vi "TF+NLH_2Dsweep.vi"() -> ()   [LabVIEW 2022 SP3]
uses:
  <vilib>/Analysis/baseanly.llb/Mean (DBL).vi
  <vilib>/Utility/file.llb/Write Delimited Spreadsheet (DBL).vi
  <vilib>/Analysis/NI_AALBase.lvlib
panel:
  out "Ri_2 phase":cluster{dbl[], dbl[]}(graph)={array[447 elements], [67.2863266033115, 68.42643229574017, 69.17560413533383, 69.48941864427059, 69.72823571868426, 69.93246230369206, 70.1751884099646, 70.29710903847356, 70.39938133386191, 70.53057955170597, 70.54955973974907, 70.65483370602274, 70.71576830766907, 70.74836693865872, 70.76726186359649, 70.82230290925978, 70.874667517587, 70.89353111410381, 70.91524850533594, 70.93619825305268, 70.95863943875658, 71.00402301767619, 71.02562315691524, 71.04364751898778, 71.09155969320202, 71.10466632875095, 71.10472623689654, 71.11327539933023, 71.12212675635854, 71.13448640937536, 71.13707018459343, 71.156029588503, 71.18142789627288, 71.18100597943726, 71.20627888034906, 71.2369698804632, 71.21647578693465, 71.22359731855786, 71.23619623503137, 71.23447865756799, 71.25487976993254, 71.25641101829986, 71.23187433810936, 71.26795744521557, 71.26926560819051, 71.2771926948209, 71.27014833338151, 71.29771757397829, 71.30132174890119, 71.3027753509576, 71.31013562290448, 71.3102375767113, 71.31479459935522, 71.31377012836376, 71.31067966990994, 71.32732871141567, 71.31983842896408, 71.32251344696019, 71.32521523529707, 71.32875354873806, 71.35240329133966, 71.32964637397781, 71.32891425163895, 71.33475814547418, 71.34060930371533, 71.34054473598107, 71.31731968477858, 71.34187116380903, 71.33824813020512, 71.3390204549954, 71.3291558641549, 71.33242973297482, 71.32654001657814, 71.3272617859802, 71.3232175453115, 71.32751642872424, 71.3248015822765, 71.31798187946346, 71.3225081113599, 71.29809468363369, 71.30757005126013, 71.31570116799156, 71.30739843616387, 71.29146920648236, 71.31124170405452, 71.29596584243514, 71.28527922227121, 71.28458810569983, 71.27687551520447, 71.28116342030664, 71.27141850884814, 71.25665249517958, 71.26071027298815, 71.24933212594051, 71.25573024107487, 71.23687214113531, 71.24357647122437, 71.22797873896852, 71.24152814258585, 71.24474907085207, 71.22697381112455, 71.19497244467797, 71.17889791182691, 71.18099382170517, 71.15694947879511, 71.17059403346802, 71.12873981748677, 71.1107641143075, 71.14403706999485, 71.09262969949951, 71.06730520589295, 71.0630662116972, 71.02272879938403, 71.01998987723536, 70.99742600032722, 70.95532207530876, 70.92773951911037, 70.91163496840906, 70.8723642026468, 70.8417266112045, 70.8181277661851, 70.78078830297738, 70.71770772291823, 70.64708869592285, 70.61065891810469, 70.54665253154197, 70.46814601200624, 70.3283370315843, 70.29477028786333, 70.12133548068076, 70.06168917206354, 69.71047188058449, 69.32322258598009, 69.00245607837441, 68.38129382500267, 63.32943082108405, 63.32943082108405]}
  out "Ri_1 phase":cluster{dbl[], dbl[]}(graph)={array[447 elements], [98.64824057353222, 99.17128830231329, 99.1951342832612, 99.00789207290453, 86.10182821595602, -22.857403054638922, 96.84732468296504, 95.16561698897686, 94.41179895625767, 93.19312788552409, 92.23293801802438, 91.48213679635391, 90.86975385450903, 90.08904401111859, 89.56708637967665, 89.05816339184628, 88.51699643736988, 88.00847910591001, 87.55358527129964, 86.9386521072525, 86.32661049392021, 85.97224810625127, 85.4201820241664, 84.76613324411304, 83.98328622688851, 82.62160554286582, 81.65949317710628, 81.06783279665753, 79.92401079184569, 79.42237386116088, 77.70119428653867, 76.70556650622181, 75.87256065512653, 74.17517588749186, 72.53499012614749, 70.99216973171393, 69.3270225882778, 67.65430069310983, 66.10158964613719, 64.57827117039957, 63.36900691986517, 61.856694114558294, 60.5780266856337, 58.9553710362398, 57.66899646954723, 56.46028015883566, 55.18644618742208, 53.89478474582762, 52.86893225941858, 51.90576740532828, 50.815840539479666, 49.83854583648395, 48.98783726797048, 48.20481920257575, 47.14323960132569, 46.56300379926881, 45.8424597787853, 45.104085421320164, 43.98778066206287, 43.55050208439842, 42.823698017347695, 42.208475197083224, 41.75023833211596, 41.006095441554294, 40.42414009253254, 39.92347465699966, 39.3026509483175, 38.70256301313423, 38.39814062530039, 39.08975991819877, 39.69244374540481, 40.39664196446022, 41.06014705097745, 41.5943514568138, 42.34629494787673, 42.80698579826661, 43.43303183920828, 44.19103885752135, 44.94458808485702, 45.81347646789879, 46.337237587140464, 47.157534614289126, 48.026176291338786, 48.910058096664116, 49.821788971793694, 50.620099538298255, 51.49220008891227, 52.576410576076526, 53.43639146612666, 54.795931099898326, 56.02887262919462, 57.22985495493462, 58.39636346943762, 60.06322069434742, 61.59991363454748, 63.227834999494156, 64.75529515969637, 66.40199391928505, 67.89160304574969, 69.41810595275406, 70.61294407010547, 72.26206019073916, 73.96623167454496, 74.87689970747078, 76.00422375609539, 77.31419973762613, 78.31609814928468, 79.07290556369516, 80.20713955144493, 81.345873616141, 82.42155295485148, 83.26995575330962, 84.0578825397184, 84.63979623611135, 85.34509922962876, 85.96512304224451, 86.47660709059683, 87.13813748614467, 87.65181081992219, 88.1985540120427, 88.44105847774664, 89.09342262415899, 89.37635655278324, 90.01954857540177, 90.8783427304726, 91.68597231772134, 92.80218889070814, 93.69238065841928, 95.01075372611008, 95.72905598293364, 71.98501757492694, 98.59740760348397, 98.99419919655249, 99.42747762755556, 99.12811502864284, 104.73224340549825, 118.33929590572768, 118.33929590572768]}
  out "Ri_2":cluster{dbl[], dbl[]}(graph)={array[447 elements], [15988.416286217624, 16728.6647819144, 17222.42749373977, 17463.498507260032, 17721.138199063775, 17863.57717963653, 17945.60163377109, 18070.197068356076, 18166.566932119193, 18199.668814845758, 18277.191037185512, 18350.597939893203, 18361.15003068617, 18538.192909865553, 18450.974040946323, 18496.93935775767, 18509.824502922875, 18528.92733421688, 18537.86973653712, 18247.33592210623, 18948.769873693338, 18615.781885697997, 18640.684401341037, 18645.991010057183, 18662.51527969985, 18677.117982566386, 18686.291050878437, 18723.39732314651, 18716.394342243046, 18745.923698774528, 18742.943040640737, 18753.840717426145, 18775.146084839842, 18775.625740218755, 18793.50624032839, 18791.928638182748, 18789.77689065863, 18803.77679848704, 18818.522370940067, 18811.440317156736, 18828.816055004674, 18833.01121266815, 18836.536471830892, 18842.43162267871, 18845.759082692643, 18855.340959944944, 18860.621985832437, 18874.850438323345, 18867.832627662334, 18873.199676166147, 18874.553160643718, 18877.146479793708, 18879.575606860988, 18890.63600339655, 18899.581042113925, 18907.506617494073, 18916.48206061786, 18918.81920186236, 18914.158596064004, 18938.10837688086, 18914.372066344815, 18923.82303003343, 18929.691680309785, 18941.758817006208, 18940.591605136684, 18976.56467259452, 18972.98156024733, 18965.48790428681, 19192.184240301955, 19190.22161257914, 19184.32494170946, 19192.81728878463, 19180.92951693814, 19179.037679145236, 19182.86767673744, 19178.918568569236, 19201.412480776875, 19341.87490145231, 19045.70581863397, 19204.205684223503, 19196.311769694086, 19199.806156914856, 19198.870165396227, 19206.399452576, 19204.64888696486, 19206.22900198729, 19211.355500785234, 19200.977734814664, 19217.406066104344, 19207.61978640744, 19204.203265191234, 19196.626056963243, 19213.181809880232, 19222.584678372026, 19214.73805057691, 19211.056701580124, 19227.966064572895, 19215.157961719193, 19228.694420225944, 19223.67013231585, 19234.181235717897, 19224.874809867804, 19179.32553225776, 19255.49825519169, 19244.876218524, 19264.41086650312, 19250.059516370784, 19265.408404384434, 19272.545589135265, 19280.416444140265, 19266.700590910965, 19241.253047333794, 19347.160839478965, 19374.179636748766, 19317.46815326459, 19397.194589803166, 19411.40251989236, 19457.002513082487, 19912.691099016047, 19043.806257533153, 19494.748229323617, 19516.780218679087, 19447.240330432873, 19579.68129130049, 19615.446193127405, 19659.245364140435, 19735.448787978745, 19815.406553193978, 19861.803283628833, 20009.699793679596, 20240.011056436713, 20342.30679666903, 20588.65312850611, 21006.842319071144, 21525.00085326132, 20433.789359112274, 20433.789359112274]}
  out "Ri_1":cluster{dbl[], dbl[]}(graph)={array[447 elements], [22045576.2714605, 27293475.908086587, 30763955.208301757, 33265764.692809474, 43359821.082717545, 3155950.3758325954, 33975645.41594882, 32879454.66260026, 31716318.00728969, 31039472.693512905, 29809111.33585218, 28574312.45520694, 27543957.107786126, 26496347.036176518, 25559561.38549122, 24548364.813615683, 23365812.88687177, 22124529.65451581, 21230854.097893827, 20210267.51082642, 19580261.477197297, 18912705.180425838, 18406731.282342993, 17712068.29371939, 17027409.310427506, 16451774.118448615, 15829444.291943796, 15233977.48645753, 14766262.770308785, 14332279.386885434, 13748323.747465877, 13302293.487016145, 12875564.13292509, 12323361.341903234, 11777348.54953025, 11284216.582856042, 10759787.6896821, 10352358.648472596, 9964767.14158643, 9552161.023707548, 9163674.14096663, 8774378.96453125, 8376817.067701741, 8100140.907855841, 7766189.394005965, 7453943.332151328, 7145119.814823653, 6822330.020409241, 6532919.550885053, 6345124.678109345, 6023202.797745062, 5790106.182555463, 5600133.754870802, 5372266.874572496, 5136954.451639774, 4961445.221169122, 4757697.428252076, 4596225.497057631, 4386501.247851164, 4248260.447246732, 4089296.5911337156, 3966429.9201004268, 3832855.939994699, 3717164.6148954397, 3590778.0316126416, 3454130.471709945, 3341234.1590903536, 3265289.764642522, 3297870.0581998965, 3413163.572910136, 3544001.8891905816, 3689443.812705478, 3799303.206259065, 3926721.983737788, 4086964.4365348606, 4206268.0769452825, 4324796.6500504315, 4532717.444204017, 4705136.3930503065, 4875754.054723214, 5071253.457257944, 5303339.599973234, 5481789.417311492, 5728974.215024379, 5943041.275664855, 6174939.548842898, 6419505.835430101, 6696129.679688083, 6980660.096420176, 7328131.387300405, 7608587.58451165, 7931731.115199456, 8263562.874033847, 8695880.524476495, 9124333.086620266, 9537334.492855161, 10001273.51709675, 10434185.413471175, 10904732.657212943, 11384488.704988042, 11790752.952395312, 12375155.659543715, 12874611.660482263, 13299920.063137745, 13680109.511602128, 14152552.783915121, 14646406.058544977, 15242436.55088634, 15838963.722419221, 16488066.171778262, 17189155.40604383, 17874112.959747944, 18505753.66220926, 19199799.29112946, 20082043.340339284, 20849920.713500258, 21637861.109894592, 22530184.096754618, 23696883.713339817, 24704796.36239602, 25871820.156915992, 26994576.58276976, 28599022.488043997, 29553699.907902468, 30925102.81800534, 32120594.843124736, 33923375.76541176, 35108063.55119341, 36833143.39217386, 37366688.458940916, 23545040.53535154, 41067758.729426846, 40939623.20198413, 39560091.29458222, 36752071.88798856, 14862918.294371193, 394331.9556378005, 394331.9556378005]}
  out "Device 2 phase":dbl=67.2863266033115 format="%.3p"
  out "Device 1 phase":dbl=98.64824057353222 format="%.3p"
  out "Ri_2(Ohm)":dbl=15988.416286217624
  out "Ri_1(Ohm)":dbl=22045576.2714605
  out "Device2 Current(mA)":dbl=8.369793490118766e-06
  out "Device1 Current(mA)":dbl=1.295038149901161e-06
  in  "R2(Kohm)":dbl=2.0 format="%#_13g"
  in  "R1(Kohm)":dbl=2.0 format="%#_13g"
  in  "R2 Sensitivity":u16(ring)=26 items=["1 nV/fA", "2 nV/fA", "5 nV/fA", "10 nV/fA", "20 nV/fA", "50 nV/fA", "100 nV/fA", "200 nV/fA", "500 nV/fA", "1 uV/pA", "2 uV/pA", "5 uV/pA", "10 uV/pA", "20 uV/pA", "50 uV/pA", "100 uV/pA", "200 uV/pA", "500 uV/pA", "1 mV/nA", "2 mV/nA", "5 mV/nA", "10 mV/nA", "20 mV/nA", "50 mV/nA", "100 mV/nA", "200 mV/nA", "500 mV/nA", "1 V/uA"]
  in  "R2 Current T Constant":u8(ring)=9 items=["10 us", "30 us", "100 us", "300 us", "1 ms", "3 ms", "10 ms", "30 ms", "100 ms", "300 ms", "1 s", "3 s", "10 s", "30 s", "100 s", "300 s", "1 ks", "3 ks"]
  in  "R1 Current T Constant":u8(ring)=9 items=["10 us", "30 us", "100 us", "300 us", "1 ms", "3 ms", "10 ms", "30 ms", "100 ms", "300 ms", "1 s", "3 s", "10 s", "30 s", "100 s", "300 s", "1 ks", "3 ks"]
  in  "R1 Current sensitivity":u16(ring)=26 items=["1 nV/fA", "2 nV/fA", "5 nV/fA", "10 nV/fA", "20 nV/fA", "50 nV/fA", "100 nV/fA", "200 nV/fA", "500 nV/fA", "1 uV/pA", "2 uV/pA", "5 uV/pA", "10 uV/pA", "20 uV/pA", "50 uV/pA", "100 uV/pA", "200 uV/pA", "500 uV/pA", "1 mV/nA", "2 mV/nA", "5 mV/nA", "10 mV/nA", "20 mV/nA", "50 mV/nA", "100 mV/nA", "200 mV/nA", "500 mV/nA", "1 V/uA"]
  in  "LOCKIN3 address":refnum<visa-resource-name>="COM5"
  in  "Current measurement?":bool=TRUE
  in  "Parameter 1B 1":u16(ring)=2 items=["X", "Y", "R", "Theta", "Frequency", "Noise", "Xh1", "Yh1", "Rh1", "Theta h1", "Xh2", "Yh2", "Rh2", "Theta h2"]
  in  "Phase 1B 1":u16(ring)=3 items=["X", "Y", "R", "Theta", "Frequency", "Noise", "Xh1", "Yh1", "Rh1", "Theta h1", "Xh2", "Yh2", "Rh2", "Theta h2"]
  out "Vab_1(1w)/mV":dbl=69.89491300035615
  out "phase Vab_1":dbl=90.88973926590094
  out "Vab_1/mV":cluster{dbl[], dbl[]}(graph)={array[447 elements], [69.89491300035615, 96.76091439179595, 121.60820325078673, 144.86984014112141, 167.73987501255314, 189.85333845062206, 212.76412267080005, 234.14803223340567, 254.28955060290502, 272.7317853345533, 289.83246203860267, 305.5450081707562, 320.16279403993354, 334.0773405165712, 347.02580142204937, 359.09399104540176, 372.23679318705814, 381.71894566566425, 396.5690488528649, 406.940835102248, 415.4777292621394, 424.8569017583363, 432.7538730200402, 440.00812513863, 448.52637063152594, 456.85237908909124, 464.137670276543, 472.2262412823993, 479.92842889273936, 487.6190417996467, 496.3166214468891, 503.07011002512405, 508.8219837590173, 517.1519063185144, 525.7953306380335, 539.3627686357203, 541.3617410482888, 548.5971674541836, 556.374844313196, 563.6069775945068, 571.8031649261083, 580.495799665217, 586.3877145229121, 593.8940166229253, 600.721090651385, 607.6895159228869, 614.1735521509668, 621.3512268861805, 628.0638510684262, 636.9440825992266, 642.589550225185, 649.9335791143177, 656.2448134788818, 663.9368277053549, 670.7937070923226, 678.5695123765853, 686.3987854950642, 694.5732517890214, 699.7779564487922, 705.685059941211, 713.0262385771273, 720.1108156834745, 729.569007775922, 735.0544079957034, 740.576008333156, 748.092243959333, 756.9633362654706, 760.2650973137223, 770.0898646046744, 763.2754854059085, 758.3002322895187, 746.9705677890544, 742.0331175764676, 735.46121484323, 727.7172172859215, 720.7173158772874, 712.99169073752, 707.050271699919, 699.916135108249, 694.4541828796475, 687.007963984917, 680.182322092647, 671.6050750240062, 665.5686279746279, 659.08553222554, 653.6017948895201, 646.4809963945931, 639.403394643278, 630.3579752688884, 623.5181112871613, 616.8554923220863, 610.6099012812795, 603.2215573569297, 595.4709115032604, 585.447913504759, 577.6229779091719, 570.5976464085383, 563.4007691158172, 555.4873986901947, 548.6413839458369, 540.585411112968, 532.6016369667757, 526.2399667657975, 518.0081516009911, 511.03829248244693, 502.0670977041706, 494.5727702095127, 488.0329979874539, 478.84273975168026, 471.69952058379425, 464.6428266619654, 455.7501857674969, 447.6210647470701, 440.1493478794361, 431.08806792417124, 421.6336738249846, 411.80987033576866, 403.49332406392034, 393.617268025408, 383.21282480148824, 372.20708655208506, 360.5170780717179, 348.99573641712726, 336.0751062717885, 322.3016839152484, 307.1083537103844, 290.94530748218335, 273.55902036869213, 254.4926943267793, 234.28942783781397, 212.9781220107684, 187.86427671847667, 165.2636595766354, 142.77665596194007, 119.793615425549, 95.38271597000687, 0.09538271597000687]}
  out "phase Vab_1":cluster{dbl[], dbl[]}(graph)={array[447 elements], [90.88973926590094, 90.52797326935718, 90.24221168935227, 90.05619331418181, 89.82402670735155, 89.43475667628768, 88.97990454089964, 88.44396332463643, 87.96488659679174, 87.42119770073006, 86.92388263342272, 86.48364998536113, 85.99122029778825, 85.57113746974912, 85.1737392935055, 84.84429176826526, 84.61648244558981, 84.39863700541643, 84.39047173551977, 84.31040018808953, 84.28616173042795, 84.27963444410904, 84.29052508971986, 84.35337905461374, 84.48798685578761, 84.6334468365483, 84.84938888426412, 85.05553183037861, 85.2218152401819, 85.40541095682514, 85.66046178789543, 85.90545188370128, 86.13216922565734, 86.38265558116399, 86.65406276846046, 86.91253207804952, 87.18486426305384, 87.42816773898326, 87.63158481854084, 87.86233637683861, 88.13407094246728, 88.27976493605578, 88.57655203525272, 88.82933322275144, 89.06438112269504, 89.29707773628597, 89.50407685721082, 89.74107738483386, 89.89143188530203, 90.06691792993078, 90.3103543154843, 90.46367936659934, 90.6387057493134, 90.82986512108896, 91.01674618887878, 91.09084887196157, 91.27133334734977, 91.40474871037804, 91.52644294089797, 91.67243711695147, 91.77582850460796, 91.93779407688712, 91.96007834595751, 92.15572215870259, 92.29971314770144, 92.3387174294799, 92.42238251137285, 92.62272966378458, 92.59121603701458, 92.52667962397057, 92.37812039104159, 92.41197917214927, 92.25218709944694, 92.13367167192551, 92.04888515402025, 91.9110871959863, 91.79252598732182, 91.60650423258802, 91.59890708517739, 91.40387946715751, 91.21488009806522, 91.11358490554794, 90.99524149204582, 90.79975373157988, 90.62251592150207, 90.45192948011531, 90.27266294152018, 90.08071301381186, 89.92199803936612, 89.66090401141147, 89.48436778178451, 89.24229483637853, 88.99995082200304, 88.80450846419185, 88.63063132266655, 88.3773911659327, 88.11024296250065, 87.90048336420998, 87.63874656677974, 87.40922433762555, 87.15146501518254, 86.86078212535051, 86.6538901112055, 86.41540121139467, 86.20189760315316, 85.9426657982776, 85.690292850898, 85.43151419868113, 85.2197061571944, 85.01429203463259, 84.84078565202971, 84.65834064339072, 84.50978131286871, 84.38968861773391, 84.27730864450257, 84.19167192359482, 84.15599911428015, 84.24936497822945, 84.29514042933667, 84.4229792596429, 84.61642660479922, 84.87595078760202, 85.23931108593368, 85.62649020269703, 86.06934732659286, 86.55060906452294, 87.03428962580335, 87.51819781702497, 88.06917931477217, 88.5245583671414, 88.98978203472014, 89.44122721966406, 89.75358671473366, 90.00839348446064, 90.21871142933574, 90.46727689558784, 90.46727689558784]}
  out "Vab_2(1w)/mV":dbl=0.05504782589540923
  in  "Parameter 2B 1":u16(ring)=2 items=["X", "Y", "R", "Theta", "Frequency", "Noise", "Xh1", "Yh1", "Rh1", "Theta h1", "Xh2", "Yh2", "Rh2", "Theta h2"]
  in  "Phase 2B 1":u16(ring)=3 items=["X", "Y", "R", "Theta", "Frequency", "Noise", "Xh1", "Yh1", "Rh1", "Theta h1", "Xh2", "Yh2", "Rh2", "Theta h2"]
  out "Vab_2/mV":cluster{dbl[], dbl[]}(graph)={array[447 elements], [0.05504782589540923, 0.08174963900387706, 0.1086491390142213, 0.1350953352313944, 0.16199632000588896, 0.18871077141583378, 0.21540521495658613, 0.24212435453052203, 0.26890247886877494, 0.29552482456320167, 0.32258570821668, 0.3494042559717882, 0.37594130906440903, 0.40415399166191385, 0.4297877956839886, 0.4565469885788846, 0.4834868719058818, 0.5099801395541058, 0.5365898114212174, 0.5650196727768638, 0.6153224681040677, 0.6167753495606371, 0.6433511284852396, 0.6698553439971563, 0.6963334815374641, 0.72306249630336, 0.7498661407570503, 0.777540387307819, 0.8039872881129053, 0.8306848892073286, 0.8565751828914451, 0.8836807612900971, 0.9105318047943302, 0.936516650845644, 0.9636848031511576, 0.9900174496688153, 1.0155067100535131, 1.0429079201232776, 1.069429262326823, 1.0956882570263036, 1.1222110190156476, 1.148795646772743, 1.1753327010150363, 1.2019263533143982, 1.228381719823452, 1.2545475198538012, 1.2812633241442646, 1.3070782706694737, 1.333608439591284, 1.3600906687552823, 1.3862774538793732, 1.412061455838872, 1.4389670903805294, 1.4651948591598645, 1.4908718427837173, 1.518015543331282, 1.545769299778577, 1.572154931730819, 1.5985003001796778, 1.6233111449201556, 1.6484992142095583, 1.6747983901681438, 1.7020924335968, 1.7287579367019952, 1.7559499387410313, 1.782575600183194, 1.8090046681914527, 1.8359466301397063, 1.8586719383176984, 1.8319060664677964, 1.8059980427635538, 1.7796862395299262, 1.7514192762034468, 1.7244809548743052, 1.6983410974939976, 1.6718938419879956, 1.6462121209020237, 1.6195000852062709, 1.5674352448786275, 1.5688527907635799, 1.5421352110091182, 1.5166894409291403, 1.4901521893311171, 1.463685618446582, 1.4371269782596554, 1.4108838829627208, 1.3845821412725943, 1.3582753758079424, 1.3321639978967672, 1.3046348516956425, 1.2784296961198498, 1.251377246196452, 1.2257446823466882, 1.199624176714759, 1.1726915378017204, 1.1462270638572194, 1.11975842382519, 1.0933051178522766, 1.0670212956767868, 1.0400481080390023, 1.0136730950163222, 0.9865872713125264, 0.9595089165754551, 0.9333819228541328, 0.9067272830452382, 0.8800918508692932, 0.8531109540697044, 0.8272638966110974, 0.8002139272602338, 0.77334067720438, 0.7464596577055119, 0.720085145608187, 0.6941845834379488, 0.6705341882933702, 0.6438603276504212, 0.617016475397683, 0.5899056969248984, 0.5631586418589446, 0.535158502041674, 0.4850978602391158, 0.48255405943119034, 0.4553320577540521, 0.42723377189680495, 0.4011445572614489, 0.3744925824568009, 0.3473094083332051, 0.32092465247254065, 0.2938313088100053, 0.2671169874808368, 0.2403177493052949, 0.21367423121897425, 0.18666841954924793, 0.1596474534235999, 0.13259816185629864, 0.10564756137259422, 0.10564756137259422]}
  out "phase Vab_2":dbl=89.98636954382417
  out "phase Vab_2":cluster{dbl[], dbl[]}(graph)={array[447 elements], [89.98636954382417, 90.03967319419863, 90.0401476465123, 89.99776761885384, 90.0222418709453, 90.01526903166591, 90.02869426514728, 90.01475132450953, 90.02160015273246, 90.03106270083825, 90.03582546833678, 90.03257710652228, 90.02612755809257, 90.02777418011617, 90.02881201881874, 90.02603115955061, 90.03387858321058, 90.02423111026776, 90.0298329743401, 90.0199101721892, 90.02008626238324, 90.01905833125883, 90.0226624250662, 90.01524219410577, 90.01064477190369, 90.01314320313155, 90.00964441150451, 90.007480576353, 90.00751384955382, 90.00568040647654, 90.00225023080912, 90.00179313839485, 89.9943445053494, 89.99638341896197, 89.99107879178376, 89.99070351224353, 89.98795446635322, 89.98662682800266, 89.98255898571668, 89.97950944534594, 89.97885050000609, 89.98001159100461, 89.97638179460355, 89.97397388097008, 89.97386998434929, 89.97190686780083, 89.96964943942537, 89.96652965395793, 89.96664790872887, 89.9651967818322, 89.96328286683708, 89.96390175771866, 89.9603252973263, 89.95814083102191, 89.95867001681638, 89.95859246077052, 89.9599408176306, 89.9554627877762, 89.9563396626164, 89.9542344080695, 89.9537832379153, 89.95103282620559, 89.95050590087968, 89.95106030902204, 89.95264289581421, 89.95158819964809, 89.95041962543326, 89.94974338020069, 89.94997443777854, 89.95170075918911, 89.95247909300647, 89.95180399748936, 89.94841578255253, 89.9503050525758, 89.95385182971656, 89.95377247032924, 89.95406599067066, 89.96047202514728, 89.95820512566924, 89.95880560309685, 89.95764180403465, 89.96186623373474, 89.96308076069838, 89.96241158857234, 89.96358286171663, 89.96555096814687, 89.96414990686654, 89.96805952212296, 89.96805956444439, 89.96842578734393, 89.97234710687766, 89.97321477774166, 89.97532264688338, 89.97725566537538, 89.98119721498324, 89.97774793328412, 89.98176413337141, 89.9856479020747, 89.98484345999856, 89.98795891683308, 89.98813178811233, 89.98795432168693, 89.98952215489766, 89.99420384702498, 89.99647060182336, 89.99526917518443, 89.99933379690103, 90.00609885406311, 90.00482328009898, 90.00861804999309, 90.01263720244857, 90.01011885735718, 90.01426821869731, 90.01434477063428, 90.02407380002145, 90.01888273544807, 90.02104556140974, 90.02226692616459, 90.0184250982925, 90.02624472279317, 90.03191794705317, 90.02551643212949, 90.02854738363274, 90.02816141702668, 90.02924202432983, 90.0225129073069, 90.03393763571692, 90.02461542837548, 90.02201842331168, 90.02883400042535, 90.0149527060912, 90.03276532522105, 90.03417556063343, 90.00596720794834, 89.99433316143694, 89.99433316143694]}
  out "Phase2A-F":cluster{dbl[], dbl[]}(graph)={[0.1], [0.0]}
  out "R2A-F":cluster{dbl[], dbl[]}(graph)={[0.1], [0.0]}
  out "Phase2B-F":cluster{dbl[], dbl[]}(graph)
  out "R2B-F":cluster{dbl[], dbl[]}(graph)={[0.1], [0.0]}
  out "phase 2B 2":dbl
  in  "Phase 2B 2":u16(ring)=9 items=["X", "Y", "R", "Theta", "Frequency", "Noise", "Xh1", "Yh1", "Rh1", "Theta h1", "Xh2", "Yh2", "Rh2", "Theta h2"]
  out "phase 2A 2":dbl
  in  "Phase 2A  2":u16(ring)=3 items=["X", "Y", "R", "Theta", "Frequency", "Noise", "Xh1", "Yh1", "Rh1", "Theta h1", "Xh2", "Yh2", "Rh2", "Theta h2"]
  out "para2A Measurement 2":dbl
  in  "F Clear Plot 2A":bool
  in  "Parameter 2A 2":u16(ring)=2 items=["X", "Y", "R", "Theta", "Frequency", "Noise", "Xh1", "Yh1", "Rh1", "Theta h1", "Xh2", "Yh2", "Rh2", "Theta h2"]
  out "para2B Measurement 2":dbl
  in  "F Clear Plot 2B":bool
  in  "Parameter 2B 2":u16(ring)=8 items=["X", "Y", "R", "Theta", "Frequency", "Noise", "Xh1", "Yh1", "Rh1", "Theta h1", "Xh2", "Yh2", "Rh2", "Theta h2"]
  out "Phase1A-F":cluster{dbl[], dbl[]}(graph)
  out "R1A-F":cluster{dbl[], dbl[]}(graph)
  out "Phase1B-F":cluster{dbl[], dbl[]}(graph)
  out "R1B-F":cluster{dbl[], dbl[]}(graph)
  out "phase 1B 2":dbl
  in  "Phase 1B 2":u16(ring)=9 items=["X", "Y", "R", "Theta", "Frequency", "Noise", "Xh1", "Yh1", "Rh1", "Theta h1", "Xh2", "Yh2", "Rh2", "Theta h2"]
  out "phase 1A 2":dbl
  in  "Phase 1A 2":u16(ring)=3 items=["X", "Y", "R", "Theta", "Frequency", "Noise", "Xh1", "Yh1", "Rh1", "Theta h1", "Xh2", "Yh2", "Rh2", "Theta h2"]
  out "para1A Measurement (mV) 2":dbl=1.49013e-07
  in  "F Clear Plot 1A":bool
  in  "Parameter 1A 2":u16(ring)=2 items=["X", "Y", "R", "Theta", "Frequency", "Noise", "Xh1", "Yh1", "Rh1", "Theta h1", "Xh2", "Yh2", "Rh2", "Theta h2"]
  out "para1B Measurement (uV) 2":dbl=1.49013e-07
  in  "F Clear Plot 1B":bool
  in  "Parameter 1B 2":u16(ring)=8 items=["X", "Y", "R", "Theta", "Frequency", "Noise", "Xh1", "Yh1", "Rh1", "Theta h1", "Xh2", "Yh2", "Rh2", "Theta h2"]
  in  "path2 (folder + filename)":string="H:\\My Drive\\Lab\\Opticool\\Measurement\\NLH\\T dependence\\TaI27_A1016_B1516_test"
  out "phase Vaa_1":cluster{dbl[], dbl[]}(graph)={array[447 elements], [-90.0, -90.0, -90.0, -90.0, -90.0, -90.0, -90.0, -90.0, -90.0, -90.0, -90.0, -90.0, -90.0, -90.0, -90.0, -90.0, -90.0, -90.0, -90.0, -90.0, -90.0, -90.0, -90.0, -90.0, -90.0, -90.0, -90.0, -90.0, -90.0, -90.0, -90.0, -90.0, -90.0, -90.0, -90.0, -90.0, -90.0, -90.0, -90.0, -90.0, -90.0, -90.0, -90.0, -90.0, -90.0, -90.0, -90.0, -90.0, -90.0, -90.0, -90.0, -90.0, -90.0, -90.0, -90.0, -90.0, -90.0, -90.0, -90.0, -90.0, -90.0, -90.0, -90.0, -90.0, -90.0, -90.0, -90.0, -90.0, -90.0, -90.0, -90.0, -90.0, -90.0, -90.0, -90.0, -90.0, -90.0, -90.0, -90.0, -90.0, -90.0, -90.0, -90.0, -90.0, -90.0, -90.0, -90.0, -90.0, -90.0, -90.0, -90.0, -90.0, -90.0, -90.0, -90.0, -90.0, -90.0, -90.0, -90.0, -90.0, -90.0, -90.0, -90.0, -90.0, -90.0, -90.0, -90.0, -90.0, -90.0, -90.0, -90.0, -90.0, -90.0, -90.0, -90.0, -90.0, -90.0, -90.0, -90.0, -90.0, -90.0, -90.0, -90.0, -90.0, -90.0, -90.0, -90.0, -90.0, -90.0, -90.0, -90.0, -90.0, -90.0, -90.0, -90.0, -90.0, -90.0, -90.0]}
  out "Vaa_1/mV":cluster{dbl[], dbl[]}(graph)={array[447 elements], [28.54986230809714, 47.90602322555852, 69.13880402618318, 91.74088027854695, 116.09423060900622, 126.29292594886878, 152.34333138764072, 170.38941026837637, 188.72717003139223, 207.09670879518862, 223.27714792302223, 239.09530915982268, 253.96866223624244, 268.10055850834317, 284.1930208945555, 296.9400604656871, 306.8418650583954, 314.71077986113585, 324.8096514364511, 334.45516719840055, 345.2751932124764, 355.7157880621078, 366.8537803090993, 375.6147659337272, 382.6007505803814, 393.47724926935217, 400.49050064772996, 407.5485504924969, 413.6432604376539, 420.8265461237909, 426.6173764310682, 433.635430137789, 442.5451386667651, 446.83506923110616, 449.41691810343707, 455.1160806660415, 459.5157780704797, 464.5304454573484, 471.2973043505908, 475.2198625165156, 479.07227226723137, 482.9178917074458, 486.22088193879244, 495.09103303765596, 499.324083426905, 504.20168302074853, 509.45597042076264, 512.0104443681062, 513.8593456505303, 521.857561920325, 521.7846572347574, 524.8188626940346, 530.7443300930335, 532.2284129403052, 536.4970249271563, 538.859316009316, 541.4792257221472, 546.466260110555, 551.0869260849482, 552.4833138837979, 555.8760860627742, 557.6075820251485, 559.767692284389, 565.4670612075352, 567.1402355116674, 568.4045720496342, 571.3865971710253, 578.6325276470443, 576.7201061295497, 571.1883361841326, 570.4182884439209, 569.461761245208, 565.2512639499868, 562.3052339123483, 560.6884611622394, 558.9193285846687, 553.1436266827282, 551.5932911338228, 548.635799671936, 542.1674835477035, 541.0172163291315, 539.914220429268, 533.6419081222197, 531.0176781462837, 525.3084038907192, 522.7943427328461, 518.5380642635973, 515.8961486976631, 514.2733852885369, 509.72759631064423, 503.9501781756484, 499.2678347371449, 496.40962237161796, 491.80635505697677, 490.4617117070987, 485.1742271220353, 482.0446129719921, 475.9996837404127, 472.6782621100959, 468.2971762724189, 462.1864679849175, 458.47754471745617, 450.5194671600685, 445.05833394151387, 437.3036576834162, 429.75676530040477, 422.2152681826013, 416.86776209046945, 410.4010237044718, 403.16700771496164, 396.8216458438753, 388.49299645581715, 380.56332239470265, 372.3807562243823, 361.6392938119466, 355.2142501054603, 344.4659622791879, 333.32240957381543, 323.4493356975189, 312.13865046326316, 300.50315760800555, 286.86993382755776, 275.8465837513604, 258.6568970790021, 241.15871978639944, 227.792037293373, 211.3465846844987, 195.5210307298651, 179.12175652769412, 160.0385725885352, 150.4506723637251, 123.84923542089372, 103.1763424845562, 80.07139246418663, 57.276443385142485, 36.166077095315934, 17.42622501409195, 17.42622501409195]}
  out "Phase1B-T":cluster{dbl[], dbl[]}(graph)={array[447 elements], [-0.0428368767358694, 0.019425738673648576, 0.06601336294885965, 0.12751390529792714, 0.21891328703140842, 0.2139600423089886, 0.3202891373518463, 0.5653445808746654, 0.8962538707982652, 1.2571346321505499, 1.606301670176481, 1.9056143928649256, 1.991351868000408, 1.988260247302692, 1.755701270770857, 1.4150419758773847, 0.9666181709825361, 0.4781661851611167, 0.07786977428258289, -0.31921775054521556, -0.5319269967389744, -0.917697368480033, -1.416396561722631, -1.6500153972582816, -1.9572642672945826, -2.2544114467295797, -2.162541178826363, -2.378638843933177, -2.7944233559771234, -2.9522321795232656, -3.073536918287995, -3.1242675115899687, -3.0838196681594883, -3.5508253393225524, -3.8243520103554154, -3.9039948394823236, -3.705890346352678, -4.021095031312841, -4.142208186339788, -4.557849167991822, -4.69334843822529, -4.98064985720908, -5.141308179691781, -5.597455016446071, -5.6045044083128195, -5.890565984116882, -6.487479059224005, -6.648445444092485, -6.7025474266406535, -6.807549291485394, -6.890715596724121, -6.670677922609039, -7.1779161834435525, -7.397104646423365, -7.725977915533429, -9.028821811181647, -9.625827157282213, -10.551010326623167, -10.140345055790643, -9.719127290466453, -9.455249331621122, -9.002043477711032, -8.812633517143642, -8.001995584354216, -6.796618229609791, -6.506804750288498, -5.384613593618006, -4.999091183121753, -4.671119395457472, -4.995028651891374, -5.163198702989056, -5.2275892583156764, -5.553112626699551, -5.742012236238783, -6.002884347788617, -6.34951264021017, -6.501343380041442, -6.996016601650247, -6.885713785862563, -6.808189214852123, -6.891739474989711, -6.414914544932198, -6.6107298401261305, -6.666545643649042, -6.669317377611124, -6.803630786969256, -6.687625686618477, -6.229020650697875, -6.5754921415814, -6.434215291472372, -6.178441867090024, -6.148668612211155, -5.855063552961937, -5.641145351326709, -5.407002479193986, -5.175085704554695, -4.984151429330852, -4.740938590426882, -4.393567047411585, -4.125555149902717, -3.9232596961522432, -3.58122053632991, -3.55297978358587, -3.012480741093095, -2.961273786915813, -2.17265758603968, -2.0218915507952593, -1.872085515945707, -1.6814909435522, -1.5599782037249579, -1.4112374104641112, -1.2382170209936327, -1.0671702138186363, -0.740217543128334, -0.6352820647843831, -0.36943879373102734, -0.16661703603105704, -0.02775688194834209, 0.12209464743594815, 0.27578697463604673, 0.44353680360386927, 0.5855139758919539, 0.6691109238405835, 0.7293740437580607, 0.7454861201352151, 0.7097541743895233, 0.6348587589201704, 0.5050228954104379, 0.3837962630215416, 0.23928951289350775, 0.4048700099789791, 0.2969667660401464, 0.2419093507799051, 0.15724973554986582, 0.07803063399563674, 0.03971435353920284, 0.03971435353920284]}
  out "R1B-T":cluster{dbl[], dbl[]}(graph)={array[447 elements], [156653.03630696764, 148669.35859716916, 140750.0698084012, 132895.51710122655, 125358.74665741803, 117251.34041918642, 110126.05537967787, 104032.3796825124, 98694.84438965151, 93627.06160482153, 88874.08330738443, 84651.96247295255, 80655.62889130137, 77353.36648383504, 74364.1231804382, 71537.43674065488, 69358.97439512891, 67633.51892577752, 66810.86995199334, 66456.55828298542, 66096.12665938094, 65862.08981586057, 65831.94755910935, 65938.78834732961, 66064.27762077464, 65323.83051235899, 64939.17778834897, 64592.35089393325, 64320.54559203627, 63927.50238148678, 63685.4736398772, 62952.941632842456, 61863.71621556276, 60968.37722476152, 60230.47573671074, 60493.40833415097, 60188.09201001243, 59886.193502477945, 59665.2220993736, 59463.7849048051, 59499.745510583736, 59594.69145722589, 59646.58712569106, 59775.211553687855, 59922.61732820779, 60037.32436687335, 59796.209859831164, 59396.04823648047, 59077.798079345455, 59005.77481987122, 58899.62037777882, 58549.59949712524, 57296.55847069468, 55185.31877347994, 52434.76696388336, 49244.170987330435, 45614.190254019355, 42447.2433009042, 40166.66109099554, 39992.14976412257, 40580.392421616554, 41558.88836278036, 43693.48991513804, 46625.649281395774, 49688.994850098374, 53044.280697961374, 55723.281474167954, 57636.31181556067, 57615.52406975564, 57520.638046988526, 57448.45745580508, 57767.61595961488, 57652.01666564756, 57527.643047949015, 57548.26764858691, 58046.55680219043, 58688.139202819584, 59519.35386512262, 60156.35189802062, 60345.93454513358, 60854.62397351101, 61566.06525510755, 62715.45636752421, 63851.76867791205, 64485.88190095292, 64583.8900715666, 64614.7318290972, 64616.22804455587, 65019.35744354623, 65159.95720882481, 65238.57114716061, 65026.68356980856, 64746.407251066936, 64664.484449826756, 64999.380726995165, 65462.789162605935, 65755.6101803984, 66133.51813389454, 66634.81383937939, 67166.7870458519, 68036.55322059919, 69027.86485769883, 70048.14565665925, 71368.20869162361, 72949.53106005031, 74835.45795357773, 76722.40627798814, 79199.53379772593, 82330.04244523244, 85827.64570941599, 89933.38874289654, 94673.33307932099, 100195.65823507162, 106491.45500187187, 113728.49713083068, 121616.58437941017, 130081.97029892445, 138723.70753480514, 148021.39689669872, 157968.65499305708, 167699.95173412305, 177664.07084666408, 184374.81286493735, 189183.163541887, 191512.30730552098, 191188.05610214468, 187927.49166520472, 180376.339012124, 168716.50294927045, 154922.70062195673, 138205.33167340915, 121320.09824131276, 104575.51507388374, 88622.86788988147, 75489.54929101207, 68245.72466796775, 68245.72466796775]}
  out "phase 1B":dbl=-0.0428368767358694
  in  "Phase 1B":u16(ring)=9 items=["X", "Y", "R", "Theta", "Frequency", "Noise", "Xh1", "Yh1", "Rh1", "Theta h1", "Xh2", "Yh2", "Rh2", "Theta h2"]
  out "phase Vaa_1":dbl=-90.0
  in  "Phase 1A":u16(ring)=3 items=["X", "Y", "R", "Theta", "Frequency", "Noise", "Xh1", "Yh1", "Rh1", "Theta h1", "Xh2", "Yh2", "Rh2", "Theta h2"]
  out "Vaa_1(1w)/mV":dbl=28.54986230809714
  in  "T Clear Plot 1A":bool
  in  "Parameter 1A":u16(ring)=2 items=["X", "Y", "R", "Theta", "Frequency", "Noise", "Xh1", "Yh1", "Rh1", "Theta h1", "Xh2", "Yh2", "Rh2", "Theta h2"]
  out "para1B Measurement":dbl=156653.03630696764
  in  "T Clear Plot 1B":bool
  in  "Parameter 1B":u16(ring)=8 items=["X", "Y", "R", "Theta", "Frequency", "Noise", "Xh1", "Yh1", "Rh1", "Theta h1", "Xh2", "Yh2", "Rh2", "Theta h2"]
  out "phase Vaa_2":cluster{dbl[], dbl[]}(graph)={array[447 elements], [90.0, 90.0, 90.0, 90.0, 90.0, 90.0, 90.0, 90.0, 90.0, 90.0, 90.0, 90.0, 90.0, 90.0, 90.0, 90.0, 90.0, 90.0, 90.0, 90.0, 90.0, 90.0, 90.0, 90.0, 90.0, 90.0, 90.0, 90.0, 90.0, 90.0, 90.0, 90.0, 90.0, 90.0, 90.0, 90.0, 90.0, 90.0, 90.0, 90.0, 90.0, 90.0, 90.0, 90.0, 90.0, 90.0, 90.0, 90.0, 90.0, 90.0, 90.0, 90.0, 90.0, 90.0, 90.0, 90.0, 90.0, 90.0, 90.0, 90.0, 90.0, 90.0, 90.0, 90.0, 90.0, 90.0, 90.0, 90.0, 90.0, 90.0, 90.0, 90.0, 90.0, 90.0, 90.0, 90.0, 90.0, 90.0, 90.0, 90.0, 90.0, 90.0, 90.0, 90.0, 90.0, 90.0, 90.0, 90.0, 90.0, 90.0, 90.0, 90.0, 90.0, 90.0, 90.0, 90.0, 90.0, 90.0, 90.0, 90.0, 90.0, 90.0, 90.0, 90.0, 90.0, 90.0, 90.0, 90.0, 90.0, 90.0, 90.0, 90.0, 90.0, 90.0, 90.0, 90.0, 90.0, 90.0, 90.0, 90.0, 90.0, 90.0, 90.0, 90.0, 90.0, 90.0, 90.0, 90.0, 90.0, 90.0, 90.0, 90.0, 90.0, 90.0, 90.0, 90.0]}
  out "Vaa_2/mV":cluster{dbl[], dbl[]}(graph)={array[447 elements], [0.13381974254969312, 0.18742714557336168, 0.24193630688555348, 0.2935892785474931, 0.3479241671469837, 0.40180896386790493, 0.45368862257203035, 0.5082025450648269, 0.5617588973183396, 0.6130105235675594, 0.6681572310006635, 0.7227895287602891, 0.7736466036357633, 0.8335500758536397, 0.8815480547811793, 0.9357109191098203, 0.9875782277032862, 1.040868809441492, 1.095090897331736, 1.1747106159712257, 1.226856272234, 1.2540223708132843, 1.308791730226083, 1.3601778715290997, 1.4144756362080564, 1.4669111879869992, 1.5198122641709386, 1.5763564964287788, 1.627258918430943, 1.6829610709942446, 1.7347039042428267, 1.787131627051539, 1.842990828060025, 1.8948913764748603, 1.9499228164526228, 2.0017844440101387, 2.0532826238944915, 2.109197084129517, 2.1629586294805323, 2.2144151171419972, 2.2692987490718153, 2.322005989452896, 2.3740937894622642, 2.4282075783401544, 2.48027388623933, 2.5346829265701496, 2.5886897937084234, 2.643246419254771, 2.693911762161861, 2.748627308177585, 2.801110037277913, 2.8529923664874692, 2.9056809189103614, 2.9607146118620182, 3.015233207723972, 3.068486923290655, 3.1234203943636327, 3.1755679448464025, 3.2287947853467114, 3.284263127783291, 3.333983892472329, 3.3877660463472044, 3.4425367018738493, 3.4976986613730205, 3.5487949460745205, 3.609858553422258, 3.6611429843509202, 3.710602935938376, 3.707057741181432, 3.652440365901994, 3.598528318933693, 3.547133036416897, 3.491914000109365, 3.436654890996338, 3.38373777826206, 3.3289956981589874, 3.279244940684171, 3.1929766105427855, 3.144399429486219, 3.1199998023843234, 3.064956277223548, 3.011777093344942, 2.958733588137276, 2.9073826220408523, 2.8529486049233252, 2.799604745203765, 2.7462382732359663, 2.6907286153414556, 2.6399129053163444, 2.5839375773906603, 2.529941329570786, 2.475965439824034, 2.4253889243156443, 2.37271574046373, 2.317295557052546, 2.2642061200665595, 2.2125103836347613, 2.1562554502299545, 2.1051508641724936, 2.050677472623137, 1.9979216366039663, 1.942572819238161, 1.8854172013620933, 1.8394191546832923, 1.7839892210108856, 1.7305228805087955, 1.6757577630299372, 1.6246239862471612, 1.5719471607187463, 1.517782524650135, 1.46244227108224, 1.4077807390939265, 1.3609587826472371, 1.307813032382216, 1.2515421511312934, 1.2020571451792048, 1.1476637017173545, 1.095545763835169, 1.0179772081249736, 0.9631381585880434, 0.9334695619404194, 0.8794155178512697, 0.8227043347953057, 0.7727602458939524, 0.7184672676003201, 0.6655627507727929, 0.6135075057219885, 0.5601076930051849, 0.5050556179993441, 0.4543692162049564, 0.40185237548020547, 0.34633302986717796, 0.2909740598878531, 0.23867838334778513, 0.18388695194469842, 0.18388695194469842]}
  out "Phase2B-T":cluster{dbl[], dbl[]}(graph)={array[447 elements], [-0.03469454178376795, -0.00736809463286604, -0.022964586979785772, -0.029719841307236955, -0.012534923664164779, -0.024046608840346307, -0.022023733182412193, -0.03259843425226211, 0.009789315130899187, -0.019231697327260287, -0.00197076413704439, -0.0009456659113533516, 0.021598458359082032, -0.00413298679003386, 0.011347317585862665, -0.005489815159564186, -0.0014322184820076947, 0.008701249063545564, -0.0007863262108556386, 0.040937815111443836, 0.014917465084632426, 0.016230414199592022, 0.015825143776374527, -0.004238768141281416, -0.01051382589652682, 0.009920733281610564, 0.010710247783674309, 0.023230377031032846, 0.017171097526619862, 0.011395695367618117, 0.029813815765387212, 0.012898568093394203, 0.032448247847814984, 0.03562701536157138, 0.009907229898713375, 0.04977618254559889, 0.061536323763389945, 0.055873059364917675, 0.02380492475396696, 0.03625374373044442, 0.03430519448445, 0.06277510794547422, 0.07897375762787914, 0.08752807527088088, 0.08402221704419507, 0.08973991309346498, 0.0868690267598029, 0.13339273780823613, 0.09958950773923789, 0.1319588742982189, 0.11200284605761765, 0.15173873916779504, 0.16735786090412777, 0.15229026460267883, 0.22884208641750078, 0.23233864824972522, 0.23085021357532587, 0.33335493111798997, 0.326747996257691, 0.35480709937030613, 0.4086867273386582, 0.48624541016539424, 0.3986964971024789, 0.4539889628130613, 0.4112947951309035, 0.36204948261250963, 0.37742637398489504, 0.42856724709625676, 0.4055333230141495, 0.3897500925288805, 0.3912548203211305, 0.3629025185492264, 0.32524440217378214, 0.3266906651948484, 0.30773861022717164, 0.25136721891928404, 0.24350155530653952, 0.2074197884324378, 0.20756072404172934, 0.20676220168454867, 0.19175260402444544, 0.1844711791087847, 0.13579375665250842, 0.15673231630620288, 0.11178794068160332, 0.14232205084844235, 0.11318497393618447, 0.1178655751936033, 0.09750899228105897, 0.09598622265035975, 0.07968677068785954, 0.062103901546804154, 0.06468685358155588, 0.07130268220684274, 0.07367927757035928, 0.044940632348484826, 0.04322308683449492, 0.05928277999632499, 0.024978464527785058, 0.03750346734159589, 0.030685547811318513, 0.018566627851074075, 0.03964375522641834, 0.004305476282311017, 0.010646690472283877, 0.008912045909642622, 0.017865981871776022, -0.0008468168685072223, 0.003932436303019588, 0.0009799036396718466, 0.03471865296441348, 0.017131373755713237, 0.005703705814645815, 0.007878891259521884, 0.032421741276479184, 0.010287942075355511, 0.02494364696719114, -0.007668201026975579, 0.02259238992163588, 0.0024294858061123647, -0.020071333366863748, 0.00913976669873675, 0.017212947020931714, -0.0033978822633656614, 0.012212676978409043, -0.01377040034799221, -0.030083462210506257, 0.004873300030023296, -0.023080036016378157, -0.007736338791769626, 0.022416006023880913, -0.05293149222077768, 0.005589169575936739, -0.09292022719030579, -0.04906017162668733, -0.04906017162668733]}
  out "R2B-T":cluster{dbl[], dbl[]}(graph)={array[447 elements], [224.31020276269777, 224.60377548201282, 225.22347176742275, 225.91773997839977, 226.45945173437548, 227.12567189517975, 227.51642229012563, 227.96829859640474, 228.47996003541195, 228.76107190040221, 226.4189254096958, 223.91764724512285, 223.23117521643087, 222.48718467724544, 221.9456332503363, 221.41367062456445, 220.8761919530412, 220.23973368373112, 219.4068524676711, 219.86104138665482, 222.92290328956537, 222.76495129689187, 222.58427828222167, 222.25680481414642, 222.0208623609733, 221.5968860635552, 221.39100387860464, 221.49563198982224, 221.40393206190254, 221.31485763476508, 221.19976412255608, 221.0888567681919, 221.06677662002747, 221.01456689210949, 221.0527851800606, 221.09549196529608, 220.9264169471766, 220.8304991827642, 220.82785689146283, 220.84043268399137, 220.72177686322723, 220.6345111468347, 220.55644747173685, 220.5402590623827, 220.48225606035743, 220.32087161306325, 220.11846055196474, 219.8640256189347, 219.64924927945688, 219.7536045590544, 219.8422693562694, 218.4031930662498, 214.5319582267555, 207.61882892034237, 197.49457221720758, 184.630714158023, 170.54591260604502, 158.4030182669329, 153.8075165339134, 154.47527859435257, 156.71929368175213, 162.25156612173976, 170.9538890288341, 182.18693584845872, 195.05212018672682, 206.2188748866844, 217.76901545437033, 225.6820571765245, 222.9976895844238, 220.0647761355623, 219.48677619173765, 218.79669141503646, 218.52796635690916, 218.45569181296025, 218.46156278856736, 218.549579972007, 218.34084474404497, 219.35602755748306, 223.06977804707998, 223.11503384681896, 222.9852365584214, 222.65965517515065, 222.31342433505662, 222.06471234403773, 221.9410105223669, 221.74277958375646, 221.66022405497193, 221.84712962001694, 221.88575662893146, 222.23993109513987, 222.4955356478094, 223.03038336409185, 223.27144521099504, 223.42837371143932, 223.85804156605815, 224.10381398938705, 224.07165969923227, 223.97780787672374, 223.82008476386866, 223.73628283256286, 223.63708505535965, 223.76627606393504, 223.9889370427336, 224.3673614055348, 225.11185280168365, 225.97940490668242, 226.8642371378034, 227.60879420193237, 228.4471285359262, 226.7211995262438, 225.23371021811445, 225.4061576476849, 225.3413731847518, 224.94638444033504, 224.5758371075391, 223.95789162594562, 223.4997408059089, 222.8913673823479, 223.37483154916856, 226.7894253640083, 226.85336503567444, 226.2459228281341, 224.2264539057997, 220.38012630707524, 215.23644906884803, 206.68869367458956, 196.44840238295063, 183.03686374884867, 167.1169259695031, 149.507102179271, 130.1937485434156, 110.57110560406726, 91.03958567818853, 72.82366360836305, 58.408183652265265, 58.408183652265265]}
  out "phase 2B":dbl=-0.03469454178376795
  in  "Phase 2B":u16(ring)=9 items=["X", "Y", "R", "Theta", "Frequency", "Noise", "Xh1", "Yh1", "Rh1", "Theta h1", "Xh2", "Yh2", "Rh2", "Theta h2"]
  out "phase Vaa_2":dbl=90.0
  in  "Phase 2A":u16(ring)=3 items=["X", "Y", "R", "Theta", "Frequency", "Noise", "Xh1", "Yh1", "Rh1", "Theta h1", "Xh2", "Yh2", "Rh2", "Theta h2"]
  out "Vaa_2(1w)/mV":dbl=0.13381974254969312
  in  "T Clear Plot 2A":bool
  in  "Parameter 2A":u16(ring)=2 items=["X", "Y", "R", "Theta", "Frequency", "Noise", "Xh1", "Yh1", "Rh1", "Theta h1", "Xh2", "Yh2", "Rh2", "Theta h2"]
  out "para2B Measurement":dbl=224.31020276269777
  in  "T Clear Plot 2B":bool
  in  "Parameter 2B":u16(ring)=8 items=["X", "Y", "R", "Theta", "Frequency", "Noise", "Xh1", "Yh1", "Rh1", "Theta h1", "Xh2", "Yh2", "Rh2", "Theta h2"]
  in  "Save data or not":bool=TRUE
  in  "path1 (folder + filename)":string="H:\\My Drive\\Lab\\Opticool\\Measurement\\NLH\\T dependence\\TaI29_A1112_B116_test"
  in  "V Loop#":i32=1
  in  "Two Devices ?":bool=TRUE
  in  "LOCKIN2 address":refnum<visa-resource-name>="COM4"
  in  "2B frequency 2":dbl=26.7 format="%#_13g"
  in  "2B Input Connection (0: Single-Ended)":u16(ring)=1 items=["Single-Ended Voltage", "Differential Voltage", "1 MOhm Current Gain", "100 MOhm Current Gain"]
  in  "2B harmonic 1":u8=2
  in  "2B harmonic 2":u8=3
  in  "2B reference Manual Phase":dbl
  in  "auto phase 2B":bool=TRUE
  in  "2B Sample time (s)":dbl=0.001 min=0.001 max=100.0 step=0.001
  in  "2B Sensitivity":u16(ring)=27 items=["1 nV/fA", "2 nV/fA", "5 nV/fA", "10 nV/fA", "20 nV/fA", "50 nV/fA", "100 nV/fA", "200 nV/fA", "500 nV/fA", "1 uV/pA", "2 uV/pA", "5 uV/pA", "10 uV/pA", "20 uV/pA", "50 uV/pA", "100 uV/pA", "200 uV/pA", "500 uV/pA", "1 mV/nA", "2 mV/nA", "5 mV/nA", "10 mV/nA", "20 mV/nA", "50 mV/nA", "100 mV/nA", "200 mV/nA", "500 mV/nA", "1 V/uA"]
  in  "Enable Sync Filter 2B (open when f<200Hz)":bool
  in  "2B Time Constant":u8(ring)=9 items=["10 us", "30 us", "100 us", "300 us", "1 ms", "3 ms", "10 ms", "30 ms", "100 ms", "300 ms", "1 s", "3 s", "10 s", "30 s", "100 s", "300 s", "1 ks", "3 ks"]
  in  "2B Reference Source":u8(ring)=3 items=["External", "Internal", "Internal Sweep", "Channel-A"]
  in  "2B Low Pass Filter Slope":u8(ring)=2 items=["6 dB/oct", "12 dB/oct", "18 db/oct", "24 dB/oct"]
  in  "2A frequency":dbl=36.7 format="%#_13g"
  in  "2A Input Connection (0: Single-Ended)":u16(ring)=1 items=["Single-Ended Voltage", "Differential Voltage", "1 MOhm Current Gain", "100 MOhm Current Gain"]
  in  "2A harmonic 1":u8=2
  in  "2A harmonic 2":u8=3
  in  "2A reference Manual Phase":dbl
  in  "auto phase 2A":bool=TRUE
  in  "2A Reference Source":u8(ring)=1 items=["External", "Internal", "Internal Sweep"]
  in  "2A Sample time (s)":dbl=0.001 min=0.001 max=100.0 step=0.001
  in  "2A Time Constant":u8(ring)=9 items=["10 us", "30 us", "100 us", "300 us", "1 ms", "3 ms", "10 ms", "30 ms", "100 ms", "300 ms", "1 s", "3 s", "10 s", "30 s", "100 s", "300 s", "1 ks", "3 ks"]
  in  "Enable Sync Filter 2A (open when f<200Hz)":bool
  in  "2A Sensitivity":u16(ring)=27 items=["1 nV/fA", "2 nV/fA", "5 nV/fA", "10 nV/fA", "20 nV/fA", "50 nV/fA", "100 nV/fA", "200 nV/fA", "500 nV/fA", "1 uV/pA", "2 uV/pA", "5 uV/pA", "10 uV/pA", "20 uV/pA", "50 uV/pA", "100 uV/pA", "200 uV/pA", "500 uV/pA", "1 mV/nA", "2 mV/nA", "5 mV/nA", "10 mV/nA", "20 mV/nA", "50 mV/nA", "100 mV/nA", "200 mV/nA", "500 mV/nA", "1 V/uA"]
  in  "2A Low Pass Filter Slope":u8(ring)=2 items=["6 dB/oct", "12 dB/oct", "18 db/oct", "24 dB/oct"]
  in  "T Delay":dbl=5.0
  out "Temperature":dbl
  out "Field":dbl
  out "Field Status 2":i32(ring) items=["MagnetUnknown"=0, "StablePersistent"=1, "WarmingSwitch"=2, "CoolingSwitch"=3, "StableDriven"=4, "Iterating"=5, "Charging"=6, "Discharging"=7, "CurrentError"=8, "MagnetFailure"=15]
  out "Temperature Status 2":i32(ring) items=["TemperatureUnknown"=0, "Stable"=1, "Tracking"=2, "Near"=5, "Chasing"=6, "Filling"=7, "Standby"=10, "Disabled"=13, "ImpedanceNotFunction"=14, "TempFailure"=15]
  in  "?":bool
  out "Sine voltage F":dbl format="%#_13g"
  out "Sine voltage T":dbl=0.09999999999999964 format="%#_13g"
  in  "Initialization?":bool
  in  "F Delay":dbl=5.0
  out "V Loop Run F":i32
  out "Backward":bool
  out "Forward":bool=TRUE
  in  "V Step(mV)":i32=50
  out "V Loop Run T":i32=1
  in  "High Value (V)":dbl=3.5
  in  "Low Value (V)":dbl=0.1
  in  "System Stablization (s)":dbl=0.5 format="%#_13g"
  in  "Low Value (Oe)":dbl
  in  "High Value (Oe)":dbl=70000.0
  in  "Sweep Field Approach":i32(ring) items=["Linear", "NoOvershoot", "Oscillate"]
  in  "Sweep F Rate (Oe/s)":dbl=200.0 format="%#_13g"
  in  "Sweep F mode":i32(ring) items=["Persistent", "Driven"]
  in  "Set Fixed T":dbl=300.0
  in  "Fixed Temperature Approach":i32(ring)=1 items=["FastSettle", "NoOvershoot"]
  in  "FIxed T  Rate (K/min)":dbl=20.0
  out "Field Setting":dbl format="%#_13g"
  out "Fixed Temperature":dbl
  out "Measured Field":dbl
  out "Field Status":i32(ring) items=["MagnetUnknown"=0, "StablePersistent"=1, "WarmingSwitch"=2, "CoolingSwitch"=3, "StableDriven"=4, "Iterating"=5, "Charging"=6, "Discharging"=7, "CurrentError"=8, "MagnetFailure"=15]
  out "Temperature Status":i32(ring) items=["TemperatureUnknown"=0, "Stable"=1, "Tracking"=2, "Near"=5, "Chasing"=6, "Filling"=7, "Standby"=10, "Disabled"=13, "ImpedanceNotFunction"=14, "TempFailure"=15]
  out "Measuring F":bool
  in  "Step(Oe)":i32=5000
  out "Temperature Status":i32(ring)=1 items=["TemperatureUnknown"=0, "Stable"=1, "Tracking"=2, "Near"=5, "Chasing"=6, "Filling"=7, "Standby"=10, "Disabled"=13, "ImpedanceNotFunction"=14, "TempFailure"=15]
  out "Field Status":i32(ring)=4 items=["MagnetUnknown"=0, "StablePersistent"=1, "WarmingSwitch"=2, "CoolingSwitch"=3, "StableDriven"=4, "Iterating"=5, "Charging"=6, "Discharging"=7, "CurrentError"=8, "MagnetFailure"=15]
  out "Fixed Field":dbl=0.222309460490942
  out "Measured Temp":dbl=2.131896138191223
  in  "Set FIxed F (Oe)":dbl format="%#_13g"
  in  "Fixed Field Approach":i32(ring) items=["Linear", "NoOvershoot", "Oscillate"]
  in  "FIxed F Rate (Oe/s)":dbl=100.0 format="%#_13g"
  in  "Fixed F mode":i32(ring) items=["Persistent", "Driven"]
  in  "Sweep Temperature Approach":i32(ring)=1 items=["FastSettle", "NoOvershoot"]
  in  "Sweep T  Rate (K/min)":dbl=10.0
  in  "Sweep T/F":bool=TRUE
  in  "Remote":bool=TRUE
  in  "IP Address":string="169.254.170.239"
  out "Measuring T":bool
  in  "LOCKIN1 address":refnum<visa-resource-name>="COM3"
  out "Temp Setting":dbl=2.0 format="%#_13g"
  in  "Step(K)":i32=10
  in  "B frequency":dbl=26.7 format="%#_13g"
  in  "B Input Connection (0: Single-Ended)":u16(ring)=1 items=["Single-Ended Voltage", "Differential Voltage", "1 MOhm Current Gain", "100 MOhm Current Gain"]
  in  "B harmonic 1":u8=2
  in  "B harmonic 2":u8=3
  in  "B reference Manual Phase":dbl
  in  "auto phase B":bool=TRUE
  in  "B Sample time (s)":dbl=0.001 min=0.001 max=100.0 step=0.001
  in  "B Sensitivity":u16(ring)=27 items=["1 nV/fA", "2 nV/fA", "5 nV/fA", "10 nV/fA", "20 nV/fA", "50 nV/fA", "100 nV/fA", "200 nV/fA", "500 nV/fA", "1 uV/pA", "2 uV/pA", "5 uV/pA", "10 uV/pA", "20 uV/pA", "50 uV/pA", "100 uV/pA", "200 uV/pA", "500 uV/pA", "1 mV/nA", "2 mV/nA", "5 mV/nA", "10 mV/nA", "20 mV/nA", "50 mV/nA", "100 mV/nA", "200 mV/nA", "500 mV/nA", "1 V/uA"]
  in  "Enable Sync Filter B (open when f<200Hz)":bool
  in  "B Time Constant":u8(ring)=9 items=["10 us", "30 us", "100 us", "300 us", "1 ms", "3 ms", "10 ms", "30 ms", "100 ms", "300 ms", "1 s", "3 s", "10 s", "30 s", "100 s", "300 s", "1 ks", "3 ks"]
  in  "B Reference Source":u8(ring)=3 items=["External", "Internal", "Internal Sweep", "Channel-A"]
  in  "B Low Pass Filter Slope":u8(ring)=2 items=["6 dB/oct", "12 dB/oct", "18 db/oct", "24 dB/oct"]
  in  "A frequency":dbl=26.7 format="%#_13g"
  in  "A Input Connection (0: Single-Ended)":u16(ring)=1 items=["Single-Ended Voltage", "Differential Voltage", "1 MOhm Current Gain", "100 MOhm Current Gain"]
  in  "A harmonic 1":u8=2
  in  "A harmonic 2":u8=3
  in  "A reference Manual Phase":dbl
  in  "auto phase A":bool=TRUE
  in  "A Reference Source":u8(ring)=1 items=["External", "Internal", "Internal Sweep"]
  in  "A Sample time (s)":dbl=0.001 min=0.001 max=100.0 step=0.001
  in  "A Time Constant":u8(ring)=9 items=["10 us", "30 us", "100 us", "300 us", "1 ms", "3 ms", "10 ms", "30 ms", "100 ms", "300 ms", "1 s", "3 s", "10 s", "30 s", "100 s", "300 s", "1 ks", "3 ks"]
  in  "Enable Sync Filter A (open when f<200Hz)":bool
  in  "A Sensitivity":u16(ring)=27 items=["1 nV/fA", "2 nV/fA", "5 nV/fA", "10 nV/fA", "20 nV/fA", "50 nV/fA", "100 nV/fA", "200 nV/fA", "500 nV/fA", "1 uV/pA", "2 uV/pA", "5 uV/pA", "10 uV/pA", "20 uV/pA", "50 uV/pA", "100 uV/pA", "200 uV/pA", "500 uV/pA", "1 mV/nA", "2 mV/nA", "5 mV/nA", "10 mV/nA", "20 mV/nA", "50 mV/nA", "100 mV/nA", "200 mV/nA", "500 mV/nA", "1 V/uA"]
  in  "A Low Pass Filter Slope":u8(ring)=2 items=["6 dB/oct", "12 dB/oct", "18 db/oct", "24 dB/oct"]
  in  "End Value (K)":dbl=2.0
  in  "Start Value (K)":dbl=2.0
  in  "Single/Double":i32=2 min=1 max=2 step=1
  # "Statue"
  # "Mesurement 1T"
  # "Ri_1 Measurement"
  # "Mesurement 1F"
  # "Lock-in Setting"
  # "Channel 1A"
  # "Sweep Setting"
  # "Channel 1B"
  # "Channel 2A"
  # "Current Measurement"
  # "Channel 2B"
  # "Mesurement 2F"
  # "Mesurement 2T"
  # "Ri_2 Measurement"
  # "Sweep F Mesurement"
  # "Temprature and Field Setting"
  # "Sweep T Mesurement"
  # "Sweep F"
  # "Sweep T"
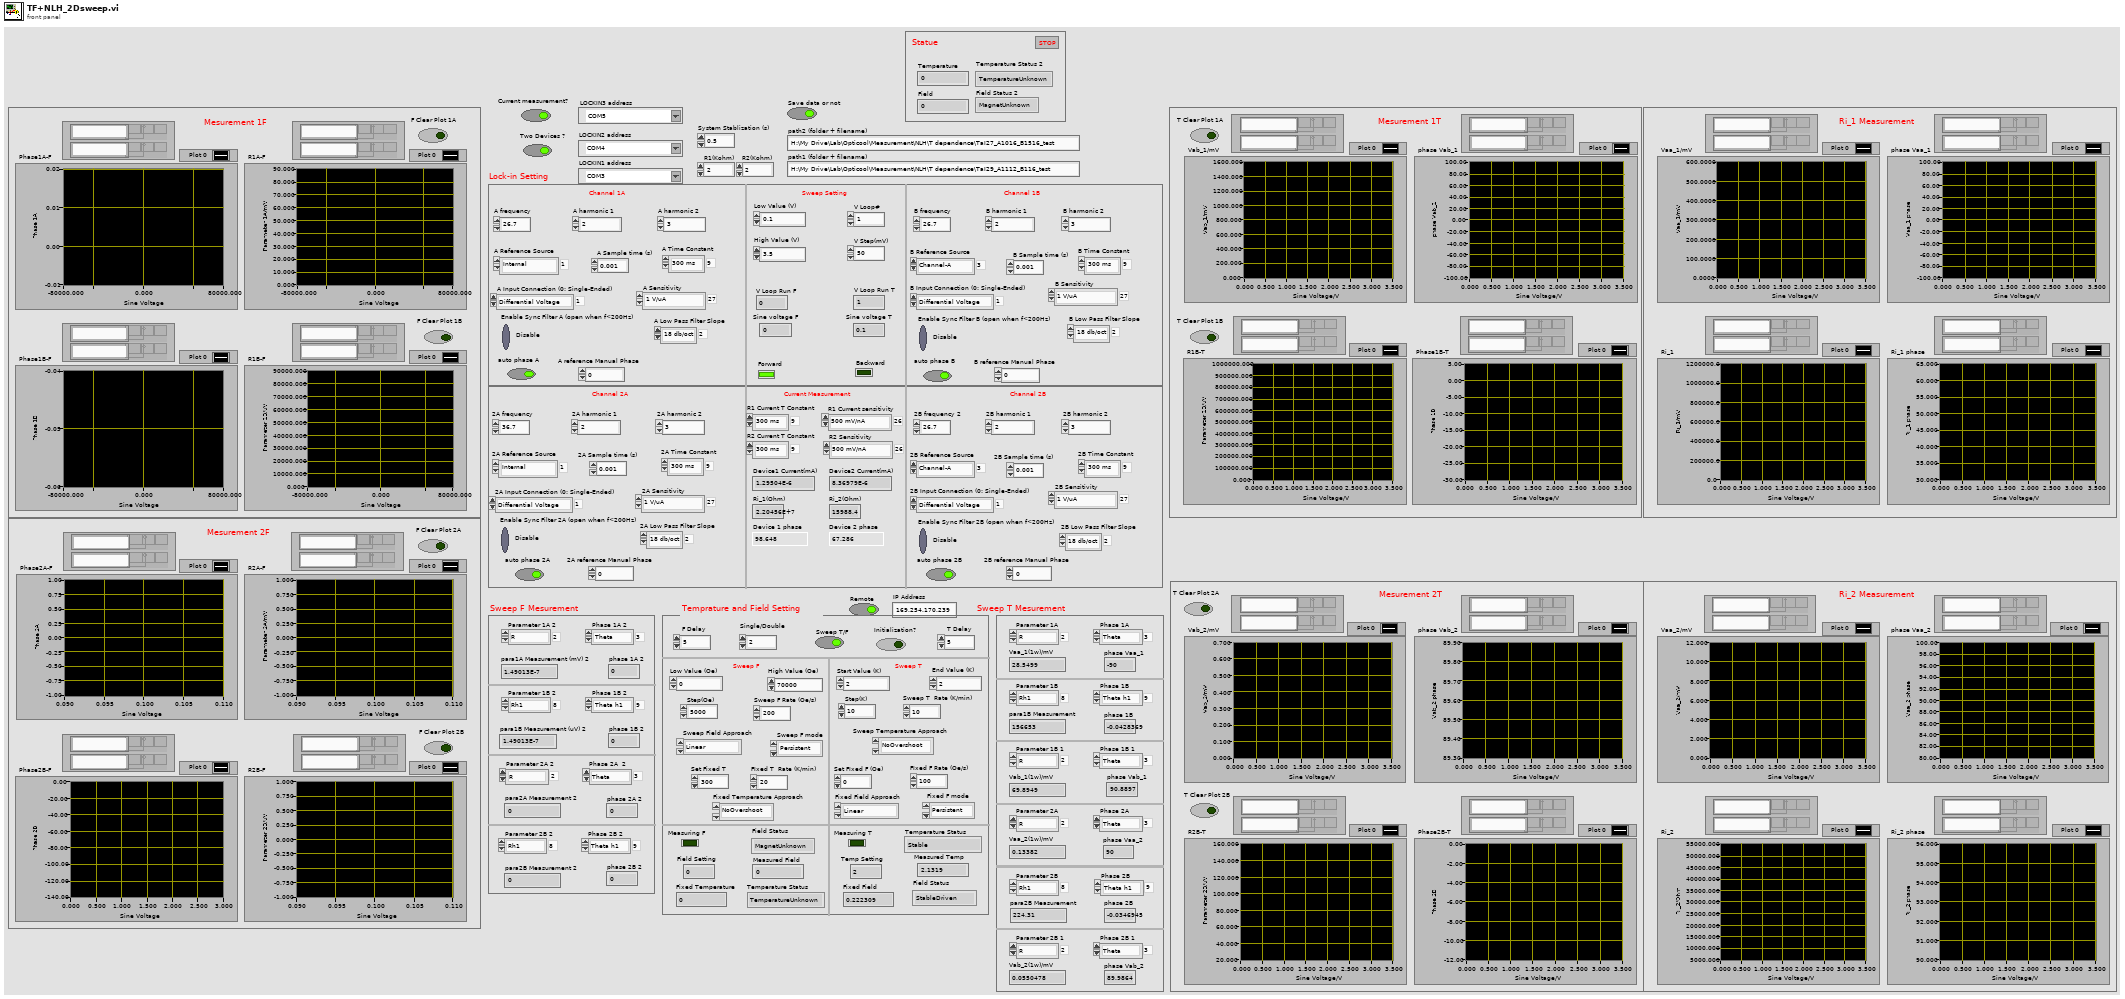
[diagram p1: front panel]
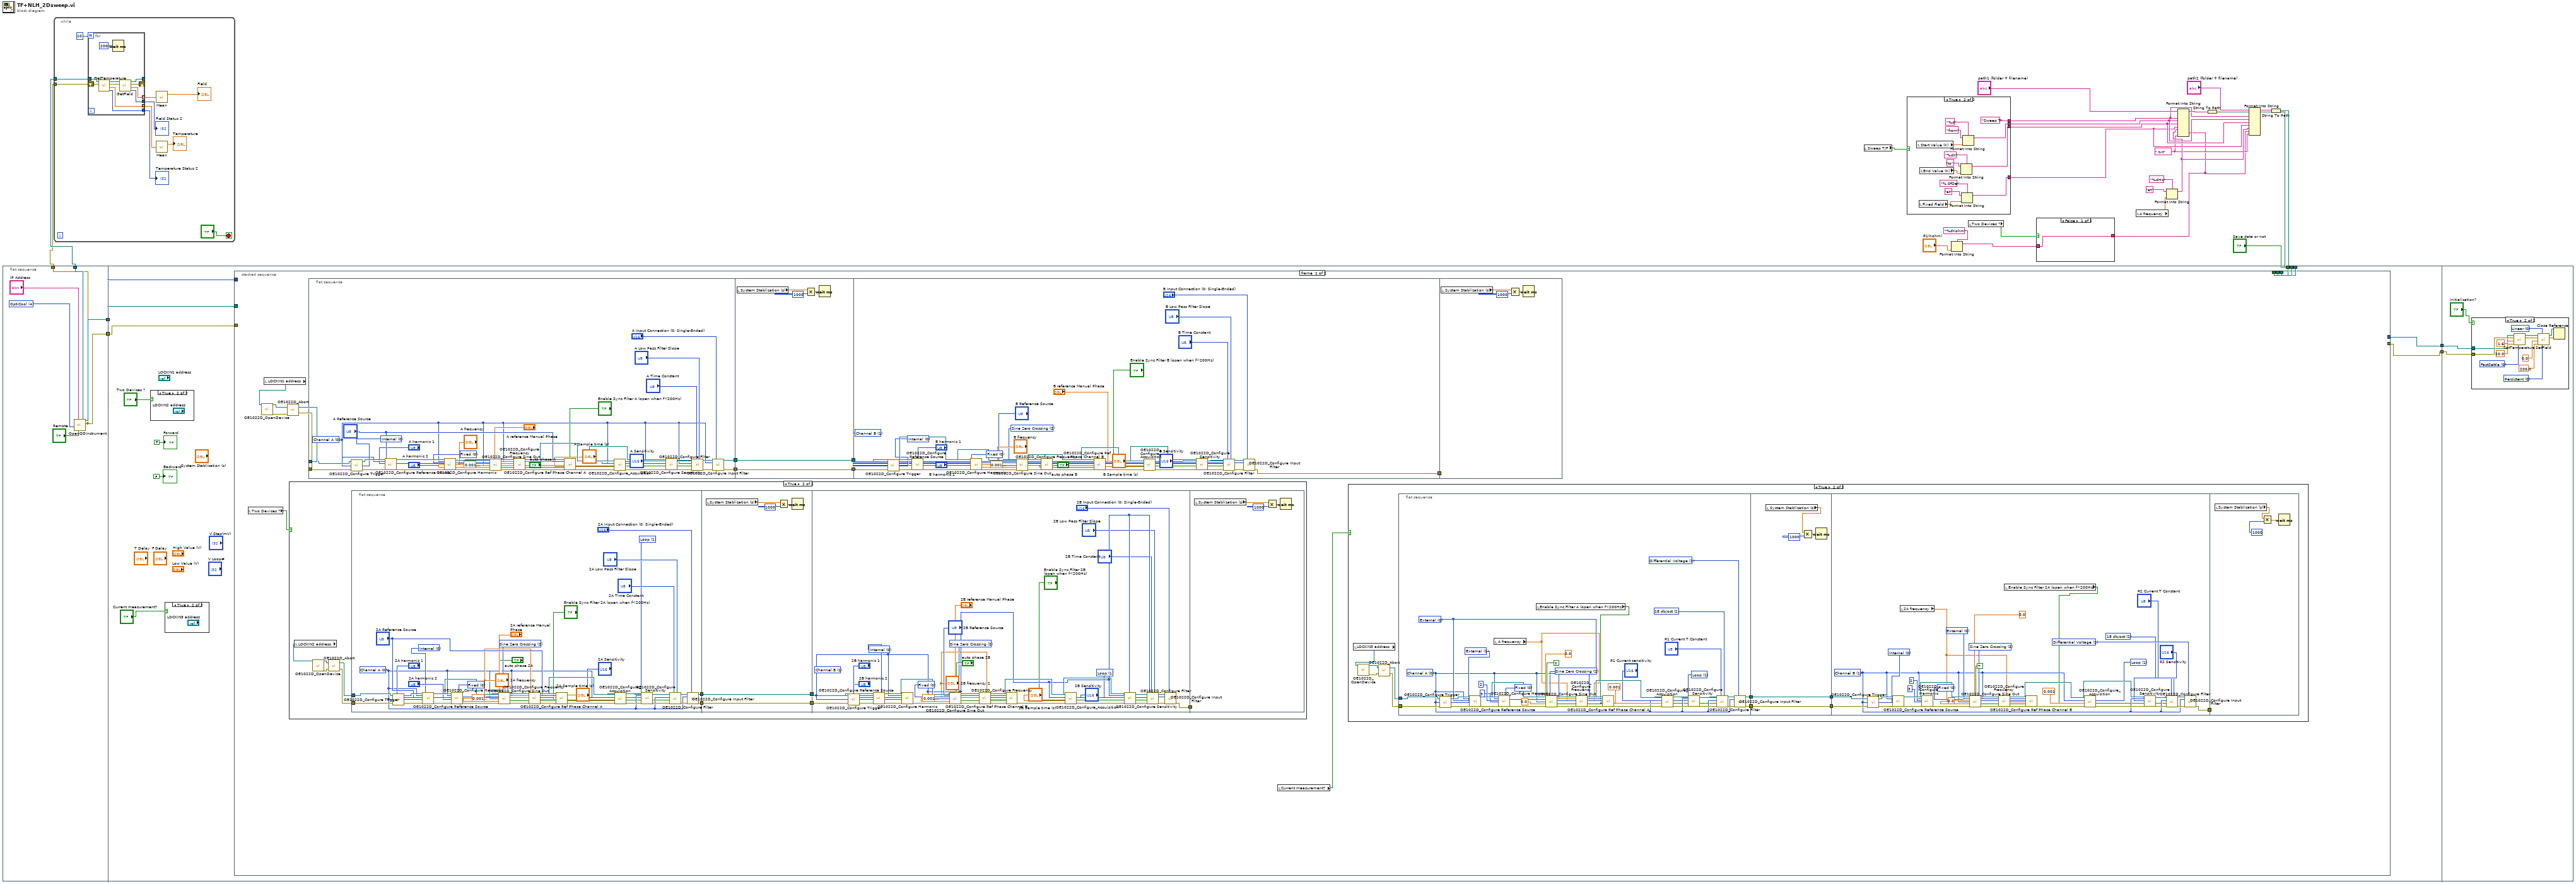
[diagram p0: block diagram]
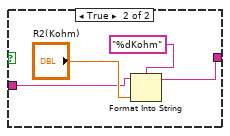
[diagram p2: hidden frame]
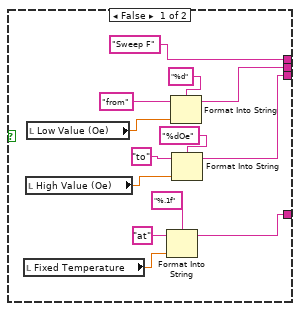
[diagram p3: hidden frame]
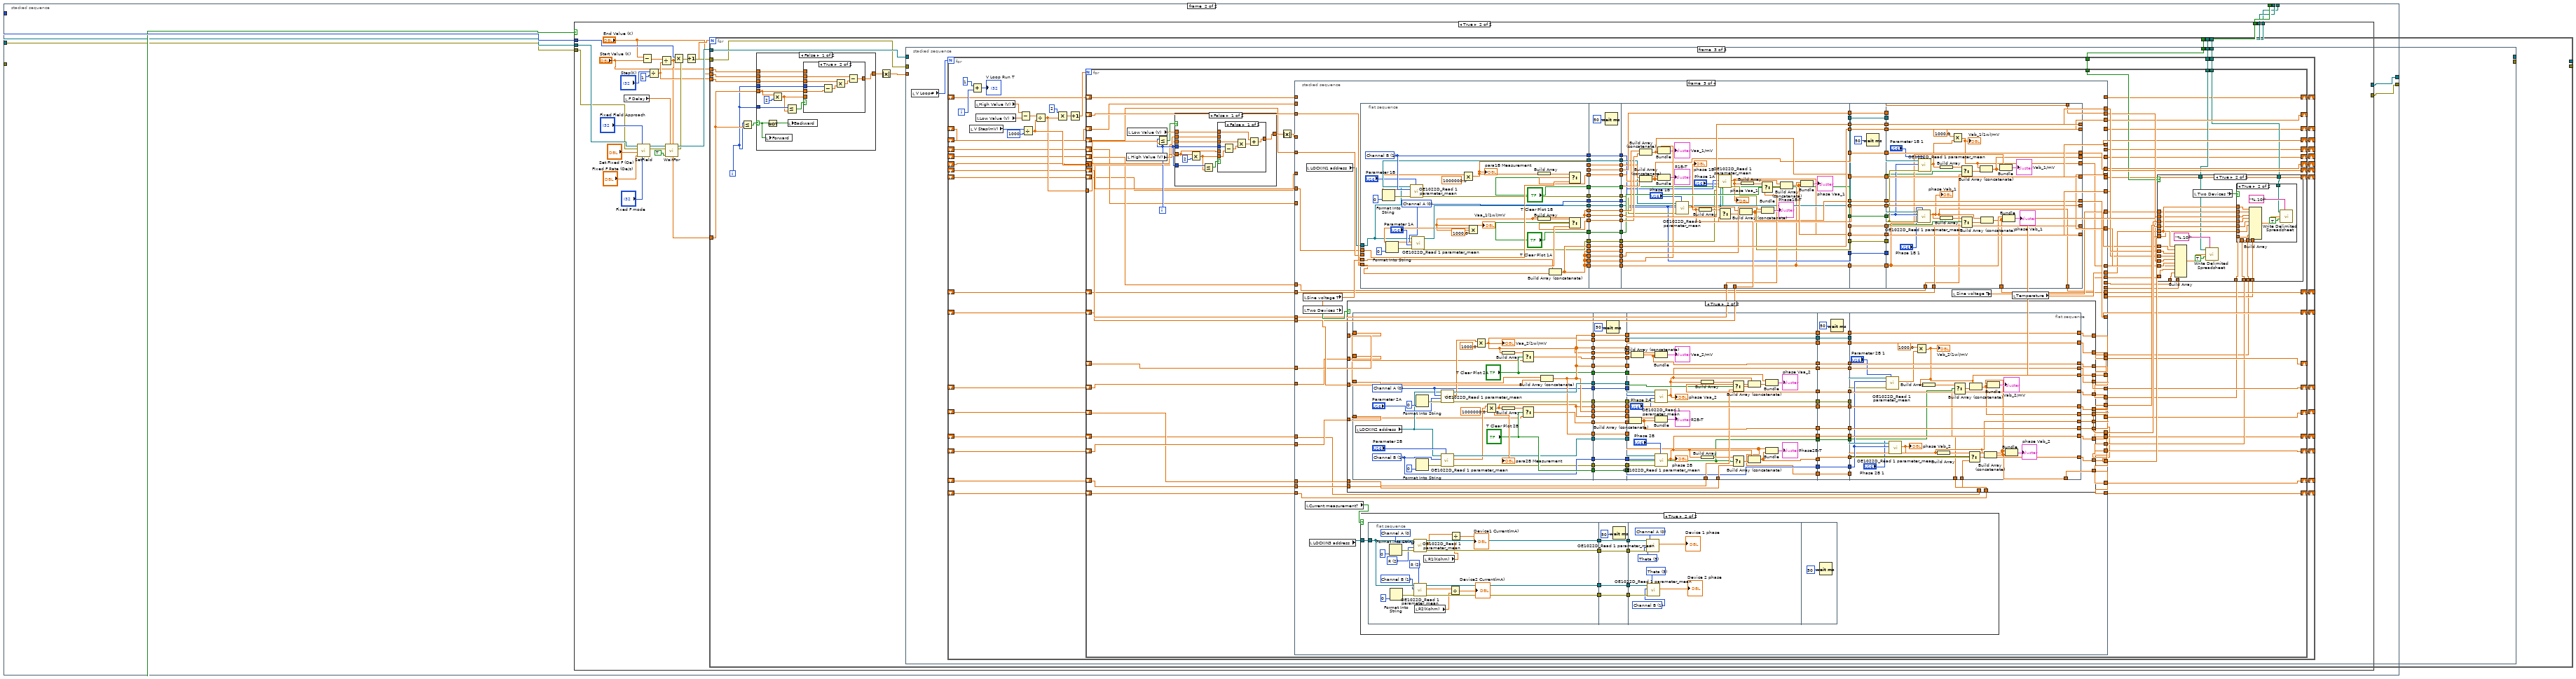
[diagram p8: hidden frame]
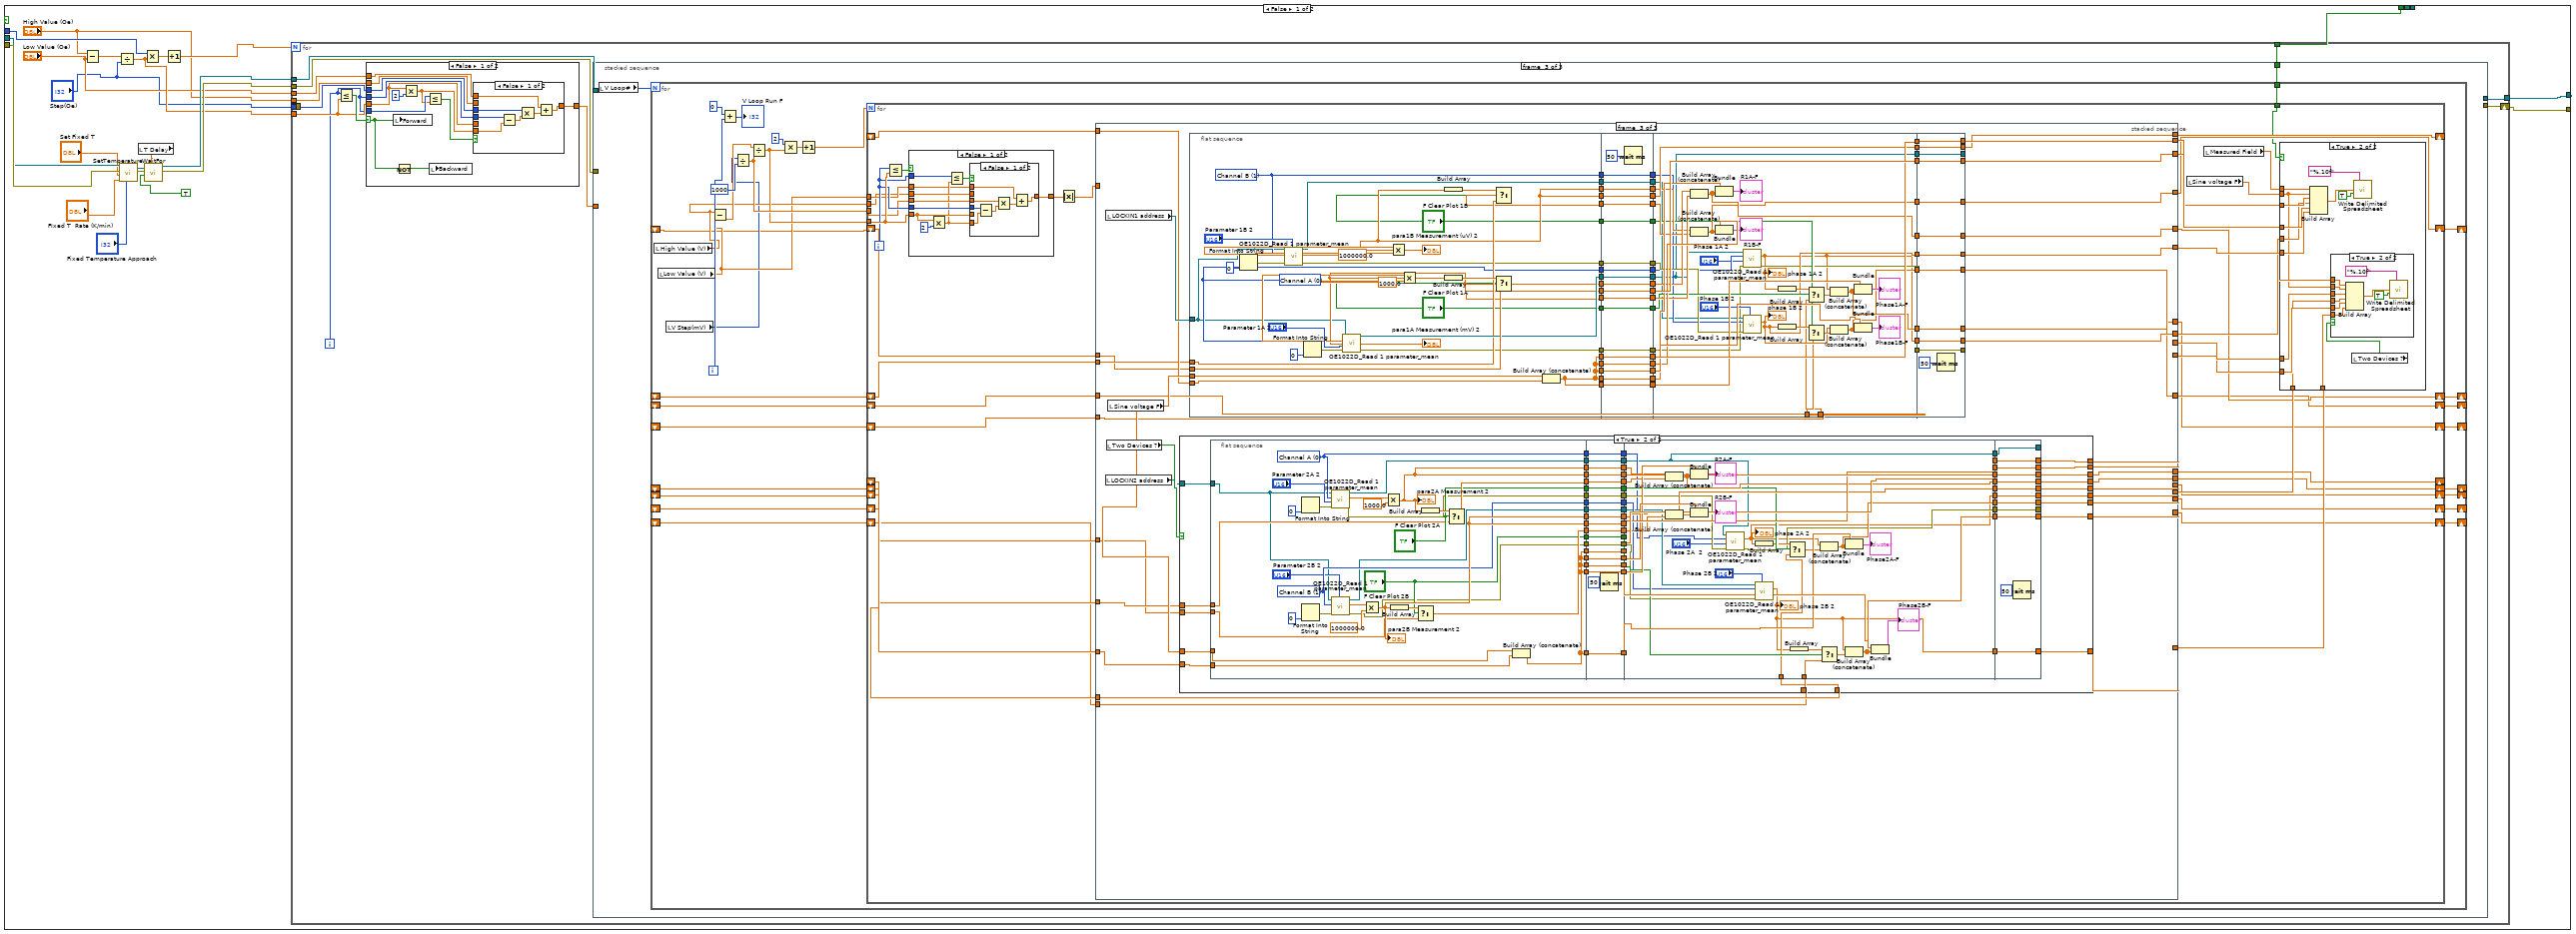
[diagram p9: hidden frame]
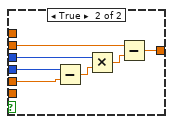
[diagram p10: hidden frame]
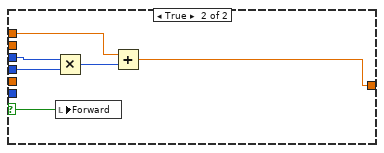
[diagram p11: hidden frame]
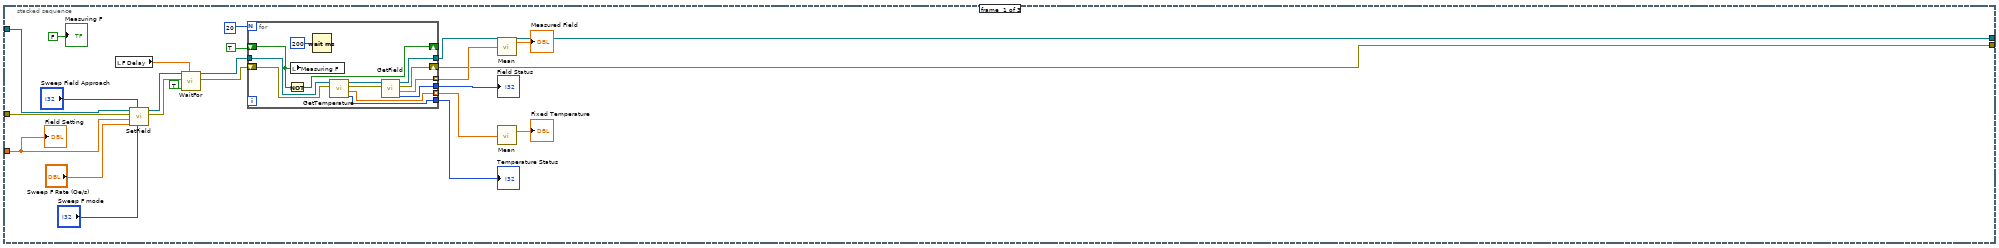
[diagram p12: hidden frame]
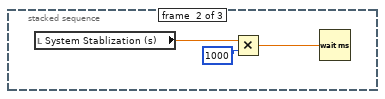
[diagram p13: hidden frame]
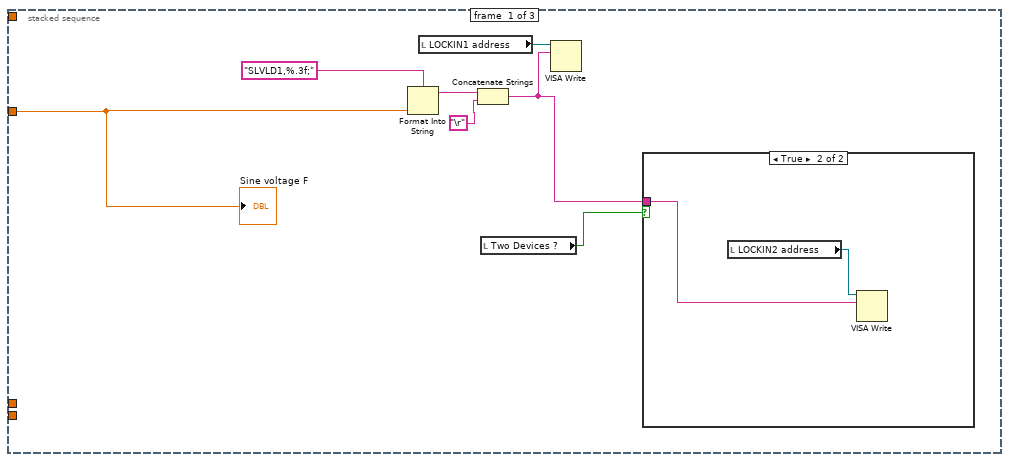
[diagram p14: hidden frame]
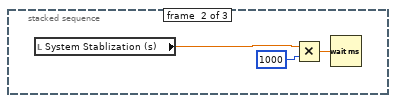
[diagram p16: hidden frame]
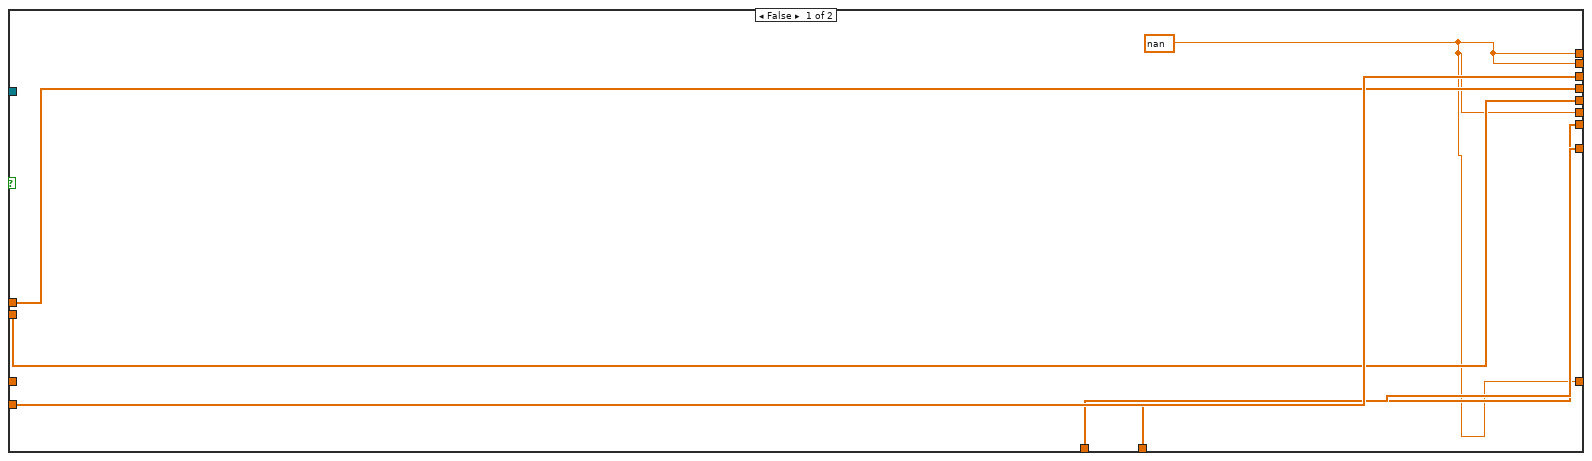
[diagram p17: hidden frame]
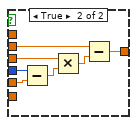
[diagram p18: hidden frame]
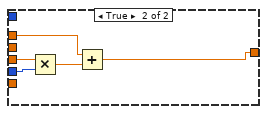
[diagram p19: hidden frame]
diagram:
  w9 = ".txt"
  n1 = flat-sequence {
    tunnel: [w30] -> w28
    tunnel: [w29] -> w27
    tunnel: [w30] -> w24
    tunnel: [w29] -> w23
    tunnel: w28 -> [w44]
    tunnel: w27 -> [w43]
    tunnel: [w42] -> w26
    tunnel: [w41] -> w25
    tunnel: w8 -> [w37]
    tunnel: w7 -> [w36]
    tunnel: "Save data or not" -> [w35]
    tunnel: w26 -> [w1801]
    tunnel: w25 -> [w1800]
    frame #0 {
      w31 = 4 items=["PPMS", "VersaLab", "DynaCool", "SVSM", "OptiCool"] ("InstrumentType")
      n2 = call "OpenQDInstrument.vi"("Remote"="Remote", "IP Address"="IP Address", "InstrumentType"=w31) -> ("error out"=w29:errorcluster, "Instrument Ref"=w30:refnum<k24>)  [unwired: 5 in]
    }
    frame #1 {
      n3 = case shown="True" "Two Devices ?" {
        frame False {
        }
        frame True {
        }
      }
      n4 = case shown="True" "Current measurement?" {
        frame False {
        }
        frame True {
        }
      }
      n5 = stacked-sequence {
        tunnel: "Single/Double" -> [_ w344]
        tunnel: w44 -> [_ w342]
        tunnel: w43 -> [_ w341]
        tunnel: [_ w340] -> w42
        tunnel: [_ w339] -> w41
        tunnel: w37 -> [_ w337]
        tunnel: w36 -> [_ w336]
        tunnel: w35 -> [_ w338]
        frame #0 {
          n6 = local read "Two Devices ?"() -> (w47:bool)
          n7 = local read "LOCKIN1 address"() -> (w48:refnum<visa-resource-name>)
          n8 = call "OE1022D_OpenDevice.vi"("VISA resource name"=w48) -> ("VISA资源名称输出"=w49:refnum<visa-resource-name>, "错误输出"=w50:errorcluster)  [unwired: 17 in]
          n9 = call "OE1022D_Abort.vi"("error in (no error)"=w50, "VISA resource name"=w49) -> ("error out"=w55:errorcluster, "VISA resource name out"=w56:refnum<visa-resource-name>)
          n10 = case shown="True" w47 {
            frame False {
            }
            frame True {
              n11 = local read "LOCKIN2 address"() -> (w155:refnum<visa-resource-name>)
              n12 = call "OE1022D_OpenDevice.vi"("VISA resource name"=w155) -> ("VISA资源名称输出"=w158:refnum<visa-resource-name>, "错误输出"=w159:errorcluster)  [unwired: 17 in]
              n13 = call "OE1022D_Abort.vi"("error in (no error)"=w159, "VISA resource name"=w158) -> ("error out"=w156:errorcluster, "VISA resource name out"=w157:refnum<visa-resource-name>)
              n14 = flat-sequence {
                tunnel: w157 -> [w204]
                tunnel: [w192] -> w164
                tunnel: w156 -> [w203]
                tunnel: [w180] -> w163
                tunnel: w164 -> [w209]
                tunnel: [w209] -> w162
                tunnel: w163 -> [w208]
                tunnel: [w208] -> w161
                tunnel: w162 -> [w231]
                tunnel: [w230] -> w160
                tunnel: w161 -> [w229]
                tunnel: w160 -> [_]
                frame #0 {
                  w165 = u8 2 items=["TTL Pos", "TTL Neg", "Sine Zero Crossing"] ("External Ref Trigger")
                  w166 = u8 1 items=["Single", "Loop"] ("Sample Mode (Single/Loop)")
                  w179 = u8 0 items=["Fixed", "Linear", "Log"] ("SineOut Mode")
                  w181 = u16 0 items=["Internal", "External"] ("Trigger Source (0: Internal)")
                  w170 = u8 0 items=["Channel A", "Channel B"] ("OE1022D A/B")
                  n15 = call "OE1022D_Configure Trigger.vi"("Trigger Source (0: Internal)"=w181, "error in (no error)   2"=w203, "OE1022D A/B"=w170, "VISA resource name   2"=w204) -> ("error out   2"=w197:errorcluster, "VISA resource name out   2"=w198:refnum<visa-resource-name>)
                  n16 = call "OE1022D_Configure Reference Source.vi"("VISA resource name"=w198, "OE1022D A/B"=w170, "Reference Source"="2A Reference Source", "error in (no error)"=w197) -> ("VISA resource name out"=w196:refnum<visa-resource-name>, "error out"=w194:errorcluster)  [unwired: 14 in]
                  n17 = call "OE1022D_Configure Harmonic.vi"("VISA resource name"=w196, "OE1022D A/B"=w170, "Harmonic 1"="2A harmonic 1", "Harmonic 2"="2A harmonic 2", "error in (no error)"=w194) -> ("VISA resource name out"=w195:refnum<visa-resource-name>, "error out"=w193:errorcluster)  [unwired: 13 in]
                  n18 = call "OE1022D_Configure Sine Out.vi"("VISA resource name"=w195, "SineOut Mode"=w179, "OE1022D A/B"=w170, "Sine Output Amplitude (V)"=sgl 0.001, "error in (no error)"=w193) -> ("VISA resource name out"=w201:refnum<visa-resource-name>, "error out"=w200:errorcluster)  [unwired: 9 in]
                  n19 = call "OE1022D_Configure Frequency.vi"("VISA resource name"=w201, "OE1022D A/B"=w170, "Internal Frequency(Hz)"="2A frequency", "error in (no error)"=w200) -> ("VISA resource name out"=w191:refnum<visa-resource-name>, "error out"=w188:errorcluster)  [unwired: 14 in]
                  n20 = call "OE1022D_Configure Ref Phase Channel A.vi"("VISA resource name"=w191, "Reference Source"="2A Reference Source", "External Ref Trigger"=w165, "Internal Frequency(Hz)"="2A frequency", "Auto Phase (T: Enabled)"="auto phase 2A", "error in (no error)"=w188, "Manual Phase  (degree)"="2A reference Manual Phase") -> ("VISA resource name out"=w190:refnum<visa-resource-name>, "error out"=w189:errorcluster)  [unwired: 11 in]
                  n21 = call "OE1022D_Configure_Acquisition.vi"("VISA resource name"=w190, "OE1022D A/B"=w170, "Sample time (s)"="2A Sample time (s)", "error in (no error)"=w189, "Sample Mode (Single/Loop)"=w166) -> ("VISA resource name out"=w173:refnum<visa-resource-name>, "error out"=w172:errorcluster)  [unwired: 3 in]
                  n22 = call "OE1022D_Configure Sensitivity.vi"("VISA resource name"=w173, "OE1022D A/B"=w170, "Sensitivity"="2A Sensitivity", "error in (no error)"=w172) -> ("VISA resource name out"=w177:refnum<visa-resource-name>, "error out"=w176:errorcluster)  [unwired: 14 in]
                  n23 = call "OE1022D_Configure Filter.vi"("Low Pass Filter Slope (1: 12dB/oct)"="2A Low Pass Filter Slope", "Time Constant (8: 100ms)"="2A Time Constant", "error in (no error)"=w176, "Enable Sync Filter (F: Disable)"="Enable Sync Filter 2A (open when f<200Hz)", "OE1022D A/B"=w170, "VISA resource name"=w177) -> ("error out"=w174:errorcluster, "VISA resource name out"=w175:refnum<visa-resource-name>)  [unwired: 4 in]
                  n24 = call "OE1022D_Configure Input Filter.vi"("VISA resource name"=w175, "Input Source"="2A Input Connection (0: Single-Ended)", "OE1022D A/B"=w170, "error in (no error)"=w174) -> ("VISA resource name out"=w180:refnum<visa-resource-name>, "error out"=w192:errorcluster)  [unwired: 10 in]
                }
                frame #1 {
                  n25 = local read "System Stablization (s)"() -> (w205:dbl)
                  n26 = Multiply(x=w205, y=1000) -> (x*y=w207:dbl)
                  n27 = Wait (ms)(milliseconds to wait=w207) -> ()  [unwired: 1 out]
                }
                frame #2 {
                  w211 = u8 1 items=["Single", "Loop"] ("Sample Mode (Single/Loop)")
                  w213 = u8 2 items=["TTL Pos", "TTL Neg", "Sine Zero Crossing"] ("External Ref Trigger")
                  w226 = u8 0 items=["Fixed", "Linear", "Log"] ("SineOut Mode")
                  w232 = u16 0 items=["Internal", "External"] ("Trigger Source (0: Internal)")
                  w218 = u8 1 items=["Channel A", "Channel B"] ("OE1022D A/B")
                  n28 = call "OE1022D_Configure Trigger.vi"("Trigger Source (0: Internal)"=w232, "error in (no error)   2"=w231, "OE1022D A/B"=w218, "VISA resource name   2"=w229) -> ("error out   2"=w244:errorcluster, "VISA resource name out   2"=w245:refnum<visa-resource-name>)
                  n29 = call "OE1022D_Configure Reference Source.vi"("VISA resource name"=w245, "OE1022D A/B"=w218, "error in (no error)"=w244) -> ("VISA resource name out"=w243:refnum<visa-resource-name>, "error out"=w241:errorcluster)  [unwired: 15 in]
                  n30 = call "OE1022D_Configure Harmonic.vi"("VISA resource name"=w243, "OE1022D A/B"=w218, "Harmonic 1"="2B harmonic 1", "Harmonic 2"="2B harmonic 2", "error in (no error)"=w241) -> ("VISA resource name out"=w242:refnum<visa-resource-name>, "error out"=w240:errorcluster)  [unwired: 13 in]
                  n31 = call "OE1022D_Configure Sine Out.vi"("VISA resource name"=w242, "SineOut Mode"=w226, "OE1022D A/B"=w218, "Sine Output Amplitude (V)"=sgl 0.001, "error in (no error)"=w240) -> ("VISA resource name out"=w247:refnum<visa-resource-name>, "error out"=w246:errorcluster)  [unwired: 9 in]
                  n32 = call "OE1022D_Configure Frequency.vi"("VISA resource name"=w247, "OE1022D A/B"=w218, "Internal Frequency(Hz)"="2B frequency 2", "error in (no error)"=w246) -> ("VISA resource name out"=w239:refnum<visa-resource-name>, "error out"=w236:errorcluster)  [unwired: 14 in]
                  n33 = call "OE1022D_Configure Ref Phase Channel B.vi"("VISA resource name"=w239, "Reference Source"="2B Reference Source", "External Ref Trigger"=w213, "Internal Frequency(Hz)"="2B frequency 2", "Auto Phase (T: Enabled)"="auto phase 2B", "error in (no error)"=w236, "Manual Phase  (degree)"="2B reference Manual Phase") -> ("VISA resource name out"=w238:refnum<visa-resource-name>, "error out"=w237:errorcluster)  [unwired: 11 in]
                  n34 = call "OE1022D_Configure_Acquisition.vi"("VISA resource name"=w238, "OE1022D A/B"=w218, "Sample time (s)"="2B Sample time (s)", "error in (no error)"=w237, "Sample Mode (Single/Loop)"=w211) -> ("VISA resource name out"=w219:refnum<visa-resource-name>, "error out"=w220:errorcluster)  [unwired: 3 in]
                  n35 = call "OE1022D_Configure Sensitivity.vi"("VISA resource name"=w219, "OE1022D A/B"=w218, "Sensitivity"="2B Sensitivity", "error in (no error)"=w220) -> ("VISA resource name out"=w223:refnum<visa-resource-name>, "error out"=w222:errorcluster)  [unwired: 14 in]
                  n36 = call "OE1022D_Configure Filter.vi"("Low Pass Filter Slope (1: 12dB/oct)"="2B Low Pass Filter Slope", "Time Constant (8: 100ms)"="2B Time Constant", "error in (no error)"=w222, "Enable Sync Filter (F: Disable)"="Enable Sync Filter 2B (open when f<200Hz)", "OE1022D A/B"=w218, "VISA resource name"=w223) -> ("error out"=w221:errorcluster, "VISA resource name out"=w210:refnum<visa-resource-name>)  [unwired: 4 in]
                  n37 = call "OE1022D_Configure Input Filter.vi"("VISA resource name"=w210, "Input Source"="2B Input Connection (0: Single-Ended)", "OE1022D A/B"=w218, "error in (no error)"=w221) -> ("error out"=w230:errorcluster)  [unwired: 10 in, 1 out]
                }
                frame #3 {
                  n38 = local read "System Stablization (s)"() -> (w249:dbl)
                  n39 = Multiply(x=w249, y=1000) -> (x*y=w251:dbl)
                  n40 = Wait (ms)(milliseconds to wait=w251) -> ()  [unwired: 1 out]
                }
              }
            }
          }
          n41 = flat-sequence {
            tunnel: w56 -> [w289]
            tunnel: [w277] -> w54
            tunnel: w55 -> [w288]
            tunnel: [w265] -> w52
            tunnel: w54 -> [w294]
            tunnel: [w294] -> w53
            tunnel: w52 -> [w293]
            tunnel: [w293] -> w51
            tunnel: w53 -> [w315]
            tunnel: [w314] -> w57
            tunnel: w51 -> [w313]
            tunnel: w57 -> [_]
            frame #0 {
              w264 = u8 0 items=["Fixed", "Linear", "Log"] ("SineOut Mode")
              w266 = u16 0 items=["Internal", "External"] ("Trigger Source (0: Internal)")
              w255 = u8 0 items=["Channel A", "Channel B"] ("OE1022D A/B")
              n42 = call "OE1022D_Configure Trigger.vi"("Trigger Source (0: Internal)"=w266, "error in (no error)   2"=w288, "OE1022D A/B"=w255, "VISA resource name   2"=w289) -> ("error out   2"=w282:errorcluster, "VISA resource name out   2"=w283:refnum<visa-resource-name>)
              n43 = call "OE1022D_Configure Reference Source.vi"("VISA resource name"=w283, "OE1022D A/B"=w255, "Reference Source"="A Reference Source", "error in (no error)"=w282) -> ("VISA resource name out"=w281:refnum<visa-resource-name>, "error out"=w279:errorcluster)  [unwired: 14 in]
              n44 = call "OE1022D_Configure Harmonic.vi"("VISA resource name"=w281, "OE1022D A/B"=w255, "Harmonic 1"="A harmonic 1", "Harmonic 2"="A harmonic 2", "error in (no error)"=w279) -> ("VISA resource name out"=w280:refnum<visa-resource-name>, "error out"=w278:errorcluster)  [unwired: 13 in]
              n45 = call "OE1022D_Configure Sine Out.vi"("VISA resource name"=w280, "SineOut Mode"=w264, "OE1022D A/B"=w255, "Sine Output Amplitude (V)"=sgl 0.001 ("A Sine Output Amplitude (V)"), "error in (no error)"=w278) -> ("VISA resource name out"=w286:refnum<visa-resource-name>, "error out"=w285:errorcluster)  [unwired: 9 in]
              n46 = call "OE1022D_Configure Frequency.vi"("VISA resource name"=w286, "OE1022D A/B"=w255, "Internal Frequency(Hz)"="A frequency", "error in (no error)"=w285) -> ("VISA resource name out"=w276:refnum<visa-resource-name>, "error out"=w273:errorcluster)  [unwired: 14 in]
              n47 = call "OE1022D_Configure Ref Phase Channel A.vi"("VISA resource name"=w276, "Reference Source"="A Reference Source", "Internal Frequency(Hz)"="A frequency", "Auto Phase (T: Enabled)"="auto phase A", "error in (no error)"=w273, "Manual Phase  (degree)"="A reference Manual Phase") -> ("VISA resource name out"=w275:refnum<visa-resource-name>, "error out"=w274:errorcluster)  [unwired: 12 in]
              n48 = call "OE1022D_Configure_Acquisition.vi"("VISA resource name"=w275, "OE1022D A/B"=w255, "Sample time (s)"="A Sample time (s)", "error in (no error)"=w274) -> ("VISA resource name out"=w258:refnum<visa-resource-name>, "error out"=w257:errorcluster)  [unwired: 4 in]
              n49 = call "OE1022D_Configure Sensitivity.vi"("VISA resource name"=w258, "OE1022D A/B"=w255, "Sensitivity"="A Sensitivity", "error in (no error)"=w257) -> ("VISA resource name out"=w262:refnum<visa-resource-name>, "error out"=w261:errorcluster)  [unwired: 14 in]
              n50 = call "OE1022D_Configure Filter.vi"("Low Pass Filter Slope (1: 12dB/oct)"="A Low Pass Filter Slope", "Time Constant (8: 100ms)"="A Time Constant", "error in (no error)"=w261, "Enable Sync Filter (F: Disable)"="Enable Sync Filter A (open when f<200Hz)", "OE1022D A/B"=w255, "VISA resource name"=w262) -> ("error out"=w259:errorcluster, "VISA resource name out"=w260:refnum<visa-resource-name>)  [unwired: 4 in]
              n51 = call "OE1022D_Configure Input Filter.vi"("VISA resource name"=w260, "Input Source"="A Input Connection (0: Single-Ended)", "OE1022D A/B"=w255, "error in (no error)"=w259) -> ("VISA resource name out"=w265:refnum<visa-resource-name>, "error out"=w277:errorcluster)  [unwired: 10 in]
            }
            frame #1 {
              n52 = local read "System Stablization (s)"() -> (w290:dbl)
              n53 = Multiply(x=w290, y=1000) -> (x*y=w292:dbl)
              n54 = Wait (ms)(milliseconds to wait=w292) -> ()  [unwired: 1 out]
            }
            frame #2 {
              w297 = u8 2 items=["TTL Pos", "TTL Neg", "Sine Zero Crossing"] ("External Ref Trigger")
              w310 = u8 0 items=["Fixed", "Linear", "Log"] ("SineOut Mode")
              w316 = u16 0 items=["Internal", "External"] ("Trigger Source (0: Internal)")
              w302 = u8 1 items=["Channel A", "Channel B"] ("OE1022D A/B")
              n55 = call "OE1022D_Configure Trigger.vi"("Trigger Source (0: Internal)"=w316, "error in (no error)   2"=w315, "OE1022D A/B"=w302, "VISA resource name   2"=w313) -> ("error out   2"=w328:errorcluster, "VISA resource name out   2"=w329:refnum<visa-resource-name>)
              n56 = call "OE1022D_Configure Reference Source.vi"("VISA resource name"=w329, "OE1022D A/B"=w302, "error in (no error)"=w328) -> ("VISA resource name out"=w327:refnum<visa-resource-name>, "error out"=w325:errorcluster)  [unwired: 15 in]
              n57 = call "OE1022D_Configure Harmonic.vi"("VISA resource name"=w327, "OE1022D A/B"=w302, "Harmonic 1"="B harmonic 1", "Harmonic 2"="B harmonic 2", "error in (no error)"=w325) -> ("VISA resource name out"=w326:refnum<visa-resource-name>, "error out"=w324:errorcluster)  [unwired: 13 in]
              n58 = call "OE1022D_Configure Sine Out.vi"("VISA resource name"=w326, "SineOut Mode"=w310, "OE1022D A/B"=w302, "Sine Output Amplitude (V)"=sgl 0.001, "error in (no error)"=w324) -> ("VISA resource name out"=w331:refnum<visa-resource-name>, "error out"=w330:errorcluster)  [unwired: 9 in]
              n59 = call "OE1022D_Configure Frequency.vi"("VISA resource name"=w331, "OE1022D A/B"=w302, "Internal Frequency(Hz)"="B frequency", "error in (no error)"=w330) -> ("VISA resource name out"=w323:refnum<visa-resource-name>, "error out"=w320:errorcluster)  [unwired: 14 in]
              n60 = call "OE1022D_Configure Ref Phase Channel B.vi"("VISA resource name"=w323, "Reference Source"="B Reference Source", "External Ref Trigger"=w297, "Internal Frequency(Hz)"="B frequency", "Auto Phase (T: Enabled)"="auto phase B", "error in (no error)"=w320, "Manual Phase  (degree)"="B reference Manual Phase") -> ("VISA resource name out"=w322:refnum<visa-resource-name>, "error out"=w321:errorcluster)  [unwired: 11 in]
              n61 = call "OE1022D_Configure_Acquisition.vi"("VISA resource name"=w322, "OE1022D A/B"=w302, "Sample time (s)"="B Sample time (s)", "error in (no error)"=w321) -> ("VISA resource name out"=w303:refnum<visa-resource-name>, "error out"=w304:errorcluster)  [unwired: 4 in]
              n62 = call "OE1022D_Configure Sensitivity.vi"("VISA resource name"=w303, "OE1022D A/B"=w302, "Sensitivity"="B Sensitivity", "error in (no error)"=w304) -> ("VISA resource name out"=w307:refnum<visa-resource-name>, "error out"=w306:errorcluster)  [unwired: 14 in]
              n63 = call "OE1022D_Configure Filter.vi"("Low Pass Filter Slope (1: 12dB/oct)"="B Low Pass Filter Slope", "Time Constant (8: 100ms)"="B Time Constant", "error in (no error)"=w306, "Enable Sync Filter (F: Disable)"="Enable Sync Filter B (open when f<200Hz)", "OE1022D A/B"=w302, "VISA resource name"=w307) -> ("error out"=w305:errorcluster, "VISA resource name out"=w295:refnum<visa-resource-name>)  [unwired: 4 in]
              n64 = call "OE1022D_Configure Input Filter.vi"("VISA resource name"=w295, "Input Source"="B Input Connection (0: Single-Ended)", "OE1022D A/B"=w302, "error in (no error)"=w305) -> ("error out"=w314:errorcluster)  [unwired: 10 in, 1 out]
            }
            frame #3 {
              n65 = local read "System Stablization (s)"() -> (w333:dbl)
              n66 = Multiply(x=w333, y=1000) -> (x*y=w335:dbl)
              n67 = Wait (ms)(milliseconds to wait=w335) -> ()  [unwired: 1 out]
            }
          }
          n68 = local read "Current measurement?"() -> (w46:bool)
          n69 = case shown="True" w46 {
            frame False {
            }
            frame True {
              n70 = local read "LOCKIN3 address"() -> (w58:refnum<visa-resource-name>)
              n71 = call "OE1022D_OpenDevice.vi"("VISA resource name"=w58) -> ("VISA资源名称输出"=w61:refnum<visa-resource-name>, "错误输出"=w62:errorcluster)  [unwired: 17 in]
              n72 = call "OE1022D_Abort.vi"("error in (no error)"=w62, "VISA resource name"=w61) -> ("error out"=w59:errorcluster, "VISA resource name out"=w60:refnum<visa-resource-name>)
              n73 = flat-sequence {
                tunnel: w60 -> [w107]
                tunnel: [w95] -> w67
                tunnel: w59 -> [w106]
                tunnel: [w84] -> w66
                tunnel: w67 -> [w112]
                tunnel: [w112] -> w65
                tunnel: w66 -> [w111]
                tunnel: [w111] -> w64
                tunnel: w65 -> [w134]
                tunnel: [w133] -> w63
                tunnel: w64 -> [w132]
                tunnel: w63 -> [_]
                frame #0 {
                  w105 = u16 1 items=["Single-Ended Voltage", "Differential Voltage", "1 MOhm Current Gain", "100 MOhm Current Gain"] ("2A Input Connection (0: Single-Ended)  2")
                  w72 = u8 2 items=["6 dB/oct", "12 dB/oct", "18 db/oct", "24 dB/oct"] ("2A Low Pass Filter Slope 2")
                  w90 = u8 0 items=["External", "Internal", "Internal Sweep"] ("2A Reference Source 2")
                  w85 = u16 1 items=["Internal", "External"] ("Trigger Source (0: Internal)")
                  w70 = u8 2 items=["TTL Pos", "TTL Neg", "Sine Zero Crossing"] ("External Ref Trigger")
                  w71 = u8 1 items=["Single", "Loop"] ("Sample Mode (Single/Loop)")
                  w83 = u8 0 items=["Fixed", "Linear", "Log"] ("SineOut Mode")
                  w74 = u8 0 items=["Channel A", "Channel B"] ("OE1022D A/B")
                  n74 = call "OE1022D_Configure Trigger.vi"("Trigger Source (0: Internal)"=w85, "error in (no error)   2"=w106, "OE1022D A/B"=w74, "VISA resource name   2"=w107) -> ("error out   2"=w100:errorcluster, "VISA resource name out   2"=w101:refnum<visa-resource-name>)
                  n75 = call "OE1022D_Configure Reference Source.vi"("VISA resource name"=w101, "OE1022D A/B"=w74, "Reference Source"=w90, "error in (no error)"=w100) -> ("VISA resource name out"=w99:refnum<visa-resource-name>, "error out"=w97:errorcluster)  [unwired: 14 in]
                  n76 = local read "A frequency"() -> (w69:dbl)
                  n77 = call "OE1022D_Configure Harmonic.vi"("VISA resource name"=w99, "OE1022D A/B"=w74, "Harmonic 1"=u8 2 ("2A harmonic 4"), "Harmonic 2"=u8 3 ("2A harmonic 3"), "error in (no error)"=w97) -> ("VISA resource name out"=w98:refnum<visa-resource-name>, "error out"=w96:errorcluster)  [unwired: 13 in]
                  n78 = local read "Enable Sync Filter A (open when f<200Hz)"() -> (w68:bool)
                  n79 = call "OE1022D_Configure Sine Out.vi"("VISA resource name"=w98, "SineOut Mode"=w83, "OE1022D A/B"=w74, "Sine Output Amplitude (V)"=sgl 0.0, "error in (no error)"=w96) -> ("VISA resource name out"=w104:refnum<visa-resource-name>, "error out"=w103:errorcluster)  [unwired: 9 in]
                  n80 = call "OE1022D_Configure Frequency.vi"("VISA resource name"=w104, "OE1022D A/B"=w74, "Internal Frequency(Hz)"=w69, "error in (no error)"=w103) -> ("VISA resource name out"=w94:refnum<visa-resource-name>, "error out"=w91:errorcluster)  [unwired: 14 in]
                  n81 = call "OE1022D_Configure Ref Phase Channel A.vi"("VISA resource name"=w94, "Reference Source"=w90, "External Ref Trigger"=w70, "Internal Frequency(Hz)"=w69, "Auto Phase (T: Enabled)"=TRUE ("auto phase 2A 2"), "error in (no error)"=w91, "Manual Phase  (degree)"=0.0 ("2A reference Manual Phase 2")) -> ("VISA resource name out"=w93:refnum<visa-resource-name>, "error out"=w92:errorcluster)  [unwired: 11 in]
                  n82 = call "OE1022D_Configure_Acquisition.vi"("VISA resource name"=w93, "OE1022D A/B"=w74, "Sample time (s)"=0.001 ("2A Sample time (s) 2"), "error in (no error)"=w92, "Sample Mode (Single/Loop)"=w71) -> ("VISA resource name out"=w77:refnum<visa-resource-name>, "error out"=w76:errorcluster)  [unwired: 3 in]
                  n83 = call "OE1022D_Configure Sensitivity.vi"("VISA resource name"=w77, "OE1022D A/B"=w74, "Sensitivity"="R1 Current sensitivity", "error in (no error)"=w76) -> ("VISA resource name out"=w81:refnum<visa-resource-name>, "error out"=w80:errorcluster)  [unwired: 14 in]
                  n84 = call "OE1022D_Configure Filter.vi"("Low Pass Filter Slope (1: 12dB/oct)"=w72, "Time Constant (8: 100ms)"="R1 Current T Constant", "error in (no error)"=w80, "Enable Sync Filter (F: Disable)"=w68, "OE1022D A/B"=w74, "VISA resource name"=w81) -> ("error out"=w78:errorcluster, "VISA resource name out"=w79:refnum<visa-resource-name>)  [unwired: 4 in]
                  n85 = call "OE1022D_Configure Input Filter.vi"("VISA resource name"=w79, "Input Source"=w105, "OE1022D A/B"=w74, "error in (no error)"=w78) -> ("VISA resource name out"=w84:refnum<visa-resource-name>, "error out"=w95:errorcluster)  [unwired: 10 in]
                }
                frame #1 {
                  n86 = local read "System Stablization (s)"() -> (w108:dbl)
                  n87 = Multiply(x=w108, y=1000) -> (x*y=w110:dbl)
                  n88 = Wait (ms)(milliseconds to wait=w110) -> ()  [unwired: 1 out]
                }
                frame #2 {
                  w117 = u8 2 items=["6 dB/oct", "12 dB/oct", "18 db/oct", "24 dB/oct"] ("2B Low Pass Filter Slope 2")
                  w151 = u16 1 items=["Single-Ended Voltage", "Differential Voltage", "1 MOhm Current Gain", "100 MOhm Current Gain"] ("2B Input Connection (0: Single-Ended) 2")
                  w138 = u8 0 items=["External", "Internal", "Internal Sweep", "Channel-A"] ("2B Reference Source 2")
                  w116 = u8 1 items=["Single", "Loop"] ("Sample Mode (Single/Loop)")
                  w118 = u8 2 items=["TTL Pos", "TTL Neg", "Sine Zero Crossing"] ("External Ref Trigger")
                  w129 = u8 0 items=["Fixed", "Linear", "Log"] ("SineOut Mode")
                  w135 = u16 0 items=["Internal", "External"] ("Trigger Source (0: Internal)")
                  w121 = u8 1 items=["Channel A", "Channel B"] ("OE1022D A/B")
                  n89 = call "OE1022D_Configure Trigger.vi"("Trigger Source (0: Internal)"=w135, "error in (no error)   2"=w134, "OE1022D A/B"=w121, "VISA resource name   2"=w132) -> ("error out   2"=w147:errorcluster, "VISA resource name out   2"=w148:refnum<visa-resource-name>)
                  n90 = call "OE1022D_Configure Reference Source.vi"("VISA resource name"=w148, "OE1022D A/B"=w121, "error in (no error)"=w147) -> ("VISA resource name out"=w146:refnum<visa-resource-name>, "error out"=w144:errorcluster)  [unwired: 15 in]
                  n91 = local read "2A frequency"() -> (w114:dbl)
                  n92 = call "OE1022D_Configure Harmonic.vi"("VISA resource name"=w146, "OE1022D A/B"=w121, "Harmonic 1"=u8 2 ("2B harmonic 4"), "Harmonic 2"=u8 3 ("2B harmonic 3"), "error in (no error)"=w144) -> ("VISA resource name out"=w145:refnum<visa-resource-name>, "error out"=w143:errorcluster)  [unwired: 13 in]
                  n93 = call "OE1022D_Configure Sine Out.vi"("VISA resource name"=w145, "SineOut Mode"=w129, "OE1022D A/B"=w121, "Sine Output Amplitude (V)"=sgl 0.0, "error in (no error)"=w143) -> ("VISA resource name out"=w150:refnum<visa-resource-name>, "error out"=w149:errorcluster)  [unwired: 9 in]
                  n94 = call "OE1022D_Configure Frequency.vi"("VISA resource name"=w150, "OE1022D A/B"=w121, "Internal Frequency(Hz)"=w114, "error in (no error)"=w149) -> ("VISA resource name out"=w142:refnum<visa-resource-name>, "error out"=w139:errorcluster)  [unwired: 14 in]
                  n95 = local read "Enable Sync Filter 2A (open when f<200Hz)"() -> (w113:bool)
                  n96 = call "OE1022D_Configure Ref Phase Channel B.vi"("VISA resource name"=w142, "Reference Source"=w138, "External Ref Trigger"=w118, "Internal Frequency(Hz)"=w114, "Auto Phase (T: Enabled)"=TRUE ("auto phase 2B 2"), "error in (no error)"=w139, "Manual Phase  (degree)"=0.0 ("2B reference Manual Phase 2")) -> ("VISA resource name out"=w141:refnum<visa-resource-name>, "error out"=w140:errorcluster)  [unwired: 11 in]
                  n97 = call "OE1022D_Configure_Acquisition.vi"("VISA resource name"=w141, "OE1022D A/B"=w121, "Sample time (s)"=0.001 ("2B Sample time (s) 2"), "error in (no error)"=w140, "Sample Mode (Single/Loop)"=w116) -> ("VISA resource name out"=w122:refnum<visa-resource-name>, "error out"=w123:errorcluster)  [unwired: 3 in]
                  n98 = call "OE1022D_Configure Sensitivity.vi"("VISA resource name"=w122, "OE1022D A/B"=w121, "Sensitivity"="R2 Sensitivity", "error in (no error)"=w123) -> ("VISA resource name out"=w126:refnum<visa-resource-name>, "error out"=w125:errorcluster)  [unwired: 14 in]
                  n99 = call "OE1022D_Configure Filter.vi"("Low Pass Filter Slope (1: 12dB/oct)"=w117, "Time Constant (8: 100ms)"="R2 Current T Constant", "error in (no error)"=w125, "Enable Sync Filter (F: Disable)"=w113, "OE1022D A/B"=w121, "VISA resource name"=w126) -> ("error out"=w124:errorcluster, "VISA resource name out"=w115:refnum<visa-resource-name>)  [unwired: 4 in]
                  n100 = call "OE1022D_Configure Input Filter.vi"("VISA resource name"=w115, "Input Source"=w151, "OE1022D A/B"=w121, "error in (no error)"=w124) -> ("error out"=w133:errorcluster)  [unwired: 10 in, 1 out]
                }
                frame #3 {
                  n101 = local read "System Stablization (s)"() -> (w152:dbl)
                  n102 = Multiply(x=w152, y=1000) -> (x*y=w154:dbl)
                  n103 = Wait (ms)(milliseconds to wait=w154) -> ()  [unwired: 1 out]
                }
              }
            }
          }
        }
        frame #1 {
          n104 = case shown="True" "Sweep T/F" {
            tunnel: w344 -> [w350 w963]
            tunnel: w342 -> [w360 w959]
            tunnel: w341 -> [w361 w958]
            tunnel: [w356 w951] -> w340
            tunnel: [w355 w950] -> w339
            tunnel: w338 -> [w345 w939]
            tunnel: w337 -> [_ w938]
            tunnel: w336 -> [_ w937]
            frame False {
              n105 = Subtract(x="High Value (Oe)", y="Low Value (Oe)") -> (x-y=w354:dbl)
              n106 = Divide(x=w354, y="Step(Oe)") -> (x/y=w353:dbl)
              n107 = call "SetTemperature.vi"("Approach"="Fixed Temperature Approach", "Rate"="FIxed T  Rate (K/min)", "Temperature"="Set Fixed T", "error in (no error)"=w361, "Instrument Ref In"=w360) -> ("error out"=w362:errorcluster, "Instrument Ref Out"=w363:refnum<k24>)  [unwired: 2 in, 1 out]
              n108 = local read "T Delay"() -> (w347:dbl)
              n109 = Multiply(x=w350, y=w353) -> (x*y=w352:dbl)
              n110 = call "WaitFor.vi"("Delay"=w347, "Wait For Temperature"=TRUE ("WaitForTemperature"), "error in (no error)"=w362, "Instrument Ref In"=w363) -> ("error out"=w359:errorcluster, "Instrument Ref Out"=w358:refnum<k24>)  [unwired: 6 in]
              n111 = Increment(x=w352) -> (x+1=w351:dbl)
              n112 = for {
                N: w351 -> [_]
                tunnel: "Step(Oe)" -> [w376]
                tunnel: w353 -> [w374]
                tunnel: "Low Value (Oe)" -> [w377]
                tunnel: "High Value (Oe)" -> [w375]
                tunnel: w358 -> [w371]
                tunnel: w359 -> [w370]
                shift-right: [w369] -> w356
                shift-left: _ -> [_]
                tunnel: [w368] -> w355
                tunnel: w345 -> [w367]
                i -> [w373]
                n113 = Less Or Equal?(x=w373, y=w374) -> (x <= y?=w378:bool)
                n114 = case shown="False" w378 {
                  selector: w378 -> [w379 w405]
                  tunnel: w377 -> [w381 w410]
                  tunnel: w373 -> [w390 w409]
                  tunnel: w376 -> [w389 w408]
                  tunnel: [w387 w406] -> w372
                  tunnel: w375 -> [w388 _]
                  tunnel: w374 -> [w383 _]
                  tunnel: w373 -> [w386 _]
                  frame False {
                    n115 = local write "Forward"(w379) -> ()
                    n116 = Not(x=w379) -> (.not. x?=w380:bool)
                    n117 = Multiply(x=w383, y=2) -> (x*y=w382:dbl)
                    n118 = Less Or Equal?(x=w386, y=w382) -> (x <= y?=w384:bool)
                    n119 = local write "Backward"(w380) -> ()
                    n120 = case shown="False" w384 {
                      tunnel: w390 -> [w397 w404]
                      tunnel: w389 -> [w395 w402]
                      tunnel: w388 -> [_ w400]
                      tunnel: [w393 w399] -> w387
                      tunnel: w383 -> [_ w398]
                      tunnel: w382 -> [w392 _]
                      tunnel: w381 -> [w391 _]
                      frame False {
                        n121 = Subtract(x=w397, y=w392) -> (x-y=w396:dbl)
                        n122 = Multiply(x=w395, y=w396) -> (x*y=w394:dbl)
                        n123 = Add(x=w391, y=w394) -> (x+y=w393:dbl)
                      }
                      frame True {
                        n124 = Subtract(x=w404, y=w398) -> (x-y=w403:dbl)
                        n125 = Multiply(x=w402, y=w403) -> (x*y=w401:dbl)
                        n126 = Subtract(x=w400, y=w401) -> (x-y=w399:dbl)
                      }
                    }
                  }
                  frame True {
                    n127 = Multiply(x=w408, y=w409) -> (x*y=w407:i32)
                    n128 = local write "Forward"(w405) -> ()
                    n129 = Add(x=w410, y=w407) -> (x+y=w406:dbl)
                  }
                }
                n130 = stacked-sequence {
                  tunnel: w372 -> [w416 _ _]
                  tunnel: w371 -> [w415 _ _]
                  tunnel: w370 -> [w414 _ _]
                  tunnel: [w413 _ _] -> w369
                  tunnel: [w412 _ _] -> w368
                  tunnel: w367 -> [_ _ w450]
                  frame #0 {
                    n131 = local read "F Delay"() -> (w411:dbl)
                    n132 = call "SetField.vi"("Mode"="Sweep F mode", "Approach"="Sweep Field Approach", "Rate"="Sweep F Rate (Oe/s)", "Field"=w416, "error in (no error)"=w414, "Instrument Ref In"=w415) -> ("error out"=w420:errorcluster, "Instrument Ref Out"=w421:refnum<k24>)  [unwired: 1 in, 1 out]
                    n133 = call "WaitFor.vi"("Delay"=w411, "Wait For Field"=TRUE, "error in (no error)"=w420, "Instrument Ref In"=w421) -> ("error out"=w418:errorcluster, "Instrument Ref Out"=w417:refnum<k24>)  [unwired: 6 in]
                    n134 = for {
                      N: 20 -> [_]
                      shift-right: [w446] -> _
                      shift-left: TRUE -> [w444]
                      shift-right: [w441] -> w413
                      shift-left: w418 -> [w443]
                      tunnel: w417 -> [w440]
                      tunnel: [w438] -> w412
                      tunnel: [w435] -> w431
                      tunnel: [w434] -> w430
                      tunnel: [w436] -> w428 mode=indexing
                      tunnel: [w437] -> w429 mode=indexing
                      n135 = Not(x=w444) -> (.not. x?=w446:bool)
                      n136 = local write "Measuring F"(w444) -> ()
                      n137 = Wait (ms)(milliseconds to wait=u32 200) -> ()  [unwired: 1 out]
                      n138 = call "GetTemperature.vi"("error in (no error)"=w443, "Instrument Ref In"=w440) -> ("Temperature\nStatus"=w434:i32, "Temperature"=w437:dbl, "error out"=w442:errorcluster, "Instrument Ref Out"=w439:refnum<k24>)  [unwired: 3 in, 1 out]
                      n139 = call "GetField.vi"("error in (no error)"=w442, "Instrument Ref In"=w439) -> ("Field\nStatus"=w435:i32, "Field"=w436:dbl, "error out"=w441:errorcluster, "Instrument Ref Out"=w438:refnum<k24>)  [unwired: 3 in, 1 out]
                    }
                    "Field Status" <- w431
                    "Temperature Status" <- w430
                    n140 = call-poly <vilib>:"Mean.vi"("X"=w428) -> ("mean"=→"Measured Field":dbl)  [unwired: 1 out]
                    n141 = call-poly <vilib>:"Mean.vi"("X"=w429) -> ("mean"=→"Fixed Temperature":dbl)  [unwired: 1 out]
                    "Field Setting" <- w416
                    "Measuring F" <- FALSE
                  }
                  frame #1 {
                    n142 = local read "System Stablization (s)"() -> (w447:dbl)
                    n143 = Multiply(x=w447, y=1000) -> (x*y=w449:dbl)
                    n144 = Wait (ms)(milliseconds to wait=w449) -> ()  [unwired: 1 out]
                  }
                  frame #2 {
                    n145 = local read "V Loop#"() -> (w451:i32)
                    n146 = for {
                      N: w451 -> [_]
                      shift-right: [w468] -> _
                      shift-left: _ -> [w467]
                      shift-right: [w466] -> _
                      shift-left: _ -> [w465]
                      shift-right: [w464] -> _
                      shift-left: _ -> [w462]
                      shift-right: [w463] -> _
                      shift-left: _ -> [w461]
                      shift-right: [w460] -> _
                      shift-left: _ -> [w458]
                      shift-right: [w459] -> _
                      shift-left: _ -> [w457]
                      shift-right: [w456] -> _
                      shift-left: _ -> [w454]
                      shift-right: [w455] -> _
                      shift-left: _ -> [w453]
                      tunnel: w450 -> [w452]
                      i -> [w481]
                      n147 = local read "High Value (V)"() -> (w471:dbl)
                      n148 = local read "Low Value (V)"() -> (w470:dbl)
                      n149 = local read "V Step(mV)"() -> (w469:i32)
                      n150 = Subtract(x=w471, y=w470) -> (x-y=w476:dbl)
                      n151 = Add(x=0, y=w481) -> (x+y=→"V Loop Run F":i32)
                      n152 = Divide(x=w469, y=1000) -> (x/y=w473:dbl)
                      n153 = Divide(x=w476, y=w473) -> (x/y=w472:dbl)
                      n154 = Multiply(x=2, y=w472) -> (x*y=w475:dbl)
                      n155 = Increment(x=w475) -> (x+1=w474:dbl)
                      n156 = for {
                        N: w474 -> [_]
                        tunnel: w470 -> [w516]
                        tunnel: w471 -> [w514]
                        tunnel: w473 -> [w515]
                        tunnel: w472 -> [w518]
                        shift-right: [w502] -> _
                        shift-left: _ -> [w501]
                        shift-right: [w500] -> w468
                        shift-left: w467 -> [w499]
                        shift-right: [w498] -> w466
                        shift-left: w465 -> [w497]
                        shift-right: [w496] -> w464
                        shift-left: w462 -> [w494]
                        shift-right: [w495] -> w463
                        shift-left: w461 -> [w493]
                        shift-right: [w492] -> _
                        shift-left: _ -> [w491]
                        shift-right: [w490] -> w460
                        shift-left: w458 -> [w488]
                        shift-right: [w489] -> w459
                        shift-left: w457 -> [w487]
                        shift-right: [w486] -> w456
                        shift-left: w454 -> [w484]
                        shift-right: [w485] -> w455
                        shift-left: w453 -> [w483]
                        tunnel: w452 -> [w482]
                        i -> [w517]
                        n157 = Less Or Equal?(x=w517, y=w518) -> (x <= y?=w519:bool)
                        n158 = case shown="False" w519 {
                          tunnel: w516 -> [w885 w913]
                          tunnel: w517 -> [w894 w912]
                          tunnel: w515 -> [w893 w911]
                          tunnel: [w891 w909] -> w520
                          tunnel: w514 -> [w892 _]
                          tunnel: w518 -> [w887 _]
                          tunnel: w517 -> [w890 _]
                          frame False {
                            n159 = Multiply(x=w887, y=2) -> (x*y=w886:dbl)
                            n160 = Less Or Equal?(x=w890, y=w886) -> (x <= y?=w888:bool)
                            n161 = case shown="False" w888 {
                              tunnel: w894 -> [w901 w908]
                              tunnel: w893 -> [w899 w906]
                              tunnel: w892 -> [_ w904]
                              tunnel: [w897 w903] -> w891
                              tunnel: w887 -> [_ w902]
                              tunnel: w886 -> [w896 _]
                              tunnel: w885 -> [w895 _]
                              frame False {
                                n162 = Subtract(x=w901, y=w896) -> (x-y=w900:dbl)
                                n163 = Multiply(x=w899, y=w900) -> (x*y=w898:dbl)
                                n164 = Add(x=w895, y=w898) -> (x+y=w897:dbl)
                              }
                              frame True {
                                n165 = Subtract(x=w908, y=w902) -> (x-y=w907:dbl)
                                n166 = Multiply(x=w906, y=w907) -> (x*y=w905:dbl)
                                n167 = Subtract(x=w904, y=w905) -> (x-y=w903:dbl)
                              }
                            }
                          }
                          frame True {
                            n168 = Multiply(x=w911, y=w912) -> (x*y=w910:dbl)
                            n169 = Add(x=w913, y=w910) -> (x+y=w909:dbl)
                          }
                        }
                        n170 = Absolute Value(x=w520) -> (abs(x)=w513:dbl)
                        n171 = stacked-sequence {
                          tunnel: w513 -> [w524 _ _]
                          tunnel: [_ _ w554] -> w510
                          tunnel: [_ _ w561] -> w509
                          tunnel: [_ _ w560] -> w508
                          tunnel: [_ _ w559] -> w507
                          tunnel: [_ _ w558] -> w506
                          tunnel: [_ _ w557] -> w505
                          tunnel: [_ _ w556] -> w504
                          tunnel: [_ _ w555] -> w503
                          tunnel: [_ _ w553] -> w502
                          tunnel: w501 -> [_ _ w552]
                          tunnel: [_ _ w551] -> w500
                          tunnel: w499 -> [_ _ w550]
                          tunnel: [_ _ w549] -> w498
                          tunnel: w497 -> [_ _ w548]
                          tunnel: [_ _ w547] -> w496
                          tunnel: [_ _ w546] -> w495
                          tunnel: w494 -> [_ _ w545]
                          tunnel: w493 -> [_ _ w533]
                          tunnel: [_ _ w544] -> w492
                          tunnel: w491 -> [_ _ w543]
                          tunnel: [_ _ w542] -> w490
                          tunnel: [_ _ w541] -> w489
                          tunnel: w488 -> [_ _ w540]
                          tunnel: w487 -> [_ _ w539]
                          tunnel: [_ _ w538] -> w486
                          tunnel: [_ _ w537] -> w485
                          tunnel: w484 -> [_ _ w536]
                          tunnel: w483 -> [_ _ w535]
                          frame #0 {
                            n172 = Format Into String(format string="SLVLD1,%.3f;", w524) -> (resulting string=w525:string)  [unwired: 2 in, 1 out]
                            n173 = local read "LOCKIN1 address"() -> (w523:refnum<visa-resource-name>)
                            n174 = Concatenate Strings(w525, "\r") -> (w522:string)
                            n175 = local read "Two Devices ?"() -> (w521:bool)
                            n176 = VISA Write(VISA resource name=w523, write buffer=w522) -> ()  [unwired: 1 in, 3 out]
                            n177 = case shown="True" w521 {
                              tunnel: w522 -> [_ w529]
                              frame False {
                              }
                              frame True {
                                n178 = local read "LOCKIN2 address"() -> (w528:refnum<visa-resource-name>)
                                n179 = VISA Write(VISA resource name=w528, write buffer=w529) -> ()  [unwired: 1 in, 3 out]
                              }
                            }
                            "Sine voltage F" <- w524
                          }
                          frame #1 {
                            n180 = local read "System Stablization (s)"() -> (w530:dbl)
                            n181 = Multiply(x=w530, y=1000) -> (x*y=w532:dbl)
                            n182 = Wait (ms)(milliseconds to wait=w532) -> ()  [unwired: 1 out]
                          }
                          frame #2 {
                            n183 = local read "LOCKIN2 address"() -> (w534:refnum<visa-resource-name>)
                            n184 = local read "LOCKIN1 address"() -> (w564:refnum<visa-resource-name>)
                            n185 = local read "Two Devices ?"() -> (w563:bool)
                            n186 = local read "Sine voltage F"() -> (w562:dbl)
                            n187 = case shown="True" w563 {
                              tunnel: [w614 w635] -> w558
                              tunnel: [w614 w634] -> w557
                              tunnel: [w614 w633] -> w555
                              tunnel: [w614 w632] -> w556
                              tunnel: [w617 w631] -> w537
                              tunnel: [w619 w630] -> w544
                              tunnel: w543 -> [w619 w629]
                              tunnel: w535 -> [w617 w626]
                              tunnel: [w618 w628] -> w542
                              tunnel: w540 -> [w618 w627]
                              tunnel: [w616 w625] -> w541
                              tunnel: w539 -> [w616 w624]
                              tunnel: [w615 w623] -> w538
                              tunnel: w536 -> [w615 w622]
                              tunnel: w562 -> [_ w621]
                              tunnel: w534 -> [_ w620]
                              frame False {
                                w614 = nan
                              }
                              frame True {
                                n188 = flat-sequence {
                                tunnel: w629 -> [w712]
                                tunnel: [w710] -> w684
                                tunnel: [w703] -> w683
                                tunnel: [w704] -> w682
                                tunnel: [w701] -> w681
                                tunnel: [w704] -> w680
                                tunnel: [w704] -> w679
                                tunnel: [w704] -> w678
                                tunnel: [w704] -> w677
                                tunnel: [w703] -> w676
                                tunnel: [w702] -> w675
                                tunnel: [w701] -> w674
                                tunnel: [w700] -> w673
                                tunnel: ["F Clear Plot 2B"] -> w672
                                tunnel: ["F Clear Plot 2A"] -> w671
                                tunnel: [w691] -> w670
                                tunnel: [w693] -> w669
                                tunnel: [w692] -> w668
                                tunnel: [w697] -> w667
                                tunnel: [w696] -> w666
                                tunnel: w627 -> [w688]
                                tunnel: w624 -> [w687]
                                tunnel: w621 -> [w686]
                                tunnel: w620 -> [w685]
                                tunnel: w684 -> [w734]
                                tunnel: [w734] -> w665
                                tunnel: w683 -> [w733]
                                tunnel: [w733] -> w664
                                tunnel: w682 -> [w732]
                                tunnel: [w732] -> w663
                                tunnel: w681 -> [w731]
                                tunnel: [w731] -> w662
                                tunnel: w680 -> [w730]
                                tunnel: [w730] -> w661
                                tunnel: w679 -> [w729]
                                tunnel: [w729] -> w660
                                tunnel: w678 -> [w728]
                                tunnel: [w728] -> w659
                                tunnel: w677 -> [w727]
                                tunnel: [w727] -> w658
                                tunnel: w676 -> [w726]
                                tunnel: [w726] -> w657
                                tunnel: w675 -> [w725]
                                tunnel: [w725] -> w656
                                tunnel: w674 -> [w724]
                                tunnel: [w724] -> w655
                                tunnel: w673 -> [w723]
                                tunnel: [w723] -> w654
                                tunnel: w672 -> [w722]
                                tunnel: [w722] -> w653
                                tunnel: w671 -> [w721]
                                tunnel: [w721] -> w652
                                tunnel: w670 -> [w720]
                                tunnel: [w720] -> w651
                                tunnel: w669 -> [w719]
                                tunnel: [w719] -> w650
                                tunnel: w668 -> [w718]
                                tunnel: [w718] -> w649
                                tunnel: w667 -> [w717]
                                tunnel: [w717] -> w648
                                tunnel: w666 -> [w716]
                                tunnel: [w716] -> w647
                                tunnel: w665 -> [w739]
                                tunnel: w664 -> [w772]
                                tunnel: w663 -> [w771]
                                tunnel: w662 -> [w770]
                                tunnel: w661 -> [w769]
                                tunnel: w660 -> [w767]
                                tunnel: w659 -> [w765]
                                tunnel: w658 -> [w763]
                                tunnel: w657 -> [w760]
                                tunnel: w656 -> [w759]
                                tunnel: w655 -> [w756]
                                tunnel: w654 -> [w755]
                                tunnel: w653 -> [w753]
                                tunnel: w622 -> [w751]
                                tunnel: w652 -> [w750]
                                tunnel: w651 -> [w746]
                                tunnel: w650 -> [w745]
                                tunnel: w649 -> [w744]
                                tunnel: w648 -> [w741]
                                tunnel: w647 -> [w740]
                                tunnel: [w739] -> w646
                                tunnel: [w758] -> w645
                                tunnel: [w772] -> w644
                                tunnel: [w771] -> w643
                                tunnel: [w737] -> w642
                                tunnel: [w738] -> w641
                                tunnel: [w761] -> w640
                                tunnel: [w757] -> w639
                                tunnel: [w754] -> w638
                                tunnel: [w770] -> w637
                                tunnel: [w743] -> w636
                                tunnel: w626 -> [w735]
                                tunnel: [w775] -> w632
                                tunnel: [w776] -> w634
                                tunnel: [w777] -> w625
                                tunnel: [w778] -> w631
                                tunnel: [w779] -> w623
                                tunnel: [w780] -> _
                                tunnel: [w781] -> w633
                                tunnel: [w782] -> w630
                                tunnel: [w783] -> w628
                                tunnel: [w784] -> _
                                tunnel: w646 -> [w784]
                                tunnel: w645 -> [w783]
                                tunnel: w644 -> [w773]
                                tunnel: w643 -> [w782]
                                tunnel: w642 -> [w781]
                                tunnel: w641 -> [w780]
                                tunnel: w640 -> [w779]
                                tunnel: w639 -> [w778]
                                tunnel: w638 -> [w777]
                                tunnel: w637 -> [w776]
                                tunnel: w636 -> [w775]
                                tunnel: [w773] -> w635
                                frame #0 {
                                w693 = u8 1 items=["Channel A", "Channel B"] ("Channel A/B for Parameter1")
                                w696 = u8 0 items=["Channel A", "Channel B"] ("Channel A/B for Parameter1")
                                n189 = Format Into String(0) -> (error out=w711:errorcluster)  [unwired: 3 in, 1 out]
                                n190 = Format Into String(0) -> (error out=w694:errorcluster)  [unwired: 3 in, 1 out]
                                n191 = call "OE1022D_Read 1 parameter_mean.vi"("错误输入（无错误）"=w711, "Parameter"="Parameter 2A 2", "Channel (0: A)"=w696, "VISA resource name"=w685) -> ("error out"=w697:errorcluster, "Measurement"=w705:dbl, "VISA resource name out"=w710:refnum<visa-resource-name>)  [unwired: 5 in]
                                n192 = call "OE1022D_Read 1 parameter_mean.vi"("Parameter 2"="Parameter 2B 2", "错误输入（无错误）"=w694, "Channel (0: A)"=w693, "VISA resource name"=w685) -> ("error out"=w691:errorcluster, "Measurement"=w690:dbl, "VISA resource name out"=w692:refnum<visa-resource-name>)  [unwired: 5 in]
                                n193 = Multiply(x=w690, y=1000000.0) -> (x*y=w701:dbl)
                                "para2B Measurement 2" <- w701
                                n194 = Multiply(x=w705, y=1000.0) -> (x*y=w703:dbl)
                                "para2A Measurement 2" <- w703
                                n195 = Build Array(w701) -> (w707:dbl[])
                                n196 = Select(t=w707, s="F Clear Plot 2B", f=w687) -> (s? t:f=w700:dbl[])
                                n197 = Build Array(w703) -> (w713:dbl[])
                                n198 = Select(t=w713, s="F Clear Plot 2A", f=w688) -> (s? t:f=w702:dbl[])
                                n199 = Build Array (concatenate)(w686, w712) -> (w704:dbl[])
                                }
                                frame #1 {
                                n200 = Wait (ms)(milliseconds to wait=u32 50) -> ()  [unwired: 1 out]
                                }
                                frame #2 {
                                n201 = Build Array (concatenate)(w760, w759) -> (w758:dbl[])
                                n202 = Build Array (concatenate)(w756, w755) -> (w754:dbl[])
                                n203 = Bundle(w765, w758) -> (→"R2A-F":cluster{dbl[], dbl[]})  [unwired: 1 in]
                                n204 = Bundle(w767, w754) -> (→"R2B-F":cluster{dbl[], dbl[]})  [unwired: 1 in]
                                n205 = call "OE1022D_Read 1 parameter_mean.vi"("错误输入（无错误）"=w741, "Parameter"="Phase 2A  2", "Channel (0: A)"=w740, "VISA resource name"=w739) -> ("error out"=w738:errorcluster, "Measurement"=w737:dbl)  [unwired: 5 in, 1 out]
                                "phase 2A 2" <- w737
                                n206 = Build Array(w737) -> (w747:dbl[])
                                n207 = call "OE1022D_Read 1 parameter_mean.vi"("Parameter 2"="Phase 2B 2", "错误输入（无错误）"=w746, "Channel (0: A)"=w745, "VISA resource name"=w744) -> ("Measurement"=w743:dbl)  [unwired: 5 in, 2 out]
                                "phase 2B 2" <- w743
                                n208 = Select(t=w747, s=w750, f=w751) -> (s? t:f=w749:dbl[])
                                n209 = Build Array(w743) -> (w748:dbl[])
                                n210 = Build Array (concatenate)(w737, w749) -> (w761:dbl[])
                                n211 = Select(t=w748, s=w753, f=w735) -> (s? t:f=w752:dbl[])
                                n212 = Bundle(w763, w761) -> (→"Phase2A-F":cluster{dbl[], dbl[]})  [unwired: 1 in]
                                n213 = Build Array (concatenate)(w743, w752) -> (w757:dbl[])
                                n214 = Bundle(w769, w757) -> (→"Phase2B-F":cluster{dbl[], dbl[]})  [unwired: 1 in]
                                }
                                frame #3 {
                                n215 = Wait (ms)(milliseconds to wait=u32 50) -> ()  [unwired: 1 out]
                                }
                                }
                              }
                            }
                            n216 = flat-sequence {
                              tunnel: w548 -> [w812]
                              tunnel: w552 -> [w811]
                              tunnel: w550 -> [w803]
                              tunnel: [w809] -> w613
                              tunnel: [w797] -> w612
                              tunnel: [w798] -> w611
                              tunnel: [w795] -> w610
                              tunnel: [w798] -> w609
                              tunnel: [w798] -> w608
                              tunnel: [w798] -> w607
                              tunnel: [w798] -> w606
                              tunnel: [w797] -> w605
                              tunnel: [w796] -> w604
                              tunnel: [w795] -> w603
                              tunnel: [w794] -> w602
                              tunnel: ["F Clear Plot 1B"] -> w601
                              tunnel: ["F Clear Plot 1A"] -> w600
                              tunnel: [w791] -> w599
                              tunnel: [w790] -> w598
                              tunnel: [w789] -> w597
                              tunnel: [w788] -> w596
                              tunnel: [w787] -> w595
                              tunnel: w562 -> [w786]
                              tunnel: w564 -> [w785]
                              tunnel: w613 -> [w834]
                              tunnel: [w834] -> w594
                              tunnel: w612 -> [w833]
                              tunnel: [w833] -> w593
                              tunnel: w611 -> [w832]
                              tunnel: [w832] -> w592
                              tunnel: w610 -> [w831]
                              tunnel: [w831] -> w591
                              tunnel: w609 -> [w830]
                              tunnel: [w830] -> w590
                              tunnel: w608 -> [w829]
                              tunnel: [w829] -> w589
                              tunnel: w607 -> [w828]
                              tunnel: [w828] -> w588
                              tunnel: w606 -> [w827]
                              tunnel: [w827] -> w587
                              tunnel: w605 -> [w826]
                              tunnel: [w826] -> w586
                              tunnel: w604 -> [w825]
                              tunnel: [w825] -> w585
                              tunnel: w603 -> [w824]
                              tunnel: [w824] -> w584
                              tunnel: w602 -> [w823]
                              tunnel: [w823] -> w583
                              tunnel: w601 -> [w822]
                              tunnel: [w822] -> w582
                              tunnel: w600 -> [w821]
                              tunnel: [w821] -> w581
                              tunnel: w599 -> [w820]
                              tunnel: [w820] -> w580
                              tunnel: w598 -> [w819]
                              tunnel: [w819] -> w579
                              tunnel: w597 -> [w818]
                              tunnel: [w818] -> w578
                              tunnel: w596 -> [w817]
                              tunnel: [w817] -> w577
                              tunnel: w595 -> [w816]
                              tunnel: [w816] -> w576
                              tunnel: w594 -> [w840]
                              tunnel: w593 -> [w872]
                              tunnel: w592 -> [w871]
                              tunnel: w591 -> [w870]
                              tunnel: w590 -> [w869]
                              tunnel: w589 -> [w867]
                              tunnel: w588 -> [w865]
                              tunnel: w587 -> [w863]
                              tunnel: w586 -> [w860]
                              tunnel: w585 -> [w859]
                              tunnel: w584 -> [w856]
                              tunnel: w583 -> [w855]
                              tunnel: w582 -> [w853]
                              tunnel: w581 -> [w851]
                              tunnel: w580 -> [w847]
                              tunnel: w579 -> [w846]
                              tunnel: w578 -> [w845]
                              tunnel: w577 -> [w842]
                              tunnel: w576 -> [w841]
                              tunnel: [w840] -> w575
                              tunnel: [w858] -> w574
                              tunnel: [w872] -> w573
                              tunnel: [w871] -> w572
                              tunnel: [w838] -> w571
                              tunnel: [w839] -> w570
                              tunnel: [w861] -> w569
                              tunnel: [w857] -> w568
                              tunnel: [w854] -> w567
                              tunnel: [w870] -> w566
                              tunnel: [w844] -> w565
                              tunnel: w545 -> [w836]
                              tunnel: w533 -> [w835]
                              tunnel: [w874] -> w560
                              tunnel: [w875] -> w554
                              tunnel: [w876] -> w551
                              tunnel: [w877] -> w547
                              tunnel: [w878] -> w546
                              tunnel: [w879] -> _
                              tunnel: [w880] -> w559
                              tunnel: [w881] -> w553
                              tunnel: [w882] -> w561
                              tunnel: [w883] -> w549
                              tunnel: [w884] -> _
                              tunnel: w575 -> [w884]
                              tunnel: w574 -> [w883]
                              tunnel: w573 -> [w882]
                              tunnel: w572 -> [w881]
                              tunnel: w571 -> [w880]
                              tunnel: w570 -> [w879]
                              tunnel: w569 -> [w878]
                              tunnel: w568 -> [w877]
                              tunnel: w567 -> [w876]
                              tunnel: w566 -> [w875]
                              tunnel: w565 -> [w874]
                              frame #0 {
                                w790 = u8 1 items=["Channel A", "Channel B"] ("Channel A/B for Parameter1")
                                w787 = u8 0 items=["Channel A", "Channel B"] ("Channel A/B for Parameter1")
                                n217 = Format Into String(0) -> (error out=w805:errorcluster)  [unwired: 3 in, 1 out]
                                n218 = call "OE1022D_Read 1 parameter_mean.vi"("Parameter 2"="Parameter 1B 2", "错误输入（无错误）"=w805, "Channel (0: A)"=w790, "VISA resource name"=w785) -> ("error out"=w791:errorcluster, "Measurement"=w799:dbl, "VISA resource name out"=w789:refnum<visa-resource-name>)  [unwired: 5 in]
                                n219 = Format Into String(0) -> (error out=w810:errorcluster)  [unwired: 3 in, 1 out]
                                n220 = call "OE1022D_Read 1 parameter_mean.vi"("错误输入（无错误）"=w810, "Parameter"="Parameter 1A 2", "Channel (0: A)"=w787, "VISA resource name"=w785) -> ("error out"=w788:errorcluster, "Measurement"=w800:dbl, "VISA resource name out"=w809:refnum<visa-resource-name>)  [unwired: 5 in]
                                n221 = Multiply(x=w799, y=1000000.0) -> (x*y=w795:dbl)
                                "para1B Measurement (uV) 2" <- w795
                                n222 = Multiply(x=w800, y=1000.0) -> (x*y=w797:dbl)
                                "para1A Measurement (mV) 2" <- w797
                                n223 = Build Array(w795) -> (w806:dbl[])
                                n224 = Build Array(w797) -> (w813:dbl[])
                                n225 = Select(t=w806, s="F Clear Plot 1B", f=w803) -> (s? t:f=w794:dbl[])
                                n226 = Select(t=w813, s="F Clear Plot 1A", f=w812) -> (s? t:f=w796:dbl[])
                                n227 = Build Array (concatenate)(w786, w811) -> (w798:dbl[])
                              }
                              frame #1 {
                                n228 = Wait (ms)(milliseconds to wait=u32 50) -> ()  [unwired: 1 out]
                              }
                              frame #2 {
                                n229 = Build Array (concatenate)(w860, w859) -> (w858:dbl[])
                                n230 = Build Array (concatenate)(w856, w855) -> (w854:dbl[])
                                n231 = Bundle(w865, w858) -> (→"R1A-F":cluster{dbl[], dbl[]})  [unwired: 1 in]
                                n232 = Bundle(w867, w854) -> (→"R1B-F":cluster{dbl[], dbl[]})  [unwired: 1 in]
                                n233 = call "OE1022D_Read 1 parameter_mean.vi"("错误输入（无错误）"=w842, "Parameter"="Phase 1A 2", "Channel (0: A)"=w841, "VISA resource name"=w840) -> ("error out"=w839:errorcluster, "Measurement"=w838:dbl)  [unwired: 5 in, 1 out]
                                "phase 1A 2" <- w838
                                n234 = call "OE1022D_Read 1 parameter_mean.vi"("Parameter 2"="Phase 1B 2", "错误输入（无错误）"=w847, "Channel (0: A)"=w846, "VISA resource name"=w845) -> ("Measurement"=w844:dbl)  [unwired: 5 in, 2 out]
                                "phase 1B 2" <- w844
                                n235 = Build Array(w838) -> (w848:dbl[])
                                n236 = Build Array(w844) -> (w849:dbl[])
                                n237 = Select(t=w848, s=w851, f=w835) -> (s? t:f=w850:dbl[])
                                n238 = Select(t=w849, s=w853, f=w836) -> (s? t:f=w852:dbl[])
                                n239 = Build Array (concatenate)(w838, w850) -> (w861:dbl[])
                                n240 = Build Array (concatenate)(w844, w852) -> (w857:dbl[])
                                n241 = Bundle(w863, w861) -> (→"Phase1A-F":cluster{dbl[], dbl[]})  [unwired: 1 in]
                                n242 = Bundle(w869, w857) -> (→"Phase1B-F":cluster{dbl[], dbl[]})  [unwired: 1 in]
                              }
                              frame #3 {
                                n243 = Wait (ms)(milliseconds to wait=u32 50) -> ()  [unwired: 1 out]
                              }
                            }
                          }
                        }
                        n244 = local read "Sine voltage F"() -> (w511:dbl)
                        n245 = local read "Measured Field"() -> (w512:dbl)
                        n246 = case shown="True" w482 {
                          tunnel: w512 -> [_ w919]
                          tunnel: w510 -> [_ w923]
                          tunnel: w509 -> [_ w924]
                          tunnel: w507 -> [_ w922]
                          tunnel: w508 -> [_ w921]
                          tunnel: w511 -> [_ w918]
                          tunnel: w506 -> [_ w917]
                          tunnel: w505 -> [_ w916]
                          tunnel: w504 -> [_ w915]
                          tunnel: w503 -> [_ w914]
                          frame False {
                          }
                          frame True {
                            n247 = Build Array(w919, w918, w924, w922, w923, w921) -> (w926:dbl[])
                            n248 = local read "Two Devices ?"() -> (w920:bool)
                            n249 = case shown="True" w920 {
                              tunnel: w919 -> [_ w933]
                              tunnel: w917 -> [_ w932]
                              tunnel: w916 -> [_ w931]
                              tunnel: w914 -> [_ w930]
                              tunnel: w915 -> [_ w929]
                              tunnel: w918 -> [_ w928]
                              frame False {
                              }
                              frame True {
                                n250 = Build Array(w933, w928, w932, w930, w931, w929) -> (w935:dbl[])
                                n251 = call-poly <vilib>:"Write Delimited Spreadsheet.vi"("format (%.3f)"="%.10f", "1D data"=w935, "append to file? (new file:F)"=TRUE) -> ()  [unwired: 11 in, 2 out]
                              }
                            }
                            n252 = call-poly <vilib>:"Write Delimited Spreadsheet.vi"("format (%.3f)"="%.10f", "1D data"=w926, "append to file? (new file:F)"=TRUE) -> ()  [unwired: 11 in, 2 out]
                          }
                        }
                      }
                    }
                  }
                }
              }
            }
            frame True {
              n253 = local read "F Delay"() -> (w940:dbl)
              n254 = call "SetField.vi"("Mode"="Fixed F mode", "Approach"="Fixed Field Approach", "Rate"="FIxed F Rate (Oe/s)", "Field"="Set FIxed F (Oe)", "error in (no error)"=w958, "Instrument Ref In"=w959) -> ("error out"=w954:errorcluster, "Instrument Ref Out"=w956:refnum<k24>)  [unwired: 1 in, 1 out]
              n255 = Subtract(x="End Value (K)", y="Start Value (K)") -> (x-y=w947:dbl)
              n256 = Divide(x="Step(K)", y=1) -> (x/y=w946:dbl)
              n257 = Divide(x=w947, y=w946) -> (x/y=w945:dbl)
              n258 = call "WaitFor.vi"("Delay"=w940, "Wait For Field"=TRUE, "error in (no error)"=w954, "Instrument Ref In"=w956) -> ("error out"=w955:errorcluster, "Instrument Ref Out"=w957:refnum<k24>)  [unwired: 6 in]
              n259 = Multiply(x=w963, y=w945) -> (x*y=w944:dbl)
              n260 = Increment(x=w944) -> (x+1=w943:dbl)
              n261 = for {
                N: w943 -> [_]
                tunnel: w946 -> [w976]
                tunnel: w945 -> [w974]
                tunnel: "Start Value (K)" -> [w977]
                tunnel: "End Value (K)" -> [w975]
                tunnel: w957 -> [w970]
                tunnel: w955 -> [w969]
                tunnel: [w968] -> w951
                tunnel: [w967] -> w950
                tunnel: w939 -> [w966]
                tunnel: w938 -> [w965]
                tunnel: w937 -> [w964]
                i -> [w973]
                n262 = Less Or Equal?(x=w973, y=w974) -> (x <= y?=w978:bool)
                n263 = case shown="False" w978 {
                  selector: w978 -> [w979 w1005]
                  tunnel: w977 -> [w981 w1010]
                  tunnel: w973 -> [w990 w1009]
                  tunnel: w976 -> [w989 w1008]
                  tunnel: [w987 w1006] -> w972
                  tunnel: w975 -> [w988 _]
                  tunnel: w974 -> [w983 _]
                  tunnel: w973 -> [w986 _]
                  frame False {
                    n264 = local write "Forward"(w979) -> ()
                    n265 = Not(x=w979) -> (.not. x?=w980:bool)
                    n266 = Multiply(x=w983, y=2) -> (x*y=w982:dbl)
                    n267 = Less Or Equal?(x=w986, y=w982) -> (x <= y?=w984:bool)
                    n268 = local write "Backward"(w980) -> ()
                    n269 = case shown="True" w984 {
                      tunnel: w990 -> [w997 w1004]
                      tunnel: w989 -> [w995 w1002]
                      tunnel: w988 -> [_ w1000]
                      tunnel: [w993 w999] -> w987
                      tunnel: w983 -> [_ w998]
                      tunnel: w982 -> [w992 _]
                      tunnel: w981 -> [w991 _]
                      frame False {
                        n270 = Subtract(x=w997, y=w992) -> (x-y=w996:dbl)
                        n271 = Multiply(x=w995, y=w996) -> (x*y=w994:dbl)
                        n272 = Add(x=w991, y=w994) -> (x+y=w993:dbl)
                      }
                      frame True {
                        n273 = Subtract(x=w1004, y=w998) -> (x-y=w1003:dbl)
                        n274 = Multiply(x=w1002, y=w1003) -> (x*y=w1001:dbl)
                        n275 = Subtract(x=w1000, y=w1001) -> (x-y=w999:dbl)
                      }
                    }
                  }
                  frame True {
                    n276 = Multiply(x=w1008, y=w1009) -> (x*y=w1007:dbl)
                    n277 = local write "Forward"(w1005) -> ()
                    n278 = Add(x=w1010, y=w1007) -> (x+y=w1006:dbl)
                  }
                }
                n279 = Absolute Value(x=w972) -> (abs(x)=w971:dbl)
                n280 = stacked-sequence {
                  tunnel: w971 -> [w1029 _ _]
                  tunnel: w970 -> [w1028 _ _]
                  tunnel: w969 -> [w1027 _ _]
                  tunnel: [w1013 _ _] -> w968
                  tunnel: [w1012 _ _] -> w967
                  tunnel: w966 -> [_ _ w1051]
                  tunnel: w965 -> [_ _ w1050]
                  tunnel: w964 -> [_ _ w1049]
                  frame #0 {
                    n281 = local read "T Delay"() -> (w1011:dbl)
                    n282 = call "SetTemperature.vi"("Approach"="Sweep Temperature Approach", "Rate"="Sweep T  Rate (K/min)", "Temperature"=w1029, "error in (no error)"=w1027, "Instrument Ref In"=w1028) -> ("error out"=w1025:errorcluster, "Instrument Ref Out"=w1026:refnum<k24>)  [unwired: 2 in, 1 out]
                    n283 = call "WaitFor.vi"("Delay"=w1011, "Wait For Temperature"=TRUE ("WaitForTemperature"), "error in (no error)"=w1025, "Instrument Ref In"=w1026) -> ("error out"=w1016:errorcluster, "Instrument Ref Out"=w1015:refnum<k24>)  [unwired: 6 in]
                    n284 = for {
                      N: 20 -> [_]
                      shift-right: [w1045] -> _
                      shift-left: TRUE -> [w1043]
                      shift-right: [w1040] -> w1013
                      shift-left: w1016 -> [w1042]
                      tunnel: w1015 -> [w1039]
                      tunnel: [w1037] -> w1012
                      tunnel: [w1034] -> w1022
                      tunnel: [w1033] -> w1021
                      tunnel: [w1035] -> w1019 mode=indexing
                      tunnel: [w1036] -> w1020 mode=indexing
                      n285 = Not(x=w1043) -> (.not. x?=w1045:bool)
                      n286 = local write "Measuring T"(w1043) -> ()
                      n287 = call "GetTemperature.vi"("error in (no error)"=w1042, "Instrument Ref In"=w1039) -> ("Temperature\nStatus"=w1033:i32, "Temperature"=w1036:dbl, "error out"=w1041:errorcluster, "Instrument Ref Out"=w1038:refnum<k24>)  [unwired: 3 in, 1 out]
                      n288 = Wait (ms)(milliseconds to wait=u32 200) -> ()  [unwired: 1 out]
                      n289 = call "GetField.vi"("error in (no error)"=w1041, "Instrument Ref In"=w1038) -> ("Field\nStatus"=w1034:i32, "Field"=w1035:dbl, "error out"=w1040:errorcluster, "Instrument Ref Out"=w1037:refnum<k24>)  [unwired: 3 in, 1 out]
                    }
                    "Field Status" <- w1022
                    "Temperature Status" <- w1021
                    n290 = call-poly <vilib>:"Mean.vi"("X"=w1019) -> ("mean"=→"Fixed Field":dbl)  [unwired: 1 out]
                    n291 = call-poly <vilib>:"Mean.vi"("X"=w1020) -> ("mean"=→"Measured Temp":dbl)  [unwired: 1 out]
                    "Temp Setting" <- w1029
                    "Measuring T" <- FALSE
                  }
                  frame #1 {
                    n292 = local read "System Stablization (s)"() -> (w1046:dbl)
                    n293 = Multiply(x=w1046, y=1000) -> (x*y=w1048:dbl)
                    n294 = Wait (ms)(milliseconds to wait=w1048) -> ()  [unwired: 1 out]
                  }
                  frame #2 {
                    n295 = local read "V Loop#"() -> (w1052:i32)
                    n296 = for {
                      N: w1052 -> [_]
                      shift-right: [w1086] -> _
                      shift-left: _ -> [w1085]
                      shift-right: [w1087] -> _
                      shift-left: _ -> [w1084]
                      shift-right: [w1083] -> _
                      shift-left: _ -> [w1081]
                      shift-right: [w1082] -> _
                      shift-left: _ -> [w1080]
                      shift-right: [w1079] -> _
                      shift-left: _ -> [w1075]
                      shift-right: [w1078] -> _
                      shift-left: _ -> [w1074]
                      shift-right: [w1077] -> _
                      shift-left: _ -> [w1073]
                      shift-right: [w1076] -> _
                      shift-left: _ -> [w1072]
                      tunnel: w1051 -> [w1071]
                      tunnel: w1050 -> [w1070]
                      tunnel: w1049 -> [w1069]
                      shift-right: [w1067] -> _
                      shift-left: _ -> [w1065]
                      shift-right: [w1068] -> _
                      shift-left: _ -> [w1066]
                      shift-right: [w1063] -> _
                      shift-left: _ -> [w1061]
                      shift-right: [w1064] -> _
                      shift-left: _ -> [w1062]
                      shift-right: [w1060] -> _
                      shift-left: _ -> [w1059]
                      shift-right: [w1058] -> _
                      shift-left: _ -> [w1057]
                      shift-right: [w1056] -> _
                      shift-left: _ -> [w1055]
                      shift-right: [w1054] -> _
                      shift-left: _ -> [w1053]
                      i -> [w1100]
                      n297 = local read "V Step(mV)"() -> (w1088:i32)
                      n298 = Add(x=1, y=w1100) -> (x+y=→"V Loop Run T":i32)
                      n299 = local read "High Value (V)"() -> (w1090:dbl)
                      n300 = local read "Low Value (V)"() -> (w1089:dbl)
                      n301 = Subtract(x=w1090, y=w1089) -> (x-y=w1095:dbl)
                      n302 = Divide(x=w1088, y=1000) -> (x/y=w1092:dbl)
                      n303 = Divide(x=w1095, y=w1092) -> (x/y=w1091:dbl)
                      n304 = Multiply(x=2, y=w1091) -> (x*y=w1094:dbl)
                      n305 = Increment(x=w1094) -> (x+1=w1093:dbl)
                      n306 = for {
                        N: w1093 -> [_]
                        tunnel: w1092 -> [w1160]
                        tunnel: w1091 -> [w1162]
                        shift-right: [w1149] -> _
                        shift-left: _ -> [w1146]
                        shift-right: [w1147] -> w1086
                        shift-left: w1085 -> [w1145]
                        shift-right: [w1148] -> w1087
                        shift-left: w1084 -> [w1144]
                        shift-right: [w1143] -> w1083
                        shift-left: w1081 -> [w1141]
                        shift-right: [w1142] -> w1082
                        shift-left: w1080 -> [w1140]
                        shift-right: [w1139] -> _
                        shift-left: _ -> [w1138]
                        shift-right: [w1137] -> w1079
                        shift-left: w1075 -> [w1133]
                        shift-right: [w1136] -> w1078
                        shift-left: w1074 -> [w1130]
                        shift-right: [w1135] -> w1077
                        shift-left: w1073 -> [w1132]
                        shift-right: [w1134] -> w1076
                        shift-left: w1072 -> [w1131]
                        tunnel: w1071 -> [w1129]
                        tunnel: w1070 -> [w1128]
                        tunnel: w1069 -> [w1127]
                        shift-right: [w1123] -> w1067
                        shift-left: w1065 -> [w1122]
                        shift-right: [w1124] -> w1068
                        shift-left: w1066 -> [w1121]
                        shift-right: [w1115] -> w1063
                        shift-left: w1061 -> [w1114]
                        shift-right: [w1116] -> w1064
                        shift-left: w1062 -> [w1113]
                        shift-right: [w1108] -> w1060
                        shift-left: w1059 -> [w1107]
                        shift-right: [w1106] -> w1058
                        shift-left: w1057 -> [w1105]
                        shift-right: [w1104] -> w1056
                        shift-left: w1055 -> [w1103]
                        shift-right: [w1102] -> w1054
                        shift-left: w1053 -> [w1101]
                        i -> [w1161]
                        n307 = local read "High Value (V)"() -> (w1164:dbl)
                        n308 = local read "Low Value (V)"() -> (w1165:dbl)
                        n309 = Less Or Equal?(x=w1161, y=w1162) -> (x <= y?=w1163:bool)
                        n310 = case shown="False" w1163 {
                          tunnel: w1165 -> [w1731 w1759]
                          tunnel: w1161 -> [w1740 w1758]
                          tunnel: w1160 -> [w1739 w1757]
                          tunnel: [w1737 w1755] -> w1159
                          tunnel: w1164 -> [w1738 _]
                          tunnel: w1162 -> [w1733 _]
                          tunnel: w1161 -> [w1736 _]
                          frame False {
                            n311 = Multiply(x=w1733, y=2) -> (x*y=w1732:dbl)
                            n312 = Less Or Equal?(x=w1736, y=w1732) -> (x <= y?=w1734:bool)
                            n313 = case shown="False" w1734 {
                              tunnel: w1740 -> [w1747 w1754]
                              tunnel: w1739 -> [w1745 w1752]
                              tunnel: w1738 -> [_ w1750]
                              tunnel: [w1743 w1749] -> w1737
                              tunnel: w1733 -> [_ w1748]
                              tunnel: w1732 -> [w1742 _]
                              tunnel: w1731 -> [w1741 _]
                              frame False {
                                n314 = Subtract(x=w1747, y=w1742) -> (x-y=w1746:dbl)
                                n315 = Multiply(x=w1745, y=w1746) -> (x*y=w1744:dbl)
                                n316 = Add(x=w1741, y=w1744) -> (x+y=w1743:dbl)
                              }
                              frame True {
                                n317 = Subtract(x=w1754, y=w1748) -> (x-y=w1753:dbl)
                                n318 = Multiply(x=w1752, y=w1753) -> (x*y=w1751:dbl)
                                n319 = Subtract(x=w1750, y=w1751) -> (x-y=w1749:dbl)
                              }
                            }
                          }
                          frame True {
                            n320 = Multiply(x=w1757, y=w1758) -> (x*y=w1756:dbl)
                            n321 = Add(x=w1759, y=w1756) -> (x+y=w1755:dbl)
                          }
                        }
                        n322 = Absolute Value(x=w1159) -> (abs(x)=w1158:dbl)
                        n323 = stacked-sequence {
                          tunnel: w1158 -> [w1169 _ _ _]
                          tunnel: [_ _ w1240 _] -> w1157
                          tunnel: [_ _ w1239 _] -> w1156
                          tunnel: [_ _ w1238 _] -> w1155
                          tunnel: [_ _ w1237 _] -> w1154
                          tunnel: [_ _ w1236 _] -> w1153
                          tunnel: [_ _ w1235 _] -> w1152
                          tunnel: [_ _ w1234 _] -> w1151
                          tunnel: [_ _ w1233 _] -> w1150
                          tunnel: [_ _ w1231 _] -> w1149
                          tunnel: [_ _ w1230 _] -> w1148
                          tunnel: [_ _ w1229 _] -> w1147
                          tunnel: w1146 -> [_ _ w1228 w1707]
                          tunnel: w1145 -> [_ _ w1227 _]
                          tunnel: w1144 -> [_ _ w1226 _]
                          tunnel: [_ _ w1225 _] -> w1143
                          tunnel: [_ _ w1224 _] -> w1142
                          tunnel: w1141 -> [_ _ w1223 _]
                          tunnel: w1140 -> [_ _ w1222 _]
                          tunnel: [_ _ w1221 _] -> w1139
                          tunnel: w1138 -> [_ _ w1220 _]
                          tunnel: [_ _ w1219 _] -> w1137
                          tunnel: [_ _ w1218 _] -> w1136
                          tunnel: [_ _ w1217 _] -> w1135
                          tunnel: [_ _ w1216 _] -> w1134
                          tunnel: w1133 -> [_ _ w1215 _]
                          tunnel: w1132 -> [_ _ w1214 _]
                          tunnel: w1131 -> [_ _ w1213 _]
                          tunnel: w1130 -> [_ _ w1212 _]
                          tunnel: [_ _ w1199 _] -> w1126
                          tunnel: [_ _ w1198 _] -> w1125
                          tunnel: [_ _ w1197 _] -> w1124
                          tunnel: [_ _ w1196 _] -> w1123
                          tunnel: w1122 -> [_ _ w1194 _]
                          tunnel: w1121 -> [_ _ w1195 _]
                          tunnel: [_ _ w1193 _] -> w1120
                          tunnel: [_ _ w1192 _] -> w1119
                          tunnel: [_ _ w1189 _] -> w1118
                          tunnel: [_ _ w1188 _] -> w1117
                          tunnel: [_ _ w1183 _] -> w1116
                          tunnel: [_ _ w1182 _] -> w1115
                          tunnel: w1114 -> [_ _ w1180 _]
                          tunnel: w1113 -> [_ _ w1181 _]
                          tunnel: [_ _ _ w1706] -> w1112
                          tunnel: [_ _ _ w1709] -> w1111
                          tunnel: [_ _ _ w1708] -> w1110
                          tunnel: [_ _ _ w1705] -> w1109
                          tunnel: [_ _ _ w1703] -> w1108
                          tunnel: w1107 -> [_ _ _ w1702]
                          tunnel: [_ _ _ w1701] -> w1106
                          tunnel: w1105 -> [_ _ _ w1700]
                          tunnel: [_ _ _ w1699] -> w1104
                          tunnel: w1103 -> [_ _ _ w1698]
                          tunnel: [_ _ _ w1697] -> w1102
                          tunnel: w1101 -> [_ _ _ w1696]
                          frame #0 {
                            n324 = Format Into String(format string="SLVLD1,%.3f;", w1169) -> (resulting string=w1170:string)  [unwired: 2 in, 1 out]
                            n325 = local read "LOCKIN1 address"() -> (w1168:refnum<visa-resource-name>)
                            n326 = Concatenate Strings(w1170, "\r") -> (w1166:string)
                            n327 = VISA Write(VISA resource name=w1168, write buffer=w1166) -> ()  [unwired: 1 in, 3 out]
                            n328 = local read "Two Devices ?"() -> (w1167:bool)
                            n329 = case shown="True" w1167 {
                              tunnel: w1166 -> [_ w1174]
                              frame False {
                              }
                              frame True {
                                n330 = local read "LOCKIN2 address"() -> (w1173:refnum<visa-resource-name>)
                                n331 = VISA Write(VISA resource name=w1173, write buffer=w1174) -> ()  [unwired: 1 in, 3 out]
                              }
                            }
                            "Sine voltage T" <- w1169
                          }
                          frame #1 {
                            n332 = local read "System Stablization (s)"() -> (w1175:dbl)
                            n333 = Multiply(x=w1175, y=1000) -> (x*y=w1177:dbl)
                            n334 = Wait (ms)(milliseconds to wait=w1177) -> ()  [unwired: 1 out]
                          }
                          frame #2 {
                            n335 = local read "Sine voltage T"() -> (w1232:dbl)
                            n336 = local read "Two Devices ?"() -> (w1241:bool)
                            n337 = local read "Current measurement?"() -> (w1179:bool)
                            n338 = local read "LOCKIN1 address"() -> (w1211:refnum<visa-resource-name>)
                            n339 = local read "LOCKIN3 address"() -> (w1178:refnum<visa-resource-name>)
                            n340 = case shown="True" w1241 {
                              tunnel: w1232 -> [_ w1380]
                              tunnel: [w1337 w1379] -> w1240
                              tunnel: [w1337 w1378] -> w1239
                              tunnel: [w1337 w1377] -> w1238
                              tunnel: [w1337 w1376] -> w1237
                              tunnel: [w1340 w1375] -> w1216
                              tunnel: [w1342 w1374] -> w1221
                              tunnel: w1220 -> [w1342 w1373]
                              tunnel: w1213 -> [w1340 w1370]
                              tunnel: [w1341 w1372] -> w1219
                              tunnel: w1215 -> [w1341 w1371]
                              tunnel: [w1339 w1369] -> w1217
                              tunnel: w1214 -> [w1339 w1368]
                              tunnel: [w1338 w1367] -> w1218
                              tunnel: w1212 -> [w1338 w1366]
                              tunnel: [w1337 w1352] -> w1199
                              tunnel: [w1337 w1351] -> w1198
                              tunnel: [w1336 w1348] -> w1197
                              tunnel: [w1335 w1347] -> w1196
                              tunnel: w1195 -> [w1336 w1346]
                              tunnel: w1194 -> [w1335 w1343]
                              frame False {
                                w1337 = nan
                              }
                              frame True {
                                n341 = flat-sequence {
                                tunnel: w1380 -> [w1457]
                                tunnel: w1373 -> [w1430]
                                tunnel: [w1455] -> w1429
                                tunnel: [w1448] -> w1428
                                tunnel: [w1449] -> w1427
                                tunnel: [w1446] -> w1426
                                tunnel: [w1449] -> w1425
                                tunnel: [w1449] -> w1424
                                tunnel: [w1449] -> w1423
                                tunnel: [w1449] -> w1422
                                tunnel: [w1448] -> w1421
                                tunnel: [w1447] -> w1420
                                tunnel: [w1446] -> w1419
                                tunnel: [w1445] -> w1418
                                tunnel: ["T Clear Plot 2B"] -> w1417
                                tunnel: ["T Clear Plot 2A"] -> w1416
                                tunnel: [w1436] -> w1415
                                tunnel: [w1438] -> w1414
                                tunnel: [w1437] -> w1413
                                tunnel: [w1442] -> w1412
                                tunnel: [w1441] -> w1411
                                tunnel: w1371 -> [w1432]
                                tunnel: w1368 -> [w1431]
                                tunnel: w1429 -> [w1479]
                                tunnel: [w1479] -> w1410
                                tunnel: w1428 -> [w1478]
                                tunnel: [w1478] -> w1409
                                tunnel: w1427 -> [w1477]
                                tunnel: [w1477] -> w1408
                                tunnel: w1426 -> [w1476]
                                tunnel: [w1476] -> w1407
                                tunnel: w1425 -> [w1475]
                                tunnel: [w1475] -> w1406
                                tunnel: w1424 -> [w1474]
                                tunnel: [w1474] -> w1405
                                tunnel: w1423 -> [w1473]
                                tunnel: [w1473] -> w1404
                                tunnel: w1422 -> [w1472]
                                tunnel: [w1472] -> w1403
                                tunnel: w1421 -> [w1471]
                                tunnel: [w1471] -> w1402
                                tunnel: w1420 -> [w1470]
                                tunnel: [w1470] -> w1401
                                tunnel: w1419 -> [w1469]
                                tunnel: [w1469] -> w1400
                                tunnel: w1418 -> [w1468]
                                tunnel: [w1468] -> w1399
                                tunnel: w1417 -> [w1467]
                                tunnel: [w1467] -> w1398
                                tunnel: w1416 -> [w1466]
                                tunnel: [w1466] -> w1397
                                tunnel: w1415 -> [w1465]
                                tunnel: [w1465] -> w1396
                                tunnel: w1414 -> [w1464]
                                tunnel: [w1464] -> w1395
                                tunnel: w1413 -> [w1463]
                                tunnel: [w1463] -> w1394
                                tunnel: w1412 -> [w1462]
                                tunnel: [w1462] -> w1393
                                tunnel: w1411 -> [w1461]
                                tunnel: [w1461] -> w1392
                                tunnel: w1410 -> [w1487]
                                tunnel: w1409 -> [w1517]
                                tunnel: w1408 -> [w1516]
                                tunnel: w1407 -> [w1515]
                                tunnel: w1406 -> [w1481]
                                tunnel: w1405 -> [w1513]
                                tunnel: w1404 -> [w1511]
                                tunnel: w1403 -> [w1509]
                                tunnel: w1402 -> [w1506]
                                tunnel: w1401 -> [w1505]
                                tunnel: w1400 -> [w1502]
                                tunnel: w1399 -> [w1501]
                                tunnel: w1398 -> [w1480]
                                tunnel: w1366 -> [w1498]
                                tunnel: w1397 -> [w1497]
                                tunnel: w1396 -> [w1493]
                                tunnel: w1395 -> [w1482]
                                tunnel: w1394 -> [w1492]
                                tunnel: w1393 -> [w1489]
                                tunnel: w1392 -> [w1488]
                                tunnel: [w1487] -> w1391
                                tunnel: [w1504] -> w1390
                                tunnel: [w1517] -> w1389
                                tunnel: [w1516] -> w1388
                                tunnel: [w1485] -> w1387
                                tunnel: [w1486] -> w1386
                                tunnel: [w1507] -> w1385
                                tunnel: [w1503] -> w1384
                                tunnel: [w1500] -> w1383
                                tunnel: [w1515] -> w1382
                                tunnel: [w1491] -> w1381
                                tunnel: w1370 -> [w1483]
                                tunnel: [w1482] -> w1354
                                tunnel: [w1481] -> w1349
                                tunnel: [w1480] -> w1344
                                tunnel: w1391 -> [w1532]
                                tunnel: w1390 -> [w1531]
                                tunnel: w1389 -> [w1521]
                                tunnel: w1388 -> [w1530]
                                tunnel: w1387 -> [w1529]
                                tunnel: w1386 -> [w1528]
                                tunnel: w1385 -> [w1527]
                                tunnel: w1384 -> [w1526]
                                tunnel: w1383 -> [w1525]
                                tunnel: w1382 -> [w1524]
                                tunnel: w1381 -> [w1523]
                                tunnel: [w1532] -> w1365
                                tunnel: [w1531] -> w1364
                                tunnel: [w1530] -> w1363
                                tunnel: [w1529] -> w1362
                                tunnel: [w1528] -> w1361
                                tunnel: [w1527] -> w1360
                                tunnel: [w1526] -> w1359
                                tunnel: [w1525] -> w1358
                                tunnel: [w1524] -> w1357
                                tunnel: [w1523] -> w1356
                                tunnel: [w1521] -> w1355
                                tunnel: w1354 -> [w1520]
                                tunnel: [w1520] -> w1353
                                tunnel: [w1519] -> w1350
                                tunnel: w1349 -> [w1519]
                                tunnel: [w1518] -> w1345
                                tunnel: w1344 -> [w1518]
                                tunnel: [w1554] -> w1379
                                tunnel: [w1555] -> w1376
                                tunnel: [w1556] -> w1378
                                tunnel: [w1557] -> w1369
                                tunnel: [w1558] -> w1375
                                tunnel: [w1559] -> w1367
                                tunnel: [w1560] -> w1377
                                tunnel: [w1561] -> w1374
                                tunnel: [w1562] -> w1372
                                tunnel: w1365 -> [w1553]
                                tunnel: w1364 -> [w1562]
                                tunnel: w1363 -> [w1561]
                                tunnel: w1362 -> [w1560]
                                tunnel: w1361 -> [w1538]
                                tunnel: w1360 -> [w1559]
                                tunnel: w1359 -> [w1558]
                                tunnel: w1358 -> [w1557]
                                tunnel: w1357 -> [w1556]
                                tunnel: w1356 -> [w1555]
                                tunnel: w1355 -> [w1554]
                                tunnel: w1353 -> [w1552]
                                tunnel: [w1545] -> w1352
                                tunnel: [w1535] -> w1351
                                tunnel: w1350 -> [w1544]
                                tunnel: [w1543] -> w1348
                                tunnel: [w1542] -> w1347
                                tunnel: w1346 -> [w1541]
                                tunnel: w1345 -> [w1540]
                                tunnel: w1343 -> [w1539]
                                frame #0 {
                                w1438 = u8 1 items=["Channel A", "Channel B"] ("Channel A/B for Parameter1")
                                w1441 = u8 0 items=["Channel A", "Channel B"] ("Channel A/B for Parameter1")
                                n342 = local read "LOCKIN2 address"() -> (w1433:refnum<visa-resource-name>)
                                n343 = Format Into String(0) -> (error out=w1456:errorcluster)  [unwired: 3 in, 1 out]
                                n344 = Format Into String(0) -> (error out=w1439:errorcluster)  [unwired: 3 in, 1 out]
                                n345 = call "OE1022D_Read 1 parameter_mean.vi"("错误输入（无错误）"=w1456, "Parameter"="Parameter 2A", "Channel (0: A)"=w1441, "VISA resource name"=w1433) -> ("error out"=w1442:errorcluster, "Measurement"=w1450:dbl, "VISA resource name out"=w1455:refnum<visa-resource-name>)  [unwired: 5 in]
                                n346 = call "OE1022D_Read 1 parameter_mean.vi"("Parameter 2"="Parameter 2B", "错误输入（无错误）"=w1439, "Channel (0: A)"=w1438, "VISA resource name"=w1433) -> ("error out"=w1436:errorcluster, "Measurement"=w1435:dbl, "VISA resource name out"=w1437:refnum<visa-resource-name>)  [unwired: 5 in]
                                n347 = Multiply(x=w1450, y=1000.0) -> (x*y=w1448:dbl)
                                "Vaa_2(1w)/mV" <- w1448
                                n348 = Multiply(x=w1435, y=1000000.0) -> (x*y=w1446:dbl)
                                "para2B Measurement" <- w1446
                                n349 = Build Array(w1448) -> (w1458:dbl[])
                                n350 = Build Array(w1446) -> (w1452:dbl[])
                                n351 = Select(t=w1458, s="T Clear Plot 2A", f=w1432) -> (s? t:f=w1447:dbl[])
                                n352 = Select(t=w1452, s="T Clear Plot 2B", f=w1431) -> (s? t:f=w1445:dbl[])
                                n353 = Build Array (concatenate)(w1457, w1430) -> (w1449:dbl[])
                                }
                                frame #1 {
                                n354 = Wait (ms)(milliseconds to wait=u32 50) -> ()  [unwired: 1 out]
                                }
                                frame #2 {
                                n355 = Build Array (concatenate)(w1502, w1501) -> (w1500:dbl[])
                                n356 = Build Array (concatenate)(w1506, w1505) -> (w1504:dbl[])
                                n357 = Bundle(w1511, w1504) -> (→"Vaa_2/mV":cluster{dbl[], dbl[]})  [unwired: 1 in]
                                n358 = call "OE1022D_Read 1 parameter_mean.vi"("错误输入（无错误）"=w1489, "Parameter"="Phase 2A", "Channel (0: A)"=w1488, "VISA resource name"=w1487) -> ("error out"=w1486:errorcluster, "Measurement"=w1485:dbl)  [unwired: 5 in, 1 out]
                                "phase Vaa_2" <- w1485
                                n359 = Bundle(w1513, w1500) -> (→"R2B-T":cluster{dbl[], dbl[]})  [unwired: 1 in]
                                n360 = call "OE1022D_Read 1 parameter_mean.vi"("Parameter 2"="Phase 2B", "错误输入（无错误）"=w1493, "Channel (0: A)"=w1482, "VISA resource name"=w1492) -> ("Measurement"=w1491:dbl)  [unwired: 5 in, 2 out]
                                "phase 2B" <- w1491
                                n361 = Build Array(w1485) -> (w1494:dbl[])
                                n362 = Build Array(w1491) -> (w1495:dbl[])
                                n363 = Select(t=w1494, s=w1497, f=w1498) -> (s? t:f=w1496:dbl[])
                                n364 = Select(t=w1495, s=w1480, f=w1483) -> (s? t:f=w1499:dbl[])
                                n365 = Build Array (concatenate)(w1485, w1496) -> (w1507:dbl[])
                                n366 = Build Array (concatenate)(w1491, w1499) -> (w1503:dbl[])
                                n367 = Bundle(w1509, w1507) -> (→"phase Vaa_2":cluster{dbl[], dbl[]})  [unwired: 1 in]
                                n368 = Bundle(w1481, w1503) -> (→"Phase2B-T":cluster{dbl[], dbl[]})  [unwired: 1 in]
                                }
                                frame #3 {
                                n369 = Wait (ms)(milliseconds to wait=u32 50) -> ()  [unwired: 1 out]
                                }
                                frame #4 {
                                n370 = call "OE1022D_Read 1 parameter_mean.vi"("Parameter 2"="Parameter 2B 1", "错误输入（无错误）"=w1538, "Channel (0: A)"=w1552, "VISA resource name"=w1553) -> ("Measurement"=w1536:dbl)  [unwired: 5 in, 2 out]
                                n371 = call "OE1022D_Read 1 parameter_mean.vi"("Parameter 2"="Phase 2B 1", "错误输入（无错误）"=w1538, "Channel (0: A)"=w1552, "VISA resource name"=w1553) -> ("Measurement"=w1545:dbl)  [unwired: 5 in, 2 out]
                                "phase Vab_2" <- w1545
                                n372 = Multiply(x=1000.0, y=w1536) -> (x*y=w1535:dbl)
                                "Vab_2(1w)/mV" <- w1535
                                n373 = Build Array(w1535) -> (w1551:dbl[])
                                n374 = Build Array(w1545) -> (w1548:dbl[])
                                n375 = Select(t=w1551, s=w1540, f=w1539) -> (s? t:f=w1550:dbl[])
                                n376 = Select(t=w1548, s=w1540, f=w1541) -> (s? t:f=w1547:dbl[])
                                n377 = Build Array (concatenate)(w1535, w1550) -> (w1542:dbl[])
                                n378 = Build Array (concatenate)(w1545, w1547) -> (w1543:dbl[])
                                n379 = Bundle(w1544, w1542) -> (→"Vab_2/mV":cluster{dbl[], dbl[]})  [unwired: 1 in]
                                n380 = Bundle(w1544, w1543) -> (→"phase Vab_2":cluster{dbl[], dbl[]})  [unwired: 1 in]
                                }
                                }
                              }
                            }
                            n381 = flat-sequence {
                              tunnel: w1227 -> [w1590]
                              tunnel: w1228 -> [w1589]
                              tunnel: w1226 -> [w1583]
                              tunnel: [w1587] -> w1290
                              tunnel: [w1579] -> w1289
                              tunnel: [w1580] -> w1288
                              tunnel: [w1577] -> w1287
                              tunnel: [w1580] -> w1286
                              tunnel: [w1580] -> w1285
                              tunnel: [w1580] -> w1284
                              tunnel: [w1580] -> w1283
                              tunnel: [w1579] -> w1282
                              tunnel: [w1578] -> w1281
                              tunnel: [w1577] -> w1280
                              tunnel: [w1576] -> w1279
                              tunnel: ["T Clear Plot 1B"] -> w1278
                              tunnel: ["T Clear Plot 1A"] -> w1277
                              tunnel: [w1567] -> w1276
                              tunnel: [w1569] -> w1275
                              tunnel: [w1568] -> w1274
                              tunnel: [w1573] -> w1273
                              tunnel: [w1572] -> w1272
                              tunnel: w1232 -> [w1564]
                              tunnel: w1211 -> [w1563]
                              tunnel: w1290 -> [w1612]
                              tunnel: [w1612] -> w1271
                              tunnel: w1289 -> [w1611]
                              tunnel: [w1611] -> w1270
                              tunnel: w1288 -> [w1610]
                              tunnel: [w1610] -> w1269
                              tunnel: w1287 -> [w1609]
                              tunnel: [w1609] -> w1268
                              tunnel: w1286 -> [w1608]
                              tunnel: [w1608] -> w1267
                              tunnel: w1285 -> [w1607]
                              tunnel: [w1607] -> w1266
                              tunnel: w1284 -> [w1606]
                              tunnel: [w1606] -> w1265
                              tunnel: w1283 -> [w1605]
                              tunnel: [w1605] -> w1264
                              tunnel: w1282 -> [w1604]
                              tunnel: [w1604] -> w1263
                              tunnel: w1281 -> [w1603]
                              tunnel: [w1603] -> w1262
                              tunnel: w1280 -> [w1602]
                              tunnel: [w1602] -> w1261
                              tunnel: w1279 -> [w1601]
                              tunnel: [w1601] -> w1260
                              tunnel: w1278 -> [w1600]
                              tunnel: [w1600] -> w1259
                              tunnel: w1277 -> [w1599]
                              tunnel: [w1599] -> w1258
                              tunnel: w1276 -> [w1598]
                              tunnel: [w1598] -> w1257
                              tunnel: w1275 -> [w1597]
                              tunnel: [w1597] -> w1256
                              tunnel: w1274 -> [w1596]
                              tunnel: [w1596] -> w1255
                              tunnel: w1273 -> [w1595]
                              tunnel: [w1595] -> w1254
                              tunnel: w1272 -> [w1594]
                              tunnel: [w1594] -> w1253
                              tunnel: w1271 -> [w1619]
                              tunnel: w1270 -> [w1650]
                              tunnel: w1269 -> [w1649]
                              tunnel: w1268 -> [w1648]
                              tunnel: w1267 -> [w1647]
                              tunnel: w1266 -> [w1645]
                              tunnel: w1265 -> [w1643]
                              tunnel: w1264 -> [w1614]
                              tunnel: w1263 -> [w1639]
                              tunnel: w1262 -> [w1638]
                              tunnel: w1261 -> [w1635]
                              tunnel: w1260 -> [w1634]
                              tunnel: w1222 -> [w1632]
                              tunnel: w1259 -> [w1613]
                              tunnel: w1223 -> [w1630]
                              tunnel: w1258 -> [w1629]
                              tunnel: w1257 -> [w1625]
                              tunnel: w1256 -> [w1615]
                              tunnel: w1255 -> [w1624]
                              tunnel: w1254 -> [w1621]
                              tunnel: w1253 -> [w1620]
                              tunnel: [w1619] -> w1252
                              tunnel: [w1637] -> w1251
                              tunnel: [w1650] -> w1250
                              tunnel: [w1649] -> w1249
                              tunnel: [w1617] -> w1248
                              tunnel: [w1618] -> w1247
                              tunnel: [w1640] -> w1246
                              tunnel: [w1636] -> w1245
                              tunnel: [w1633] -> w1244
                              tunnel: [w1648] -> w1243
                              tunnel: [w1623] -> w1242
                              tunnel: [w1615] -> w1190
                              tunnel: [w1614] -> w1186
                              tunnel: [w1613] -> w1184
                              tunnel: w1252 -> [w1665]
                              tunnel: w1251 -> [w1664]
                              tunnel: w1250 -> [w1663]
                              tunnel: w1249 -> [w1662]
                              tunnel: w1248 -> [w1661]
                              tunnel: w1247 -> [w1660]
                              tunnel: w1246 -> [w1659]
                              tunnel: w1245 -> [w1658]
                              tunnel: w1244 -> [w1657]
                              tunnel: w1243 -> [w1656]
                              tunnel: w1242 -> [w1655]
                              tunnel: [w1665] -> w1210
                              tunnel: [w1664] -> w1209
                              tunnel: [w1663] -> w1208
                              tunnel: [w1662] -> w1207
                              tunnel: [w1661] -> w1206
                              tunnel: [w1660] -> w1205
                              tunnel: [w1659] -> w1204
                              tunnel: [w1658] -> w1203
                              tunnel: [w1657] -> w1202
                              tunnel: [w1656] -> w1201
                              tunnel: [w1655] -> w1200
                              tunnel: [w1653] -> w1191
                              tunnel: w1190 -> [w1653]
                              tunnel: [w1652] -> w1187
                              tunnel: w1186 -> [w1652]
                              tunnel: [w1651] -> w1185
                              tunnel: w1184 -> [w1651]
                              tunnel: [w1687] -> w1234
                              tunnel: [w1688] -> w1235
                              tunnel: [w1689] -> w1230
                              tunnel: [w1690] -> w1224
                              tunnel: [w1691] -> w1225
                              tunnel: [w1692] -> w1233
                              tunnel: [w1693] -> w1231
                              tunnel: [w1694] -> w1236
                              tunnel: [w1695] -> w1229
                              tunnel: w1210 -> [w1686]
                              tunnel: w1209 -> [w1695]
                              tunnel: w1208 -> [w1694]
                              tunnel: w1207 -> [w1693]
                              tunnel: w1206 -> [w1692]
                              tunnel: w1205 -> [w1685]
                              tunnel: w1204 -> [w1691]
                              tunnel: w1203 -> [w1690]
                              tunnel: w1202 -> [w1689]
                              tunnel: w1201 -> [w1688]
                              tunnel: w1200 -> [w1687]
                              tunnel: w1191 -> [w1684]
                              tunnel: [w1668] -> w1189
                              tunnel: [w1677] -> w1188
                              tunnel: w1187 -> [w1676]
                              tunnel: w1185 -> [w1675]
                              tunnel: [w1674] -> w1183
                              tunnel: [w1673] -> w1182
                              tunnel: w1181 -> [w1672]
                              tunnel: w1180 -> [w1671]
                              frame #0 {
                                w1569 = u8 1 items=["Channel A", "Channel B"] ("Channel A/B for Parameter1")
                                w1572 = u8 0 items=["Channel A", "Channel B"] ("Channel A/B for Parameter1")
                                n382 = Format Into String(0) -> (error out=w1570:errorcluster)  [unwired: 3 in, 1 out]
                                n383 = Format Into String(0) -> (error out=w1588:errorcluster)  [unwired: 3 in, 1 out]
                                n384 = call "OE1022D_Read 1 parameter_mean.vi"("Parameter 2"="Parameter 1B", "错误输入（无错误）"=w1570, "Channel (0: A)"=w1569, "VISA resource name"=w1563) -> ("error out"=w1567:errorcluster, "Measurement"=w1566:dbl, "VISA resource name out"=w1568:refnum<visa-resource-name>)  [unwired: 5 in]
                                n385 = call "OE1022D_Read 1 parameter_mean.vi"("错误输入（无错误）"=w1588, "Parameter"="Parameter 1A", "Channel (0: A)"=w1572, "VISA resource name"=w1563) -> ("error out"=w1573:errorcluster, "Measurement"=w1581:dbl, "VISA resource name out"=w1587:refnum<visa-resource-name>)  [unwired: 5 in]
                                n386 = Multiply(x=w1566, y=1000000.0) -> (x*y=w1577:dbl)
                                "para1B Measurement" <- w1577
                                n387 = Multiply(x=w1581, y=1000.0) -> (x*y=w1579:dbl)
                                "Vaa_1(1w)/mV" <- w1579
                                n388 = Build Array(w1577) -> (w1584:dbl[])
                                n389 = Build Array(w1579) -> (w1591:dbl[])
                                n390 = Build Array (concatenate)(w1564, w1589) -> (w1580:dbl[])
                                n391 = Select(t=w1584, s="T Clear Plot 1B", f=w1583) -> (s? t:f=w1576:dbl[])
                                n392 = Select(t=w1591, s="T Clear Plot 1A", f=w1590) -> (s? t:f=w1578:dbl[])
                              }
                              frame #1 {
                                n393 = Wait (ms)(milliseconds to wait=u32 50) -> ()  [unwired: 1 out]
                              }
                              frame #2 {
                                n394 = Build Array (concatenate)(w1639, w1638) -> (w1637:dbl[])
                                n395 = Build Array (concatenate)(w1635, w1634) -> (w1633:dbl[])
                                n396 = Bundle(w1643, w1637) -> (→"Vaa_1/mV":cluster{dbl[], dbl[]})  [unwired: 1 in]
                                n397 = Bundle(w1645, w1633) -> (→"R1B-T":cluster{dbl[], dbl[]})  [unwired: 1 in]
                                n398 = call "OE1022D_Read 1 parameter_mean.vi"("Parameter 2"="Phase 1B", "错误输入（无错误）"=w1625, "Channel (0: A)"=w1615, "VISA resource name"=w1624) -> ("Measurement"=w1623:dbl)  [unwired: 5 in, 2 out]
                                "phase 1B" <- w1623
                                n399 = Build Array(w1623) -> (w1627:dbl[])
                                n400 = call "OE1022D_Read 1 parameter_mean.vi"("错误输入（无错误）"=w1621, "Parameter"="Phase 1A", "Channel (0: A)"=w1620, "VISA resource name"=w1619) -> ("error out"=w1618:errorcluster, "Measurement"=w1617:dbl)  [unwired: 5 in, 1 out]
                                "phase Vaa_1" <- w1617
                                n401 = Select(t=w1627, s=w1613, f=w1632) -> (s? t:f=w1631:dbl[])
                                n402 = Build Array (concatenate)(w1623, w1631) -> (w1636:dbl[])
                                n403 = Build Array(w1617) -> (w1626:dbl[])
                                n404 = Select(t=w1626, s=w1629, f=w1630) -> (s? t:f=w1628:dbl[])
                                n405 = Bundle(w1647, w1636) -> (→"Phase1B-T":cluster{dbl[], dbl[]})  [unwired: 1 in]
                                n406 = Build Array (concatenate)(w1617, w1628) -> (w1640:dbl[])
                                n407 = Bundle(w1614, w1640) -> (→"phase Vaa_1":cluster{dbl[], dbl[]})  [unwired: 1 in]
                              }
                              frame #3 {
                                n408 = Wait (ms)(milliseconds to wait=u32 50) -> ()  [unwired: 1 out]
                              }
                              frame #4 {
                                n409 = call "OE1022D_Read 1 parameter_mean.vi"("Parameter 2"="Phase 1B 1", "错误输入（无错误）"=w1685, "Channel (0: A)"=w1684, "VISA resource name"=w1686) -> ("Measurement"=w1677:dbl)  [unwired: 5 in, 2 out]
                                "phase Vab_1" <- w1677
                                n410 = call "OE1022D_Read 1 parameter_mean.vi"("Parameter 2"="Parameter 1B 1", "错误输入（无错误）"=w1685, "Channel (0: A)"=w1684, "VISA resource name"=w1686) -> ("Measurement"=w1669:dbl)  [unwired: 5 in, 2 out]
                                n411 = Build Array(w1669) -> (w1682:dbl[])
                                n412 = Build Array(w1677) -> (w1683:dbl[])
                                n413 = Multiply(x=1000.0 ("y"), y=w1669) -> (x*y=w1668:dbl)
                                "Vab_1(1w)/mV" <- w1668
                                n414 = Select(t=w1682, s=w1675, f=w1671) -> (s? t:f=w1678:dbl[])
                                n415 = Select(t=w1683, s=w1675, f=w1672) -> (s? t:f=w1681:dbl[])
                                n416 = Build Array (concatenate)(w1668, w1678) -> (w1673:dbl[])
                                n417 = Build Array (concatenate)(w1677, w1681) -> (w1674:dbl[])
                                n418 = Bundle(w1676, w1673) -> (→"Vab_1/mV":cluster{dbl[], dbl[]})  [unwired: 1 in]
                                n419 = Bundle(w1676, w1674) -> (→"phase Vab_1":cluster{dbl[], dbl[]})  [unwired: 1 in]
                              }
                            }
                            n420 = case shown="True" w1179 {
                              tunnel: w1178 -> [_ w1299]
                              frame False {
                              }
                              frame True {
                                n421 = flat-sequence {
                                tunnel: w1299 -> [w1313]
                                tunnel: [w1312] -> w1297
                                tunnel: [w1311] -> w1296
                                tunnel: [w1310] -> w1293
                                tunnel: [w1309] -> w1291
                                tunnel: [w1322] -> w1298
                                tunnel: w1297 -> [w1322]
                                tunnel: w1296 -> [w1321]
                                tunnel: [w1321] -> w1295
                                tunnel: [w1320] -> w1294
                                tunnel: w1293 -> [w1320]
                                tunnel: [w1319] -> w1292
                                tunnel: w1291 -> [w1319]
                                tunnel: w1298 -> [w1333]
                                tunnel: w1295 -> [w1332]
                                tunnel: w1294 -> [w1331]
                                tunnel: w1292 -> [w1330]
                                frame #0 {
                                w1306 = u16 2 items=["X", "Y", "R", "Theta", "Frequency", "Noise", "Xh1", "Yh1", "Rh1", "Theta h1", "Xh2", "Yh2", "Rh2", "Theta h2"] ("Parameter 2")
                                w1307 = u16 2 items=["X", "Y", "R", "Theta", "Frequency", "Noise", "Xh1", "Yh1", "Rh1", "Theta h1", "Xh2", "Yh2", "Rh2", "Theta h2"] ("Parameter")
                                w1308 = u16 1 items=["Channel A", "Channel B", "ADC"] ("Channel (0: A)")
                                w1314 = u16 0 items=["Channel A", "Channel B", "ADC"] ("Channel (0: A)")
                                n422 = Format Into String(0) -> (error out=w1316:errorcluster)  [unwired: 3 in, 1 out]
                                n423 = Format Into String(0) -> (error out=w1315:errorcluster)  [unwired: 3 in, 1 out]
                                n424 = call "OE1022D_Read 1 parameter_mean.vi"("错误输入（无错误）"=w1316, "Parameter"=w1307, "Channel (0: A)"=w1314, "VISA resource name"=w1313) -> ("error out"=w1311:errorcluster, "Measurement"=w1305:dbl, "VISA resource name out"=w1312:refnum<visa-resource-name>)  [unwired: 5 in]
                                n425 = call "OE1022D_Read 1 parameter_mean.vi"("Parameter 2"=w1306, "错误输入（无错误）"=w1315, "Channel (0: A)"=w1308, "VISA resource name"=w1313) -> ("error out"=w1309:errorcluster, "Measurement"=w1302:dbl, "VISA resource name out"=w1310:refnum<visa-resource-name>)  [unwired: 5 in]
                                n426 = local read "R2(Kohm)"() -> (w1303:dbl)
                                n427 = local read "R1(Kohm)"() -> (w1304:dbl)
                                n428 = Divide(x=w1302, y=w1303) -> (x/y=→"Device2 Current(mA)":dbl)
                                n429 = Divide(x=w1305, y=w1304) -> (x/y=→"Device1 Current(mA)":dbl)
                                }
                                frame #1 {
                                n430 = Wait (ms)(milliseconds to wait=u32 50) -> ()  [unwired: 1 out]
                                }
                                frame #2 {
                                w1326 = u16 3 items=["X", "Y", "R", "Theta", "Frequency", "Noise", "Xh1", "Yh1", "Rh1", "Theta h1", "Xh2", "Yh2", "Rh2", "Theta h2"] ("Parameter 2")
                                w1327 = u16 1 items=["Channel A", "Channel B", "ADC"] ("Channel (0: A)")
                                w1328 = u16 3 items=["X", "Y", "R", "Theta", "Frequency", "Noise", "Xh1", "Yh1", "Rh1", "Theta h1", "Xh2", "Yh2", "Rh2", "Theta h2"] ("Parameter")
                                w1329 = u16 0 items=["Channel A", "Channel B", "ADC"] ("Channel (0: A)")
                                n431 = call "OE1022D_Read 1 parameter_mean.vi"("错误输入（无错误）"=w1332, "Parameter"=w1328, "Channel (0: A)"=w1329, "VISA resource name"=w1333) -> ("Measurement"=→"Device 1 phase":dbl)  [unwired: 5 in, 2 out]
                                n432 = call "OE1022D_Read 1 parameter_mean.vi"("Parameter 2"=w1326, "错误输入（无错误）"=w1330, "Channel (0: A)"=w1327, "VISA resource name"=w1331) -> ("Measurement"=→"Device 2 phase":dbl)  [unwired: 5 in, 2 out]
                                }
                                frame #3 {
                                n433 = Wait (ms)(milliseconds to wait=u32 50) -> ()  [unwired: 1 out]
                                }
                                }
                              }
                            }
                            n434 = local read "Sine voltage T"() -> (w1193:dbl)
                            n435 = local read "Temperature"() -> (w1192:dbl)
                          }
                          frame #3 {
                            n436 = local read "Sine voltage T"() -> (w1714:dbl)
                            n437 = local read "Device1 Current(mA)"() -> (w1729:dbl)
                            n438 = local read "Vaa_1(1w)/mV"() -> (w1730:dbl)
                            n439 = local read "Vaa_2(1w)/mV"() -> (w1728:dbl)
                            n440 = local read "Device2 Current(mA)"() -> (w1727:dbl)
                            n441 = Build Array (concatenate)(w1714, w1707) -> (w1704:dbl[])
                            n442 = Divide(x=w1730, y=w1729) -> (x/y=w1706:dbl)
                            "Ri_1(Ohm)" <- w1706
                            n443 = Divide(x=w1728, y=w1727) -> (x/y=w1705:dbl)
                            "Ri_2(Ohm)" <- w1705
                            n444 = local read "T Clear Plot 2A"() -> (w1711:bool)
                            n445 = local read "T Clear Plot 1A"() -> (w1710:bool)
                            n446 = Build Array(w1705) -> (w1725:dbl[])
                            n447 = Build Array(w1706) -> (w1726:dbl[])
                            n448 = Select(t=w1725, s=w1711, f=w1698) -> (s? t:f=w1715:dbl[])
                            n449 = Select(t=w1726, s=w1710, f=w1702) -> (s? t:f=w1722:dbl[])
                            n450 = Build Array (concatenate)(w1705, w1715) -> (w1699:dbl[])
                            n451 = Build Array (concatenate)(w1706, w1722) -> (w1703:dbl[])
                            n452 = Bundle(w1704, w1699) -> (→"Ri_2":cluster{dbl[], dbl[]})  [unwired: 1 in]
                            n453 = Bundle(w1704, w1703) -> (→"Ri_1":cluster{dbl[], dbl[]})  [unwired: 1 in]
                            n454 = local read "T Clear Plot 1B"() -> (w1713:bool)
                            n455 = local read "T Clear Plot 2B"() -> (w1712:bool)
                            n456 = local read "Device 1 phase"() -> (w1709:dbl)
                            n457 = local read "Device 2 phase"() -> (w1708:dbl)
                            n458 = Build Array(w1709) -> (w1721:dbl[])
                            n459 = Build Array(w1708) -> (w1718:dbl[])
                            n460 = Select(t=w1721, s=w1713, f=w1700) -> (s? t:f=w1719:dbl[])
                            n461 = Select(t=w1718, s=w1712, f=w1696) -> (s? t:f=w1716:dbl[])
                            n462 = Build Array (concatenate)(w1709, w1719) -> (w1701:dbl[])
                            n463 = Build Array (concatenate)(w1708, w1716) -> (w1697:dbl[])
                            n464 = Bundle(w1704, w1701) -> (→"Ri_1 phase":cluster{dbl[], dbl[]})  [unwired: 1 in]
                            n465 = Bundle(w1704, w1697) -> (→"Ri_2 phase":cluster{dbl[], dbl[]})  [unwired: 1 in]
                          }
                        }
                        n466 = case shown="True" w1129 {
                          tunnel: w1119 -> [_ w1775]
                          tunnel: w1152 -> [_ w1780]
                          tunnel: w1153 -> [_ w1781]
                          tunnel: w1150 -> [_ w1779]
                          tunnel: w1151 -> [_ w1778]
                          tunnel: w1120 -> [_ w1777]
                          tunnel: w1157 -> [_ w1774]
                          tunnel: w1156 -> [_ w1773]
                          tunnel: w1155 -> [_ w1772]
                          tunnel: w1154 -> [_ w1771]
                          tunnel: w1120 -> [_ w1770]
                          tunnel: w1128 -> [_ w1768]
                          tunnel: w1127 -> [_ w1769]
                          tunnel: w1126 -> [_ w1767]
                          tunnel: w1125 -> [_ w1766]
                          tunnel: w1118 -> [_ w1765]
                          tunnel: w1117 -> [_ w1764]
                          tunnel: w1112 -> [_ w1763]
                          tunnel: w1111 -> [_ w1762]
                          tunnel: w1110 -> [_ w1761]
                          tunnel: w1109 -> [_ w1760]
                          frame False {
                          }
                          frame True {
                            n467 = Build Array(w1775, w1777, w1781, w1779, w1780, w1778, w1765, w1764, w1763, w1762) -> (w1783:dbl[])
                            n468 = local read "Two Devices ?"() -> (w1776:bool)
                            n469 = call-poly <vilib>:"Write Delimited Spreadsheet.vi"("file path (dialog if empty)"=w1768, "format (%.3f)"="%.10f", "1D data"=w1783, "append to file? (new file:F)"=TRUE) -> ()  [unwired: 10 in, 2 out]
                            n470 = case shown="True" w1776 {
                              tunnel: w1775 -> [_ w1795]
                              tunnel: w1774 -> [_ w1794]
                              tunnel: w1773 -> [_ w1793]
                              tunnel: w1772 -> [_ w1792]
                              tunnel: w1771 -> [_ w1791]
                              tunnel: w1770 -> [_ w1790]
                              tunnel: w1769 -> [_ w1789]
                              tunnel: w1767 -> [_ w1788]
                              tunnel: w1766 -> [_ w1787]
                              tunnel: w1761 -> [_ w1786]
                              tunnel: w1760 -> [_ w1785]
                              frame False {
                              }
                              frame True {
                                n471 = Build Array(w1795, w1790, w1794, w1792, w1793, w1791, w1787, w1788, w1785, w1786) -> (w1797:dbl[])
                                n472 = call-poly <vilib>:"Write Delimited Spreadsheet.vi"("file path (dialog if empty)"=w1789, "format (%.3f)"="%.10f", "1D data"=w1797, "append to file? (new file:F)"=TRUE) -> ()  [unwired: 10 in, 2 out]
                              }
                            }
                          }
                        }
                      }
                    }
                  }
                }
              }
            }
          }
        }
      }
      "Forward" <- FALSE ("Up")
      "Backward" <- FALSE ("Down")
    }
    frame #2 {
      n473 = case shown="True" "Initialization?" {
        tunnel: w1801 -> [w1802 w1805]
        tunnel: w1800 -> [w1803 w1804]
        frame False {
          n474 = Close Reference(reference=w1803, error in (no error)=w1802) -> ()  [unwired: 1 out]
        }
        frame True {
          w1811 = 0 items=["Linear", "NoOvershoot", "Oscillate"] ("Approach")
          w1812 = 0 items=["Persistent", "Driven"] ("Mode")
          w1808 = 0 items=["FastSettle", "NoOvershoot"] ("Approach")
          n475 = call "SetTemperature.vi"("Approach"=w1808, "Rate"=20.0, "Temperature"=1.6, "error in (no error)"=w1805, "Instrument Ref In"=w1804) -> ("error out"=w1816:errorcluster, "Instrument Ref Out"=w1815:refnum<k24>)  [unwired: 2 in, 1 out]
          n476 = call "SetField.vi"("Mode"=w1812, "Approach"=w1811, "Rate"=200.0, "Field"=0.0, "error in (no error)"=w1816, "Instrument Ref In"=w1815) -> ("error out"=w1813:errorcluster, "Instrument Ref Out"=w1814:refnum<k24>)  [unwired: 1 in, 1 out]
          n477 = Close Reference(reference=w1814, error in (no error)=w1813) -> ()  [unwired: 1 out]
        }
      }
    }
  }
  n478 = while {
    tunnel: w24 -> [w1819]
    tunnel: w23 -> [w1818]
    stop <- "?" stop-if-true
    n479 = for {
      N: 10 -> [_]
      shift-right: [w1834] -> _
      shift-left: w1818 -> [w1836]
      tunnel: w1819 -> [w1833]
      tunnel: [w1831] -> _
      tunnel: [w1828] -> w1825
      tunnel: [w1827] -> w1824
      tunnel: [w1829] -> w1822 mode=indexing
      tunnel: [w1830] -> w1823 mode=indexing
      n480 = call "GetTemperature.vi"("error in (no error)"=w1836, "Instrument Ref In"=w1833) -> ("Temperature\nStatus"=w1827:i32, "Temperature"=w1830:dbl, "error out"=w1835:errorcluster, "Instrument Ref Out"=w1832:refnum<k24>)  [unwired: 3 in, 1 out]
      n481 = Wait (ms)(milliseconds to wait=u32 200) -> ()  [unwired: 1 out]
      n482 = call "GetField.vi"("error in (no error)"=w1835, "Instrument Ref In"=w1832) -> ("Field\nStatus"=w1828:i32, "Field"=w1829:dbl, "error out"=w1834:errorcluster, "Instrument Ref Out"=w1831:refnum<k24>)  [unwired: 3 in, 1 out]
    }
    "Field Status 2" <- w1825
    "Temperature Status 2" <- w1824
    n483 = call-poly <vilib>:"Mean.vi"("X"=w1822) -> ("mean"=→"Field":dbl)  [unwired: 1 out]
    n484 = call-poly <vilib>:"Mean.vi"("X"=w1823) -> ("mean"=→"Temperature":dbl)  [unwired: 1 out]
  }
  n485 = local read "Sweep T/F"() -> (w19:bool)
  n486 = case shown="True" w19 {
    tunnel: [w1840 w1862] -> w11
    tunnel: ["Sweep F" "Sweep T"] -> w14
    tunnel: [w1838 w1855] -> w13
    tunnel: [w1839 w1854] -> w12
    frame False {
      n487 = local read "Fixed Temperature"() -> (w1841:dbl)
      n488 = local read "High Value (Oe)"() -> (w1842:dbl)
      n489 = local read "Low Value (Oe)"() -> (w1843:dbl)
      n490 = Format Into String(format string="%.1f", initial string="at", w1841) -> (resulting string=w1840:string)  [unwired: 1 in, 1 out]
      n491 = Format Into String(format string="%d", initial string="from", w1843) -> (resulting string=w1838:string)  [unwired: 1 in, 1 out]
      n492 = Format Into String(format string="%dOe", initial string="to", w1842) -> (resulting string=w1839:string)  [unwired: 1 in, 1 out]
    }
    frame True {
      n493 = local read "Start Value (K)"() -> (w1852:dbl)
      n494 = local read "Fixed Field"() -> (w1851:dbl)
      n495 = local read "End Value (K)"() -> (w1853:dbl)
      n496 = Format Into String(format string="%dK", initial string="to", w1853) -> (resulting string=w1854:string)  [unwired: 1 in, 1 out]
      n497 = Format Into String(format string="%.0fOe", initial string="at", w1851) -> (resulting string=w1862:string)  [unwired: 1 in, 1 out]
      n498 = Format Into String(format string="%d", initial string="from", w1852) -> (resulting string=w1855:string)  [unwired: 1 in, 1 out]
    }
  }
  n499 = Format Into String(format string="%dKohm", "R1(Kohm)") -> (resulting string=w2:string)  [unwired: 2 in, 1 out]
  n500 = local read "Two Devices ?"() -> (w5:bool)
  n501 = case shown="False" w5 {
    tunnel: [w1864 w1866] -> w1
    tunnel: w2 -> [w1864 w1865]
    frame False {
    }
    frame True {
      n502 = Format Into String(format string="%dKohm", initial string=w1865, "R2(Kohm)") -> (resulting string=w1866:string)  [unwired: 1 in, 1 out]
    }
  }
  n503 = local read "A frequency"() -> (w18:dbl)
  n504 = Format Into String(format string="%dHz", initial string="at", w18) -> (resulting string=w10:string)  [unwired: 1 in, 1 out]
  n505 = Format Into String(initial string="path1 (folder + filename)", w14, w13, w12, w11, w10, w1, w9) -> (resulting string=w22:string)  [unwired: 2 in, 1 out]
  n506 = String To Path(string=w22) -> (path=w8:path)
  n507 = Format Into String(initial string="path2 (folder + filename)", w14, w13, w12, w11, w10, w1, w9) -> (resulting string=w21:string)  [unwired: 2 in, 1 out]
  n508 = String To Path(string=w21) -> (path=w7:path)
